vi "Eye tracker_4.2.vi"() -> ()   [LabVIEW 2013]
doc: "made for mouse gaze expt. Version 3"
uses:
  <vilib>/vision/Avi1.llb/AviRefnum.ctl
  <vilib>/vision/Image Controls.llb/IMAQ Image.ctl
  <vilib>/Platform/TimedLoop/XDataNode/timing_clust.ctl
  <vilib>/Platform/TimedLoop/XDataNode/nitl_modes.ctl
  <vilib>/Platform/TimedLoop/XDataNode/wakeup.ctl
  <vilib>/Analysis/baseanly.llb/Mean (DBL).vi
  Eye tracking dependencies/Global 1.vi
  <vilib>/DAQmx/create/channels.llb/DAQmx Create Channel (CO-Pulse Generation-Frequency).vi
  <vilib>/DAQmx/configure/timing.llb/DAQmx Timing (Implicit).vi
  <vilib>/Utility/inputDevices.llb/closeMouse.vi
  <vilib>/Utility/inputDevices.llb/mouseAcquire.vi
  <vilib>/platform/TimedLoop/XDataNode/XDataNode.xnode
  <vilib>/vision/NI_Vision_Development_Module.lvlib
  <vilib>/Platform/TimedLoop/XDataNode/XDNodeRunTimeDep.lvlib
  <vilib>/Analysis/NI_AALBase.lvlib
panel:
  out "Camera ready RTNET":bool
  out "processed frames":i32=12126
  out "param file path":path=path "D:/Satoru/Documents/LabVIEW Data/Saccade suppression project/Eye tracking dependencies/parameters for Eye tracker.txt"
  out "aquired frames":u64=12126
  out "Last Valid Buffer":i32=4318
  in  "duty cylcle of the pulses":dbl=0.5
  out "# of pulses":i32
  out "error IO":errorcluster
  in  "ver":string="3"
  out "saving disk":string="F:\\Eye_tracker_Data3\\"
  out "Info String":string="valid file name"
  out "error flag":errorcluster
  out "eye refnum out":refnum<file>
  in  "Gain offset":dbl min=-10.0 max=10.0 step=0.1
  in  "use % thresh":bool
  in  "Points to show":enum16{"All points", "Fit points"}(ring)
  in  "P Right":i32=237 min=0 max=320 step=5
  in  "P Bottom":i32=187 min=0 max=240 step=5
  in  "P Left":i32=108 min=0 max=320 step=5
  in  "P Top":i32=90 min=0 max=240 step=5
  in  "P Fit type":enum16{"Circle", "Ellipse"}(ring)=enum."Ellipse"
  in  "P Subsampling":i32=2
  in  "P Direction to keep":enum16{"Above", "Below"}(ring)=enum."Below"
  in  "P Threshold":u8=90
  in  "file subname":string="test"
  in  "Eye Y offset(deg)":dbl
  out "calib para":T1={"slope_Rp"=-0.158875, "intercept_Rp"=1.006881, "average_Rp"=0.92245, "slope_Rp0s"=-0.125099, "intercept_Rp0s"=1.099699, "average_Rp0s"=1.033217, "Y correction (pixel,P-CR Y)"=-9.268179}
  out "average_Rp0s":dbl=1.033217 format="%0.2f"
  out "R-squared_Rp0s":dbl=0.136529 format="%0.2f"
  out "intercept_Rp0s":dbl=1.099699 format="%0.2f"
  out "slope_Rp0s":dbl=-0.125099 format="%0.2f"
  out "slope_Rp":dbl=-0.158875 format="%0.2f"
  out "intercept_Rp":dbl=1.006881 format="%0.2f"
  out "R-squared_Rp":dbl=0.186582 format="%0.2f"
  out "average_Rp":dbl=0.92245 format="%0.2f"
  out "Rp0s":dbl[](array[numeric])=[1.0039530251172462, 0.99092677428564, 0.9947124694308508, 0.91502715314781, 0.9309803093450226, 0.9217648889080421, 0.9419782161135387, 0.41862170883477745, 1.0171231935751164, 1.0055084222134438, 0.9877063931309743, 0.9965106512655807, 1.0044842853477027, 1.0208232955492513, 0.3759308138742579, 0.9922053798543352, 0.9837769455073831, 1.0906382792092393, 1.0404579348655312, 1.0380768060657999, 0.7651629263639542, 0.9942213575350989, 0.9175234235218281, 0.9692162880521514, 0.9785182040001951, 0.9925018928857751, 1.0118623499027188, 0.987701680921089, 0.9820974709148313, 0.9777636459363701, 0.996026118758922, 0.9978612450714602, 1.0057534405553457, 1.002758388150481, 1.0281377557537945, 0.9995175172174519, 1.0172882695205345, 0.9728176754414147, 0.9567541016151462, 0.9881969134208142, 0.9994817859973143, 0.937125056422465, 0.9712908288207139, 1.0043446841247143, 1.2083670139927292, 1.510991890895332, 0.9895877539387384, 1.0042622767782914, 1.019202247794033, 0.977553264609903, 0.994725760374644, 1.019400802873885, 1.334253570427072, 0.9352478253803249, 0.956119013286909, 0.9758901683111171, 0.9779851768159086, 1.0516777655254512, 0.778039137219539, 1.1531230503845833, 1.0046625233826771, 0.9901398342766586, 1.011163664944152, 0.9938975966142147, 0.6154945551221118, 1.0077384474948252, 0.9896589896861816, 0.9972982423508683, 0.6853268629838346, 0.9658925865003825, 0.9626225998838313, 1.0096874472713344, 1.0358515198060945, 1.0544730519999652, 1.0617108224193677, 1.0142433944577367, 1.0418591984643595, 1.019211033782866, 1.0450176088988177, 1.0464926937167767, 1.1283816882695141, 1.030013176033189, 1.0427307654804812, 1.0441392816021982, 1.0538940244491395, 1.0462542279584326, 1.0781380078152705, 0.9990695213505404, 1.0272273014788156, 1.0262064169141834, 0.4857640606302865, 1.5639567502437777, 0.8687438257698011, 0.9864671983220689, 1.0593826663266908, 1.077023826126648, 1.0593759395811841, 1.0778741239177942]
  out "Diameters":dbl[](array[numeric])=[0.4171123023396653, 0.41706153689125236, 0.44082198235372194, 0.5954203122934263, 0.5513970359660245, 0.4888545273412629, 0.4723633211125596, 0.6187264429619335, 0.4791395781041599, 0.47868971473218613, 0.4607929067005807, 0.4175941622450629, 0.4072745719163012, 0.40955932983558824, 0.4735723248260562, 0.44999914869512314, 0.495476167758055, 0.5199527975917938, 0.4888346729487987, 0.4452820985792543, 0.6301036042248925, 0.4469040074392198, 0.3829612562912073, 0.4107677254295738, 0.40124095377797425, 0.383476616742587, 0.3832933211731289, 0.43509323930099303, 0.4004105804184655, 0.4216375686518822, 0.45690852528210607, 0.4082721732536112, 0.45028685912440625, 0.3918383679660448, 0.3652661041731884, 0.3475647461563056, 0.4095548614857446, 0.6482149714983727, 0.5034836724573097, 0.4455174223358519, 0.4486765714162201, 0.5064000813046842, 0.49521426028650833, 0.44577031309198606, 0.45147318540007164, 0.4761169863513808, 0.43800992027731955, 0.4015153245290642, 0.39091576046128906, 0.379195166874867, 0.38301812558069126, 0.35970454061703483, 0.42529628662735336, 0.42838925138004624, 0.3826964399461055, 0.3606217495513988, 0.3686694627564316, 0.36628712709457356, 0.5276402515437981, 0.5027800799946363, 0.5917418979942912, 0.4405882646486038, 0.3855160638859669, 0.3520620038697737, 0.4917921769667696, 0.39313264413588306, 0.3962868259759099, 0.3692702539594129, 0.43066029115997034, 0.5289298666466735, 0.4857116713496977, 0.3808981023756301, 0.37251109381109737, 0.3648554945721928, 0.3719954884814041, 0.3714007266142857, 0.34155839352729517, 0.3379878486536885, 0.34158014089555133, 0.3883397541343963, 0.3779925489446427, 0.3350578969183736, 0.3364315822035769, 0.32799683082239195, 0.30857349620419, 0.3354342336706663, 0.2996572825051776, 0.3530772896636659, 0.31517664347717034, 0.3170963264045597, 0.44637289830791427, 0.37272436153500477, 0.3543878411074852, 0.46493263060229995, 0.31309427627625497, 0.39133764775033814, 0.3896143560981249, 0.34679282192506145]
  out "Rp":dbl[](array[numeric])=[0.939777828488882, 0.9243782721008702, 0.9247867300831337, 0.8546428244499522, 0.8722515142500874, 0.8599558310217699, 0.8821886686394919, 0.27768529551706517, 0.9621621967506099, 0.9489706433656064, 0.9286039576834555, 0.9360718380299038, 0.9427832164989408, 0.9580355580333006, 0.18594170348233657, 0.9408721482456565, 0.9298677620512195, 1.03645888355633, 0.9826129548661878, 0.9795606095219592, 0.6946292066688117, 0.9414788639375723, 0.8576339811674867, 0.9130407361980429, 0.9228386688426881, 0.9350370985090772, 0.95317668634537, 0.9265514452452699, 0.9183790967298439, 0.9138737325811144, 0.9315397662213876, 0.9334204076293418, 0.9423909994254046, 0.9378626398245973, 0.9648383077501701, 0.9338531100959763, 0.9531838316474268, 0.9307945475016182, 0.8970066818718861, 0.9280567210488938, 0.9374342077923953, 0.8791518280424994, 0.9236246067129958, 0.9511138467128057, 1.1666245999199012, 1.4802034620448514, 0.9412071610357354, 0.95348691386894, 0.9657397985521751, 0.9190931489538748, 0.9348033445576653, 0.9599667294264533, 1.2900914874489557, 0.8774362961435918, 0.896842734172207, 0.9171822481686075, 0.9164350407661369, 0.9903031524940573, 0.7074385526832087, 1.1067447532230492, 0.9610074838402222, 0.943528766665827, 0.958930447804304, 0.9386499872173812, 0.5144779715413748, 0.9513120067327815, 0.9306395174738417, 0.9365203104014679, 0.5902231328371776, 0.9026704048492892, 0.8933039465724875, 0.9465112185353972, 0.9722657096813544, 0.9903344550575592, 0.9978061383235594, 0.9432972456213076, 0.9754521620179915, 0.9527832237284578, 0.979250668089585, 0.9810855558397411, 1.084116178214518, 0.9823792672041992, 0.9927448850260591, 0.9912403488728432, 0.9999505174357944, 0.9893853300714827, 1.0226328706112693, 0.9508934971805839, 0.9756310457714327, 0.9724214165590328, 0.3641279840331179, 1.5306845012262937, 0.802628109680344, 0.9346469119852467, 1.00312473762936, 1.0121118529364288, 0.994327011204879, 1.0147111135607931]
  out "calib data":dbl[][][](array[numeric])
  out "Frame Rate":cluster{i32, "camera FR":i32}={200, "camera FR"=200}
  out "Frame Buffers Out":T2[](array[typedef])=[refnum, refnum, refnum, refnum, refnum, refnum, refnum, refnum, refnum, refnum, refnum, refnum, refnum, refnum, refnum, refnum, refnum, refnum, refnum, refnum, refnum, refnum, refnum, refnum, refnum, refnum, refnum, refnum, refnum, refnum, refnum, refnum, refnum, refnum, refnum, refnum, refnum, refnum, refnum, refnum, refnum, refnum, refnum, refnum, refnum, refnum, refnum, refnum, refnum, refnum, refnum, refnum, refnum, refnum, refnum, refnum, refnum, refnum, refnum, refnum, refnum, refnum, refnum, refnum, refnum, refnum, refnum, refnum, refnum, refnum, refnum, refnum, refnum, refnum, refnum, refnum, refnum, refnum, refnum, refnum, refnum, refnum, refnum, refnum, refnum, refnum, refnum, refnum, refnum, refnum, refnum, refnum, refnum, refnum, refnum, refnum, refnum, refnum, refnum, refnum, refnum, refnum, refnum, refnum, refnum, refnum, refnum, refnum, refnum, refnum, refnum, refnum, refnum, refnum, refnum, refnum, refnum, refnum, refnum, refnum, refnum, refnum, refnum, refnum, refnum, refnum, refnum, refnum, refnum, refnum, refnum, refnum, refnum, refnum, refnum, refnum, refnum, refnum, refnum, refnum, refnum, refnum, refnum, refnum, refnum, refnum, refnum, refnum, refnum, refnum, refnum, refnum, refnum, refnum, refnum, refnum, refnum, refnum, refnum, refnum, refnum, refnum, refnum, refnum, refnum, refnum, refnum, refnum, refnum, refnum, refnum, refnum, refnum, refnum, refnum, refnum, refnum, refnum, refnum, refnum, refnum, refnum, refnum, refnum, refnum, refnum, refnum, refnum, refnum, refnum, refnum, refnum, refnum, refnum, refnum, refnum, refnum, refnum, refnum, refnum, refnum, refnum, refnum, refnum, refnum, refnum, refnum, refnum, refnum, refnum, refnum, refnum, refnum, refnum, refnum, refnum, refnum, refnum, refnum, refnum, refnum, refnum, refnum, refnum, refnum, refnum, refnum, refnum, refnum, refnum, refnum, refnum, refnum, refnum, refnum, refnum, refnum, refnum, refnum, refnum, refnum, refnum, refnum, refnum, "LL Ring num 244", "LL Ring num 245", "LL Ring num 246", "LL Ring num 247", "LL Ring num 248", "LL Ring num 249", "LL Ring num 250", "LL Ring num 251", "LL Ring num 252", "LL Ring num 253", "LL Ring num 254", "LL Ring num 255", "LL Ring num 256", "LL Ring num 257", "LL Ring num 258", "LL Ring num 259", "LL Ring num 260", "LL Ring num 261", "LL Ring num 262", "LL Ring num 263", "LL Ring num 264", "LL Ring num 265", "LL Ring num 266", "LL Ring num 267", "LL Ring num 268", "LL Ring num 269", "LL Ring num 270", "LL Ring num 271", "LL Ring num 272", "LL Ring num 273", "LL Ring num 274", "LL Ring num 275", "LL Ring num 276", "LL Ring num 277", "LL Ring num 278", "LL Ring num 279", "LL Ring num 280", "LL Ring num 281", "LL Ring num 282", "LL Ring num 283", "LL Ring num 284", "LL Ring num 285", "LL Ring num 286", "LL Ring num 287", "LL Ring num 288", "LL Ring num 289", "LL Ring num 290", "LL Ring num 291", "LL Ring num 292", "LL Ring num 293", "LL Ring num 294", "LL Ring num 295", "LL Ring num 296", "LL Ring num 297", "LL Ring num 298", "LL Ring num 299", "LL Ring num 300", "LL Ring num 301", "LL Ring num 302", "LL Ring num 303", "LL Ring num 304", "LL Ring num 305", "LL Ring num 306", "LL Ring num 307", "LL Ring num 308", "LL Ring num 309", "LL Ring num 310", "LL Ring num 311", "LL Ring num 312", "LL Ring num 313", "LL Ring num 314", "LL Ring num 315", "LL Ring num 316", "LL Ring num 317", "LL Ring num 318", "LL Ring num 319", "LL Ring num 320", "LL Ring num 321", "LL Ring num 322", "LL Ring num 323", "LL Ring num 324", "LL Ring num 325", "LL Ring num 326", "LL Ring num 327", "LL Ring num 328", "LL Ring num 329", "LL Ring num 330", "LL Ring num 331", "LL Ring num 332", "LL Ring num 333", "LL Ring num 334", "LL Ring num 335", "LL Ring num 336", "LL Ring num 337", "LL Ring num 338", "LL Ring num 339", "LL Ring num 340", "LL Ring num 341", "LL Ring num 342", "LL Ring num 343", "LL Ring num 344", "LL Ring num 345", "LL Ring num 346", "LL Ring num 347", "LL Ring num 348", "LL Ring num 349", "LL Ring num 350", "LL Ring num 351", "LL Ring num 352", "LL Ring num 353", "LL Ring num 354", "LL Ring num 355", "LL Ring num 356", "LL Ring num 357", "LL Ring num 358", "LL Ring num 359", "LL Ring num 360", "LL Ring num 361", "LL Ring num 362", "LL Ring num 363", "LL Ring num 364", "LL Ring num 365", "LL Ring num 366", "LL Ring num 367", "LL Ring num 368", "LL Ring num 369", "LL Ring num 370", "LL Ring num 371", "LL Ring num 372", "LL Ring num 373", "LL Ring num 374", "LL Ring num 375", "LL Ring num 376", "LL Ring num 377", "LL Ring num 378", "LL Ring num 379", "LL Ring num 380", "LL Ring num 381", "LL Ring num 382", "LL Ring num 383", "LL Ring num 384", "LL Ring num 385", "LL Ring num 386", "LL Ring num 387", "LL Ring num 388", "LL Ring num 389", "LL Ring num 390", "LL Ring num 391", "LL Ring num 392", "LL Ring num 393", "LL Ring num 394", "LL Ring num 395", "LL Ring num 396", "LL Ring num 397", "LL Ring num 398", "LL Ring num 399", "LL Ring num 400", "LL Ring num 401", "LL Ring num 402", "LL Ring num 403", "LL Ring num 404", "LL Ring num 405", "LL Ring num 406", "LL Ring num 407", "LL Ring num 408", "LL Ring num 409", "LL Ring num 410", "LL Ring num 411", "LL Ring num 412", "LL Ring num 413", "LL Ring num 414", "LL Ring num 415", "LL Ring num 416", "LL Ring num 417", "LL Ring num 418", "LL Ring num 419", "LL Ring num 420", "LL Ring num 421", "LL Ring num 422", "LL Ring num 423", "LL Ring num 424", "LL Ring num 425", "LL Ring num 426", "LL Ring num 427", "LL Ring num 428", "LL Ring num 429", "LL Ring num 430", "LL Ring num 431", "LL Ring num 432", "LL Ring num 433", "LL Ring num 434", "LL Ring num 435", "LL Ring num 436", "LL Ring num 437", "LL Ring num 438", "LL Ring num 439", "LL Ring num 440", "LL Ring num 441", "LL Ring num 442", "LL Ring num 443", "LL Ring num 444", "LL Ring num 445", "LL Ring num 446", "LL Ring num 447", "LL Ring num 448", "LL Ring num 449", "LL Ring num 450", "LL Ring num 451", "LL Ring num 452", "LL Ring num 453", "LL Ring num 454", "LL Ring num 455", "LL Ring num 456", "LL Ring num 457", "LL Ring num 458", "LL Ring num 459", "LL Ring num 460", "LL Ring num 461", "LL Ring num 462", "LL Ring num 463", "LL Ring num 464", "LL Ring num 465", "LL Ring num 466", "LL Ring num 467", "LL Ring num 468", "LL Ring num 469", "LL Ring num 470", "LL Ring num 471", "LL Ring num 472", "LL Ring num 473", "LL Ring num 474", "LL Ring num 475", "LL Ring num 476", "LL Ring num 477", "LL Ring num 478", "LL Ring num 479", "LL Ring num 480", "LL Ring num 481", "LL Ring num 482", "LL Ring num 483", "LL Ring num 484", "LL Ring num 485", "LL Ring num 486", "LL Ring num 487", "LL Ring num 488", "LL Ring num 489", "LL Ring num 490", "LL Ring num 491", "LL Ring num 492", "LL Ring num 493", "LL Ring num 494", "LL Ring num 495", "LL Ring num 496", "LL Ring num 497", "LL Ring num 498", "LL Ring num 499"]
  out "Avi Refnum":T3
  in  "tasks":T4(tab)
  in  "Disp trace Divisor":i32=25 min=1 step=1
  in  "Disp Frame Divisor":i32=25 min=1 step=1
  in  "Save Movie? 2":bool
  in  "Cam FR (f/s)":i32=200 min=2 max=3000 step=1
  in  "Save Frame Divisor":i32=1 min=1 step=1
  in  "Gain (dB)":dbl(slide)=26.8032 min=6.0 max=39.5 step=0.0352 scale=6.0..40.0
  in  "Pixel value offset":cluster{"Ch 1":u8, "Ch 2":u8} {"Ch 2" step=1; "Ch 1" step=1}
  in  "Zoom":i32=2 min=1 step=1
  in  "Region of interest":i32[](array[numeric])
  in  "resolution":cluster{"width":u16, "height":u16}={"width"=320, "height"=240}
  out "Image Histogram":T5(graph)={"Starting Value"=0.0, "Incremental Value"=1.0, "Histogram"=[0, 0, 0, 0, 0, 0, 0, 0, 0, 0, 0, 0, 0, 0, 0, 0, 0, 0, 0, 0, 0, 0, 0, 0, 0, 0, 0, 0, 0, 0, 0, 0, 0, 0, 0, 0, 0, 0, 1, 0, 2, 1, 2, 0, 2, 5, 8, 9, 18, 23, 34, 49, 54, 74, 101, 111, 113, 126, 172, 183, 141, 158, 148, 135, 127, 122, 91, 85, 65, 46, 46, 43, 40, 39, 43, 48, 65, 47, 64, 67, 91, 83, 84, 79, 92, 128, 112, 149, 146, 162, 194, 158, 185, 221, 216, 248, 195, 235, 264, 290, 305, 364, 334, 349, 350, 401, 397, 418, 398, 463, 458, 492, 462, 444, 529, 514, 538, 509, 522, 584, 568, 532, 583, 588, 592, 524, 582, 558, 618, 623, 630, 632, 648, 649, 663, 659, 686, 600, 694, 632, 583, 621, 634, 597, 560, 534, 594, 608, 627, 668, 723, 649, 721, 661, 767, 727, 738, 779, 744, 716, 773, 730, 722, 722, 744, 741, 717, 726, 734, 718, 658, 672, 715, 706, 700, 651, 599, 659, 582, 573, 572, 475, 531, 552, 484, 442, 423, 410, 432, 389, 400, 410, 402, 399, 387, 426, 425, 434, 407, 413, 438, 473, 437, 439, 395, 440, 395, 382, 389, 401, 409, 339, 342, 316, 301, 326, 265, 255, 273, 254, 261, 232, 228, 217, 234, 230, 169, 192, 206, 164, 201, 170, 181, 178, 136, 161, 156, 156, 140, 132, 116, 121, 112, 106, 94, 88, 109, 79, 85, 75, 82, 94, 55, 101, 99, 1333]}
  out "file or folder exists? 4":bool
  in  "stop free run":bool
  in  "counter":tag="Dev1/ctr0"
  in  "Cam FR (f/s) 2":i32=200 min=2 max=3000 step=1
  out "frames captured":u64=39600
  in  "Change pupil size?":bool=TRUE
  in  "1D or 2D cal?":bool=TRUE
  in  "L/R?":bool=TRUE
  in  "clip time(s)":sgl=1.0
  in  "stop calib":bool
  out "counter finished":sgl=88.0 format="%#.1f"
  out "Y correction (pixel,P-CR Y)":dbl=-9.268179
  out "frames/clip":i32=200
  out "conversion factor":cluster{"x":dbl, "y":dbl}={"x"=0.01556420233463035, "y"=0.015463917525773196} {"y" format="%#_9g"; "x" format="%#_9g"}
  out "Rp vs Pupil":cluster{dbl[], dbl[]}[](graph)=[{[0.4171123023396653, 0.41706153689125236, 0.44082198235372194, 0.5954203122934263, 0.5513970359660245, 0.4723633211125596, 0.4607929067005807, 0.4175941622450629, 0.4072745719163012, 0.40955932983558824, 0.44999914869512314, 0.495476167758055, 0.4469040074392198, 0.4107677254295738, 0.40124095377797425, 0.383476616742587, 0.3832933211731289, 0.43509323930099303, 0.4004105804184655, 0.4216375686518822, 0.45690852528210607, 0.4082721732536112, 0.45028685912440625, 0.3918383679660448, 0.3652661041731884, 0.4095548614857446, 0.5034836724573097, 0.4455174223358519, 0.4486765714162201, 0.5064000813046842, 0.49521426028650833, 0.44577031309198606, 0.43800992027731955, 0.4015153245290642, 0.39091576046128906, 0.38301812558069126, 0.35970454061703483, 0.36628712709457356, 0.4405882646486038, 0.3855160638859669, 0.3520620038697737, 0.39313264413588306, 0.3962868259759099, 0.3692702539594129, 0.5289298666466735, 0.4857116713496977, 0.3808981023756301, 0.37251109381109737, 0.3648554945721928, 0.3714007266142857, 0.34155839352729517, 0.3379878486536885, 0.34158014089555133, 0.3883397541343963, 0.3350578969183736, 0.3364315822035769, 0.32799683082239195, 0.30857349620419, 0.3354342336706663, 0.2996572825051776, 0.3530772896636659, 0.31517664347717034, 0.3170963264045597, 0.46493263060229995, 0.31309427627625497], [0.939777828488882, 0.9243782721008702, 0.9247867300831337, 0.8546428244499522, 0.8722515142500874, 0.8821886686394919, 0.9286039576834555, 0.9360718380299038, 0.9427832164989408, 0.9580355580333006, 0.9408721482456565, 0.9298677620512195, 0.9414788639375723, 0.9130407361980429, 0.9228386688426881, 0.9350370985090772, 0.95317668634537, 0.9265514452452699, 0.9183790967298439, 0.9138737325811144, 0.9315397662213876, 0.9334204076293418, 0.9423909994254046, 0.9378626398245973, 0.9648383077501701, 0.9531838316474268, 0.8970066818718861, 0.9280567210488938, 0.9374342077923953, 0.8791518280424994, 0.9236246067129958, 0.9511138467128057, 0.9412071610357354, 0.95348691386894, 0.9657397985521751, 0.9348033445576653, 0.9599667294264533, 0.9903031524940573, 0.943528766665827, 0.958930447804304, 0.9386499872173812, 0.9513120067327815, 0.9306395174738417, 0.9365203104014679, 0.9026704048492892, 0.8933039465724875, 0.9465112185353972, 0.9722657096813544, 0.9903344550575592, 0.9432972456213076, 0.9754521620179915, 0.9527832237284578, 0.979250668089585, 0.9810855558397411, 0.9823792672041992, 0.9927448850260591, 0.9912403488728432, 0.9999505174357944, 0.9893853300714827, 1.0226328706112693, 0.9508934971805839, 0.9756310457714327, 0.9724214165590328, 0.9346469119852467, 1.00312473762936]}, {[0.4171123023396653, 0.41706153689125236, 0.44082198235372194, 0.5954203122934263, 0.5513970359660245, 0.4723633211125596, 0.4607929067005807, 0.4175941622450629, 0.4072745719163012, 0.40955932983558824, 0.44999914869512314, 0.495476167758055, 0.4469040074392198, 0.4107677254295738, 0.40124095377797425, 0.383476616742587, 0.3832933211731289, 0.43509323930099303, 0.4004105804184655, 0.4216375686518822, 0.45690852528210607, 0.4082721732536112, 0.45028685912440625, 0.3918383679660448, 0.3652661041731884, 0.4095548614857446, 0.5034836724573097, 0.4455174223358519, 0.4486765714162201, 0.5064000813046842, 0.49521426028650833, 0.44577031309198606, 0.43800992027731955, 0.4015153245290642, 0.39091576046128906, 0.38301812558069126, 0.35970454061703483, 0.36628712709457356, 0.4405882646486038, 0.3855160638859669, 0.3520620038697737, 0.39313264413588306, 0.3962868259759099, 0.3692702539594129, 0.5289298666466735, 0.4857116713496977, 0.3808981023756301, 0.37251109381109737, 0.3648554945721928, 0.3714007266142857, 0.34155839352729517, 0.3379878486536885, 0.34158014089555133, 0.3883397541343963, 0.3350578969183736, 0.3364315822035769, 0.32799683082239195, 0.30857349620419, 0.3354342336706663, 0.2996572825051776, 0.3530772896636659, 0.31517664347717034, 0.3170963264045597, 0.46493263060229995, 0.31309427627625497], [0.9398873587415357, 0.9399102647487777, 0.929189253650656, 0.8594325475462748, 0.87929640215402, 0.9149574058758638, 0.9201781220243312, 0.9396699375066659, 0.9443262661355832, 0.9432953546971639, 0.9250484010580191, 0.9045285994889237, 0.9264449676252247, 0.9427501114442752, 0.9470487103391233, 0.9550642020860263, 0.9551469073466453, 0.9317741343905228, 0.9474233852170393, 0.9378455018061569, 0.9219308036549254, 0.9438761358959925, 0.9249185825026279, 0.9512912750250406, 0.9632810138317232, 0.9432973708726745, 0.9009155129041384, 0.927070612220364, 0.9256451645196992, 0.8995995926420899, 0.9046467754260529, 0.9269565047383553, 0.930458091340477, 0.9469249108138964, 0.9517075671064884, 0.955271079050637, 0.9657904610852527, 0.9628203154795438, 0.9292947100114956, 0.9541439779474367, 0.9692388695511045, 0.9507072813788446, 0.9492840749593423, 0.9614742912109515, 0.8894338708305484, 0.9089344627765849, 0.956227660119188, 0.9600119836093526, 0.9634662860353198, 0.9605129952195437, 0.9739782303189793, 0.9755893049630445, 0.9739684176335733, 0.9528698934805067, 0.9769113359460448, 0.9762915119107062, 0.9800973775587395, 0.9888614298292744, 0.97674152808178, 0.9928845373156776, 0.9687807598628296, 0.9858820069347005, 0.9850158219129624, 0.918310226661696, 0.9868215971417378]}, {[0.37272436153500477, 0.44637289830791427, 0.43066029115997034, 0.4917921769667696, 0.42529628662735336, 0.4761169863513808, 0.4735723248260562, 0.6187264429619335, 0.3543878411074852, 0.3779925489446427, 0.5027800799946363, 0.5276402515437981, 0.45147318540007164, 0.6301036042248925, 0.5199527975917938, 0.39133764775033814, 0.5917418979942912, 0.42838925138004624, 0.3829612562912073, 0.4888346729487987, 0.3826964399461055, 0.6482149714983727, 0.4888545273412629, 0.3686694627564316, 0.3606217495513988, 0.4452820985792543, 0.4791395781041599, 0.34679282192506145, 0.3896143560981249, 0.3719954884814041, 0.379195166874867, 0.3475647461563056, 0.47868971473218613], [1.5306845012262937, 0.3641279840331179, 0.5902231328371776, 0.5144779715413748, 1.2900914874489557, 1.4802034620448514, 0.18594170348233657, 0.27768529551706517, 0.802628109680344, 1.084116178214518, 1.1067447532230492, 0.7074385526832087, 1.1666245999199012, 0.6946292066688117, 1.03645888355633, 1.0121118529364288, 0.9610074838402222, 0.8774362961435918, 0.8576339811674867, 0.9826129548661878, 0.896842734172207, 0.9307945475016182, 0.8599558310217699, 0.9164350407661369, 0.9171822481686075, 0.9795606095219592, 0.9621621967506099, 1.0147111135607931, 0.994327011204879, 0.9978061383235594, 0.9190931489538748, 0.9338531100959763, 0.9489706433656064]}]
  out "Rp0s vs Pupil":cluster{dbl[], dbl[]}[](graph)=[{[0.4171123023396653, 0.41706153689125236, 0.44082198235372194, 0.5954203122934263, 0.5513970359660245, 0.4607929067005807, 0.4175941622450629, 0.4072745719163012, 0.40955932983558824, 0.44999914869512314, 0.495476167758055, 0.4469040074392198, 0.40124095377797425, 0.383476616742587, 0.3832933211731289, 0.43509323930099303, 0.4004105804184655, 0.4216375686518822, 0.45690852528210607, 0.4082721732536112, 0.45028685912440625, 0.3918383679660448, 0.3652661041731884, 0.3475647461563056, 0.4095548614857446, 0.5034836724573097, 0.4455174223358519, 0.4486765714162201, 0.5064000813046842, 0.49521426028650833, 0.44577031309198606, 0.43800992027731955, 0.4015153245290642, 0.39091576046128906, 0.38301812558069126, 0.35970454061703483, 0.4405882646486038, 0.3855160638859669, 0.39313264413588306, 0.3962868259759099, 0.3692702539594129, 0.5289298666466735, 0.4857116713496977, 0.3808981023756301, 0.37251109381109737, 0.3714007266142857, 0.34155839352729517, 0.3379878486536885, 0.34158014089555133, 0.3350578969183736, 0.3364315822035769, 0.32799683082239195, 0.30857349620419, 0.3354342336706663, 0.3530772896636659, 0.31517664347717034, 0.3170963264045597, 0.46493263060229995, 0.31309427627625497], [1.0039530251172462, 0.99092677428564, 0.9947124694308508, 0.91502715314781, 0.9309803093450226, 0.9877063931309743, 0.9965106512655807, 1.0044842853477027, 1.0208232955492513, 0.9922053798543352, 0.9837769455073831, 0.9942213575350989, 0.9785182040001951, 0.9925018928857751, 1.0118623499027188, 0.987701680921089, 0.9820974709148313, 0.9777636459363701, 0.996026118758922, 0.9978612450714602, 1.0057534405553457, 1.002758388150481, 1.0281377557537945, 0.9995175172174519, 1.0172882695205345, 0.9567541016151462, 0.9881969134208142, 0.9994817859973143, 0.937125056422465, 0.9712908288207139, 1.0043446841247143, 0.9895877539387384, 1.0042622767782914, 1.019202247794033, 0.994725760374644, 1.019400802873885, 0.9901398342766586, 1.011163664944152, 1.0077384474948252, 0.9896589896861816, 0.9972982423508683, 0.9658925865003825, 0.9626225998838313, 1.0096874472713344, 1.0358515198060945, 1.0142433944577367, 1.0418591984643595, 1.019211033782866, 1.0450176088988177, 1.030013176033189, 1.0427307654804812, 1.0441392816021982, 1.0538940244491395, 1.0462542279584326, 0.9990695213505404, 1.0272273014788156, 1.0262064169141834, 0.9864671983220689, 1.0593826663266908]}, {[0.4171123023396653, 0.41706153689125236, 0.44082198235372194, 0.5954203122934263, 0.5513970359660245, 0.4607929067005807, 0.4175941622450629, 0.4072745719163012, 0.40955932983558824, 0.44999914869512314, 0.495476167758055, 0.4469040074392198, 0.40124095377797425, 0.383476616742587, 0.3832933211731289, 0.43509323930099303, 0.4004105804184655, 0.4216375686518822, 0.45690852528210607, 0.4082721732536112, 0.45028685912440625, 0.3918383679660448, 0.3652661041731884, 0.3475647461563056, 0.4095548614857446, 0.5034836724573097, 0.4455174223358519, 0.4486765714162201, 0.5064000813046842, 0.49521426028650833, 0.44577031309198606, 0.43800992027731955, 0.4015153245290642, 0.39091576046128906, 0.38301812558069126, 0.35970454061703483, 0.4405882646486038, 0.3855160638859669, 0.39313264413588306, 0.3962868259759099, 0.3692702539594129, 0.5289298666466735, 0.4857116713496977, 0.3808981023756301, 0.37251109381109737, 0.3714007266142857, 0.34155839352729517, 0.3379878486536885, 0.34158014089555133, 0.3350578969183736, 0.3364315822035769, 0.32799683082239195, 0.30857349620419, 0.3354342336706663, 0.3530772896636659, 0.31517664347717034, 0.3170963264045597, 0.46493263060229995, 0.31309427627625497], [0.9981520309879384, 0.9981725860034583, 0.9885519416378736, 0.925954817597733, 0.943779916290549, 0.9804656807511994, 0.9979569251010901, 1.0021353445969856, 1.0012102422693532, 0.9848360915375929, 0.966422369963961, 0.9860893194424033, 1.004578366738059, 1.0117711767077961, 1.0118453933924256, 0.9908715193435683, 1.004914586309157, 0.9963197430403843, 0.9820384733264252, 1.0017314141361677, 0.9847195971004504, 1.008385489561423, 1.0191446439023368, 1.0263119535614638, 1.0012120515117267, 0.963180117831569, 0.986650750084905, 0.9853716053042193, 0.9619992589798462, 0.9665284167400797, 0.9865483541920353, 0.9896905503063748, 1.004467273559073, 1.0087590548931966, 1.011956820551062, 1.0213965303484416, 0.9886465743301114, 1.0109454011262795, 1.0078614349614985, 1.0065843014247888, 1.0175233569133935, 0.9528769109687112, 0.9703760309970514, 1.0128152215155934, 1.0162111354018852, 1.016660724949043, 1.028743935851917, 1.03018965548182, 1.028735130305901, 1.0313759978716677, 1.030819790387256, 1.0342350354203798, 1.0420995763041199, 1.031223618487147, 1.0240799154156346, 1.0394259508576917, 1.0386486680088383, 0.9787894995746698, 1.0402691048427553]}, {[0.37272436153500477, 0.44637289830791427, 0.43066029115997034, 0.4917921769667696, 0.42529628662735336, 0.4761169863513808, 0.4735723248260562, 0.6187264429619335, 0.3543878411074852, 0.3779925489446427, 0.5027800799946363, 0.5276402515437981, 0.45147318540007164, 0.6301036042248925, 0.5199527975917938, 0.39133764775033814, 0.5917418979942912, 0.42838925138004624, 0.3829612562912073, 0.4888346729487987, 0.34679282192506145, 0.3896143560981249, 0.3826964399461055, 0.6482149714983727, 0.4888545273412629, 0.3719954884814041, 0.3606217495513988, 0.4452820985792543, 0.4791395781041599, 0.3883397541343963, 0.3686694627564316, 0.3648554945721928, 0.379195166874867, 0.47868971473218613, 0.4723633211125596, 0.2996572825051776, 0.3520620038697737, 0.36628712709457356, 0.4107677254295738], [1.5639567502437777, 0.4857640606302865, 0.6853268629838346, 0.6154945551221118, 1.334253570427072, 1.510991890895332, 0.3759308138742579, 0.41862170883477745, 0.8687438257698011, 1.1283816882695141, 1.1531230503845833, 0.778039137219539, 1.2083670139927292, 0.7651629263639542, 1.0906382792092393, 1.077023826126648, 1.0046625233826771, 0.9352478253803249, 0.9175234235218281, 1.0404579348655312, 1.0778741239177942, 1.0593759395811841, 0.956119013286909, 0.9728176754414147, 0.9217648889080421, 1.0617108224193677, 0.9758901683111171, 1.0380768060657999, 1.0171231935751164, 1.0464926937167767, 0.9779851768159086, 1.0544730519999652, 0.977553264609903, 1.0055084222134438, 0.9419782161135387, 1.0781380078152705, 0.9938975966142147, 1.0516777655254512, 0.9692162880521514]}]
  out "calib para file path":path=path "E:/Eye_tracker_Data2/cal/3cal083116_animal16-56.cal"
  in  "Save Movie? 3":bool
  in  "stop 2":bool
  in  "Outlier Cutoff_Rp(1D)":dbl=2.0
  in  "Outlier Cutoff_Rp0s(2D)":dbl=2.0
  out "Buffer Number":i32=39599
  in  "stop program":bool
  in  "End session and save":bool
  in  "Start session":bool
  out "file or folder exists?":bool
  out "Movie Directory":path=path "F:/Eye_tracker_Data3/avi/3mov013119_19-11_V1_flippingStripes.avi"
  in  "Save Movie?":bool
  out "data path":path=path "F:/Eye_tracker_Data3/eye/3trk013119_19-11_V1_flippingStripes.eye"
  in  "save eye data":bool
  out "file or folder exists? 3":bool
  in  "input cal para from file?":bool=TRUE
  in  "calib para file to load":path=path "E:/Eye_tracker_Data2/cal/3cal071717_17-48.cal"
  in  "Max expected duration of eye tracking per trial (ms)":i32=50000000
  in  "Time for eye tracking after VS (>1ms)":dbl=10.0 format="%#_13g"
  out "L Port data":u16=9094
  out "R Port data":u16=9095
  in  "talk to VS":bool=TRUE
  out "Remote IP_VS":string="192.168.137.3"
  out "L Port com":u16=9092
  out "R Port com":u16=9093
  out "Local IP_tracker":string="192.168.137.5"
  out "# in Q3":i32
  out "queue timed out? 3":bool
  out "# in Q2":i32
  out "# in Q1":i32
  out "queue timed out?":bool
  out "queue timed out? 2":bool
  out "Buffer Overrun":bool
  out "Vary pupil size?":bool=TRUE
  out "2D cal?":bool=TRUE
  out "Trial counter":u32=2
  out "frame/trial":i32=12126
  out "error out":errorcluster
  out "data path2":path=path "F:/Eye_tracker_Data3/eye/3trk013119_19-11_V1_flippingStripes.eye"
  out "move path2":path=path "F:/Eye_tracker_Data3/avi/3mov013119_19-11_V1_flippingStripes.avi"
  out "eye file exist":bool=TRUE
  out "avi file exist":bool
  in  "Display Overlay":bool=TRUE
  in  "Include Overlay to Movie?":bool
  out "eye trace":cluster{i32, dbl, "Data":dbl[][]}(graph)={0, 0.005, "Data"=array5x13000[65000 elements]}
  in  "CR Right":i32=185 min=0 max=320 step=5
  in  "CR Bottom":i32=175 min=0 max=240 step=5
  in  "CR Left":i32=150 min=0 max=320 step=5
  in  "CR Top":i32=130 min=0 max=240 step=5
  in  "CR Fit type":enum16{"Circle", "Ellipse"}(ring)
  in  "CR Subsampling":i32=1
  in  "CR Direction to keep":enum16{"Above", "Below"}(ring)
  in  "CR Threshold":u8=255
  out "Image":T2(plugin-control)
  # "Temporary items and other variables"
  # "Common settings"
  # "Pupil"
  # "Region of Interest"
  # "Fit Parameters"
  # "AVI FR"
  # "save or display portion of frames >=2"
  # "left          top         right       bottom"
  # "(mm/pixel)"
  # "Cornea Reflection"
  # "Region of Interest"
  # "Fit Parameters"
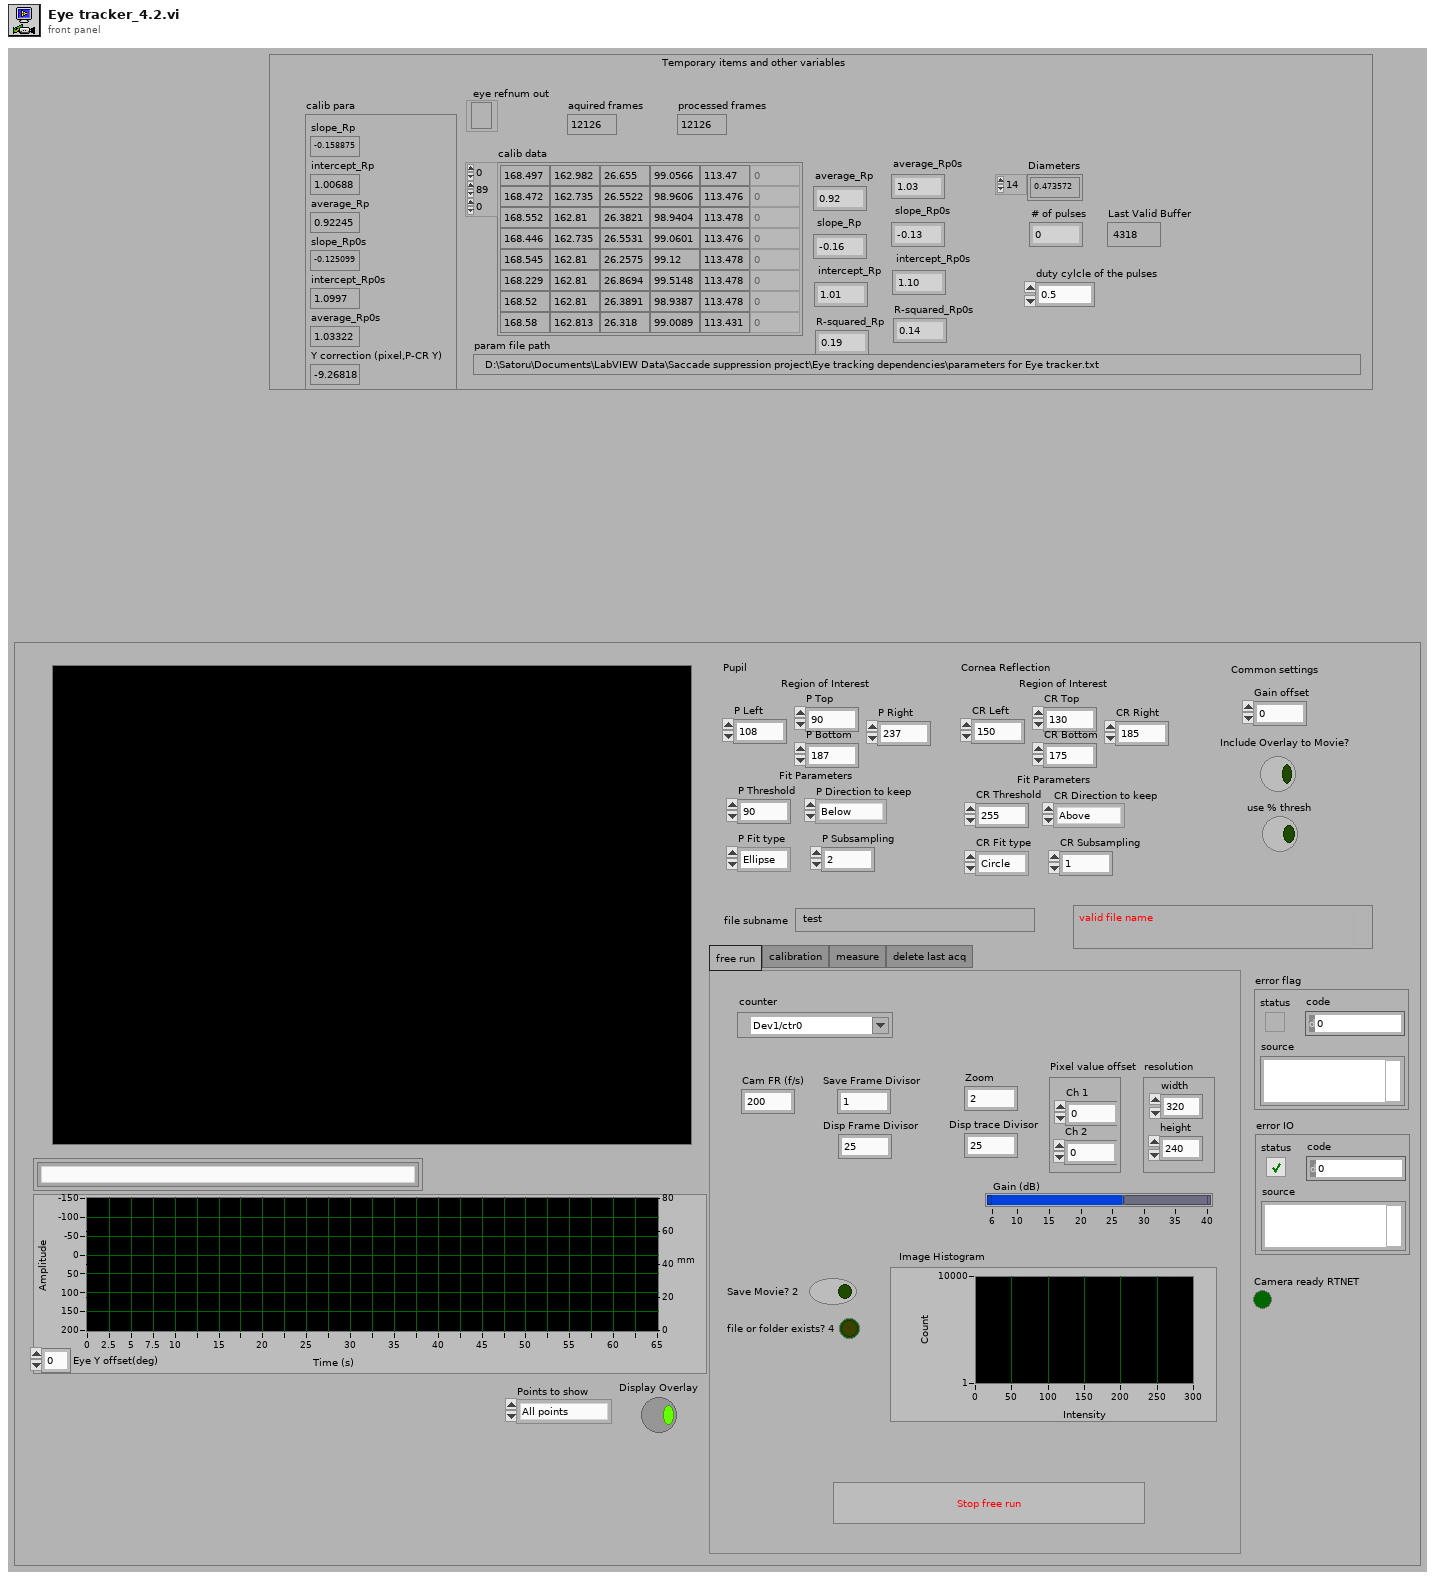
[diagram p1: front panel]
types:
  T1 = cluster{"slope_Rp":dbl, "intercept_Rp":dbl, "average_Rp":dbl, "slope_Rp0s":dbl, "intercept_Rp0s":dbl, "average_Rp0s":dbl, "Y correction (pixel,P-CR Y)":dbl}
  T2 = typedef "IMAQ Image.ctl" = refnum<image>
  T3 = typedef "AviRefnum.ctl" = refnum<k1>
  T4 = enum32{"free run", "calibration", "measure", "delete last acq"}
  T5 = cluster{"Starting Value":sgl, "Incremental Value":sgl, "Histogram":u32[]}
  T6 = enum8{"Enabled", "Disabled", "Disabled and Grayed Out"}
  T7 = enum16{"open", "replace", "create", "open or create", "replace or create", "replace or create with confirmation"}
  T8 = enum16{"big-endian, network order", "native, host order", "little-endian"}
  T9 = typedef "XDNodeRunTimeDep.lvlib/timing_clust.ctl" = cluster{"Expected End [f-1]":u64, "Actual End [f-1]":u64, "Finished Late? [f-1]":bool, "Expected End [i-1]":u64, "Actual End [i-1]":u64, "Finished Late? [i-1]":bool, "Expected Start [i]":u64, "Actual Start [i]":u64, "Expected Start [f]":u64, "Actual Start [f]":u64, "Source Name":string, "Structure Name":string, "Period":i64, "Deadline":i64, "Offset":i64, "Start":i64, "Priority":i32, "Timeout":i32, "Mode":T10, "Wakeup Reason":T11, "Error":errorcluster, "Source Type":string, "Secondary Source Type":string, "Global End Time":u64, "Global Start Time":u64, "Frame Duration":u64, "Iteration Duration":u64, "Assigned CPU":i32, "I/O Scan Engine Mode":u32}
  T10 = typedef "XDNodeRunTimeDep.lvlib/nitl_modes.ctl" = enum32{"No Change", "Process missed periods, maintain original phase", "Discard missed periods, maintain original phase", "Process missed periods, ignore original phase", "Discard missed periods, ignore original phase"}
  T11 = typedef "XDNodeRunTimeDep.lvlib/wakeup.ctl" = enum32{"Normal", "Aborted", "Asynchronous wakeup", "Timing source error", "Timed loop error", "Timeout"}
  T12 = typedef "Image Type" = u32
  T13 = cluster{"button 1":bool, "button 2":bool, "button 3":bool, "button 4":bool}
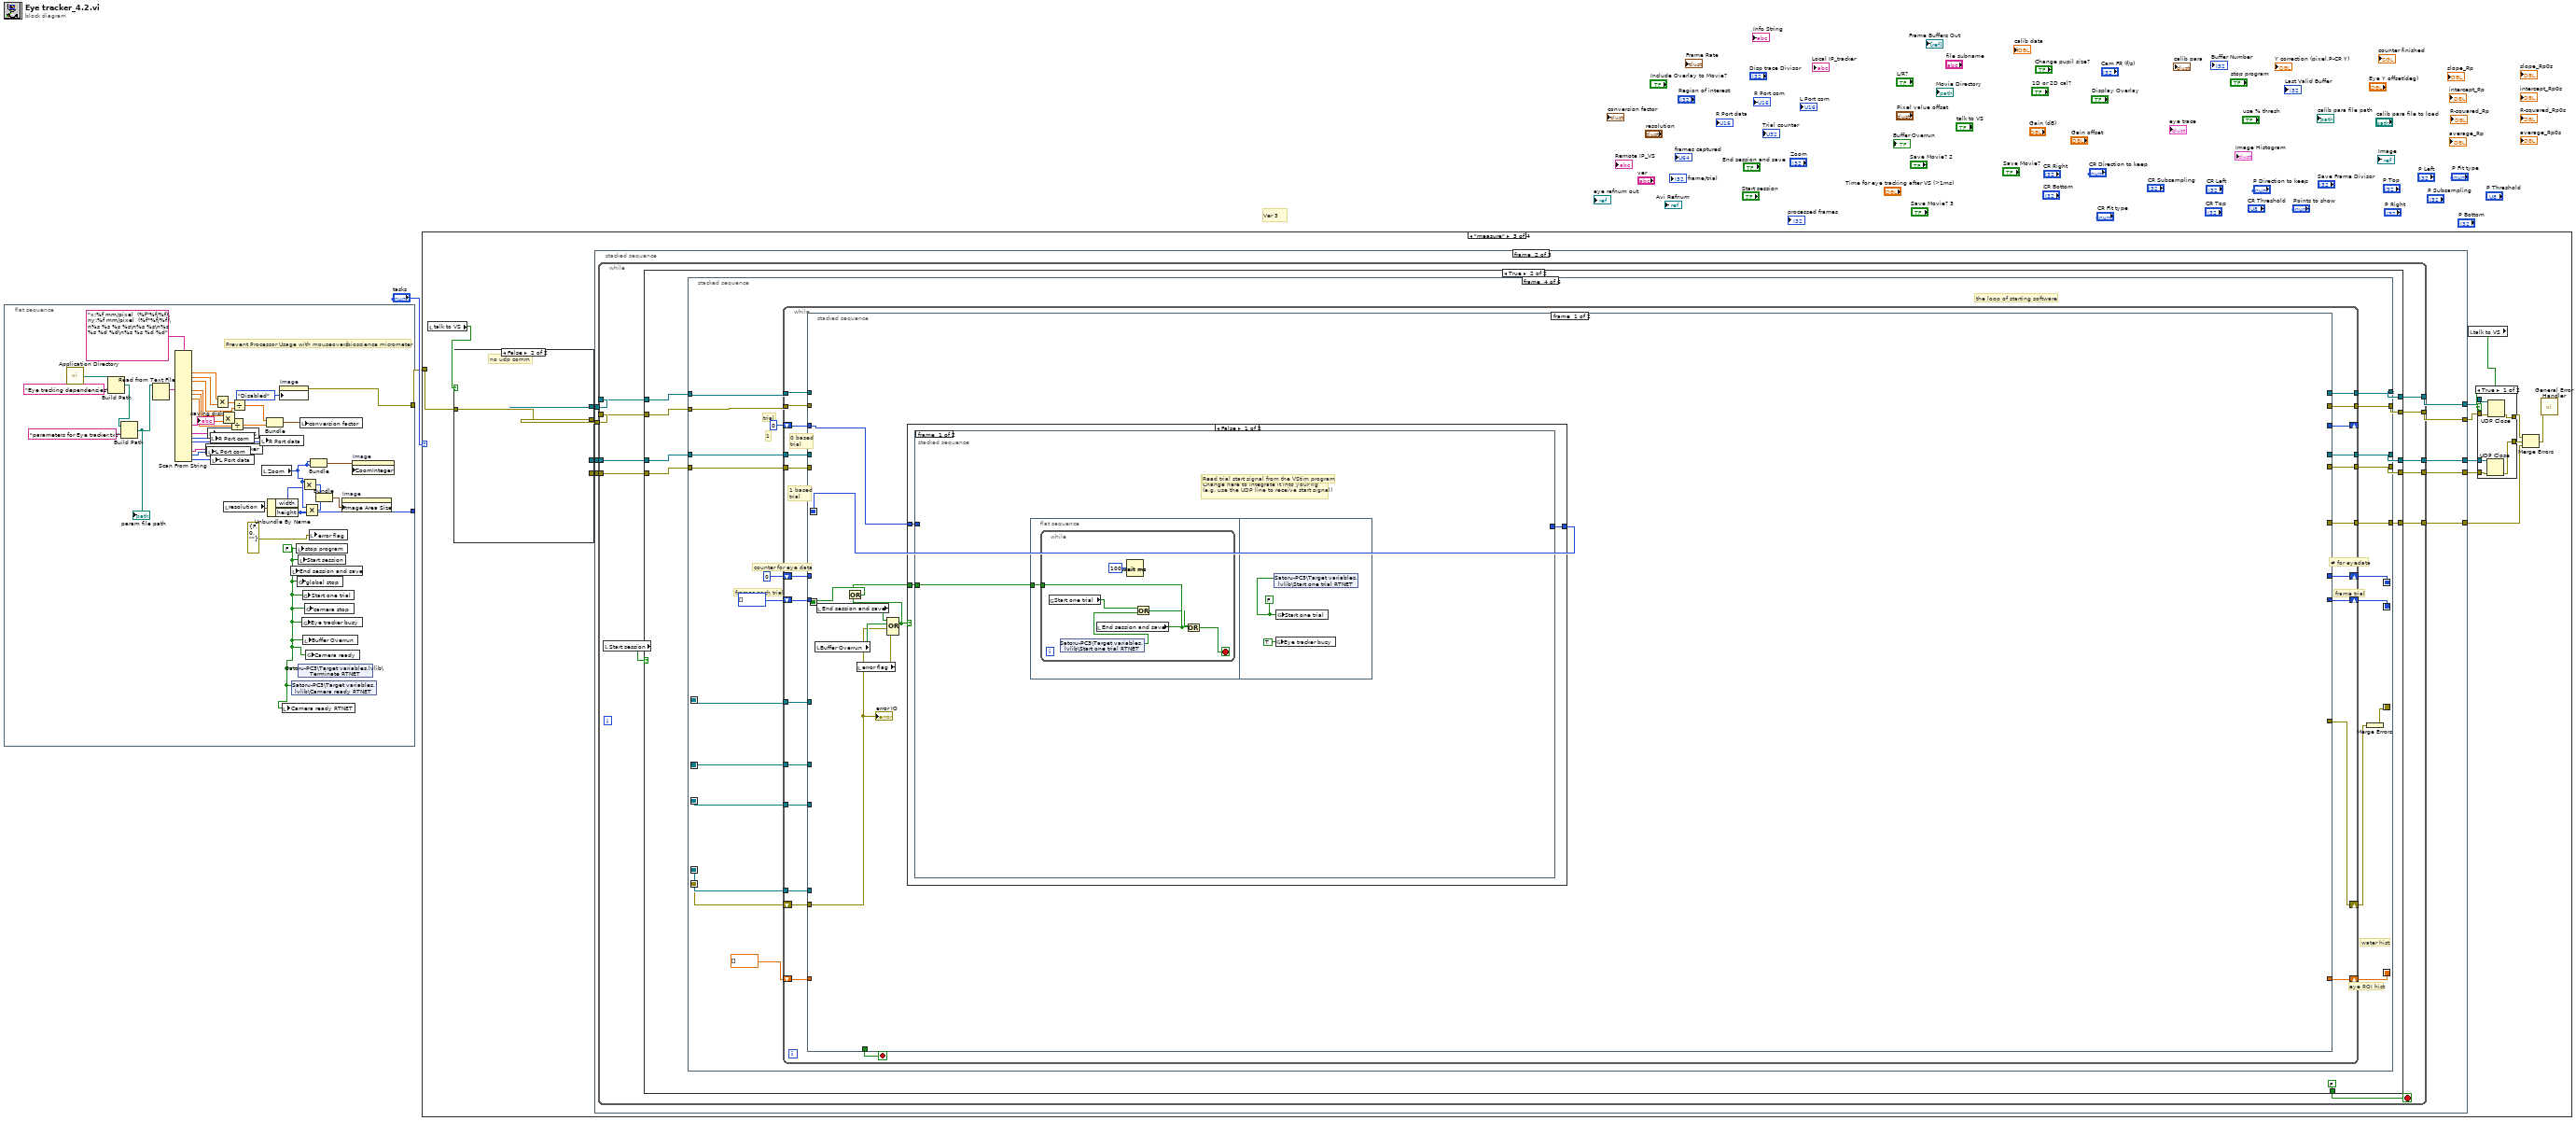
[diagram p0: block diagram]
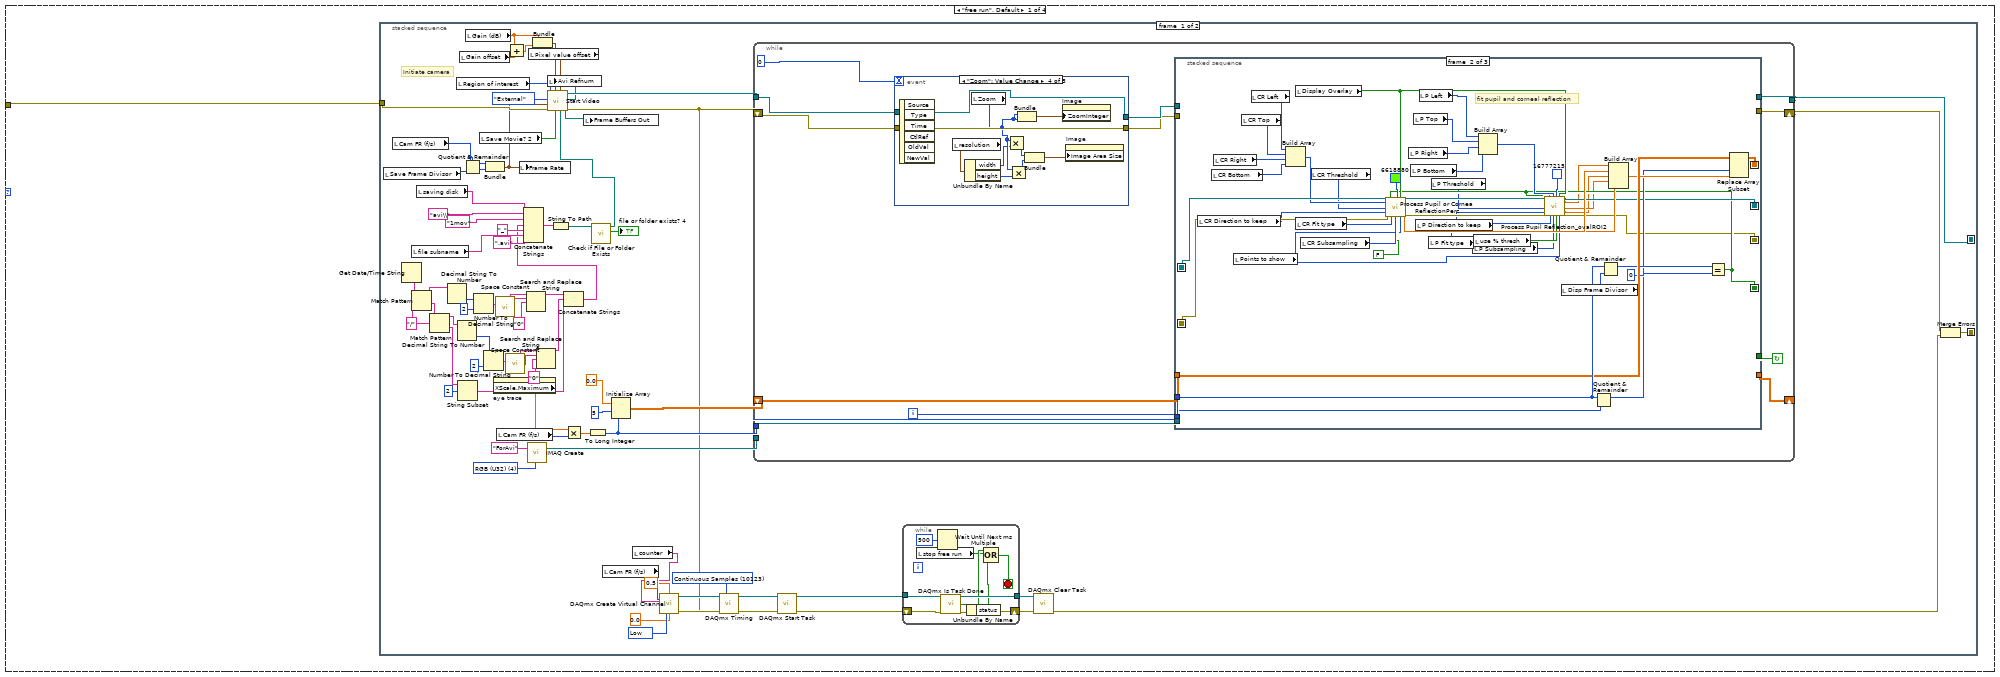
[diagram p2: hidden frame]
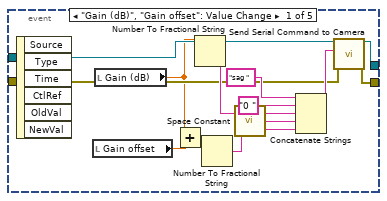
[diagram p3: hidden frame]
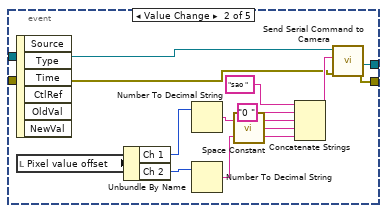
[diagram p4: hidden frame]
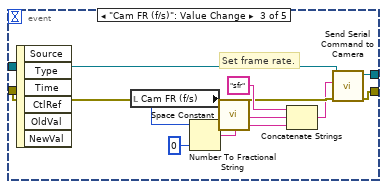
[diagram p5: hidden frame]
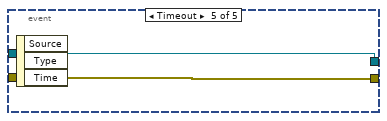
[diagram p6: hidden frame]
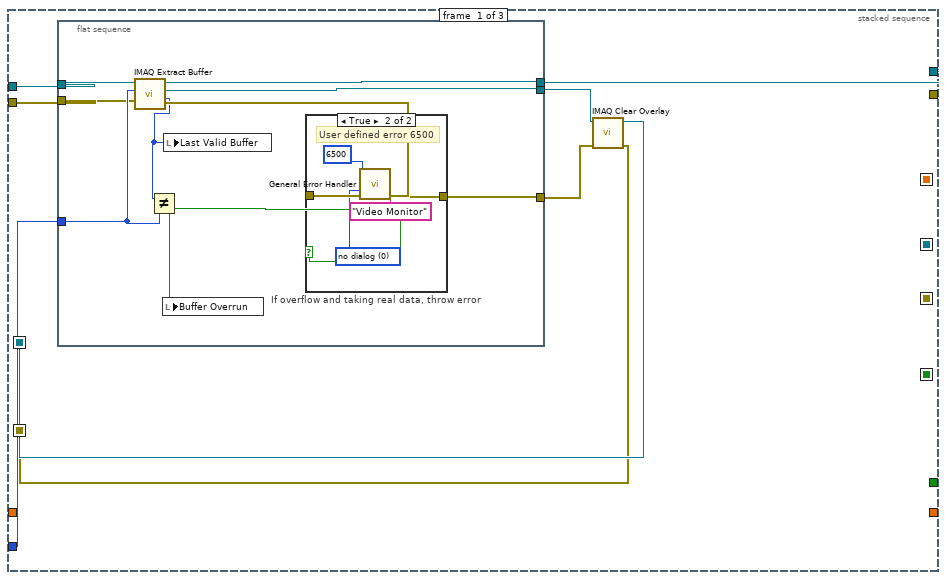
[diagram p7: hidden frame]
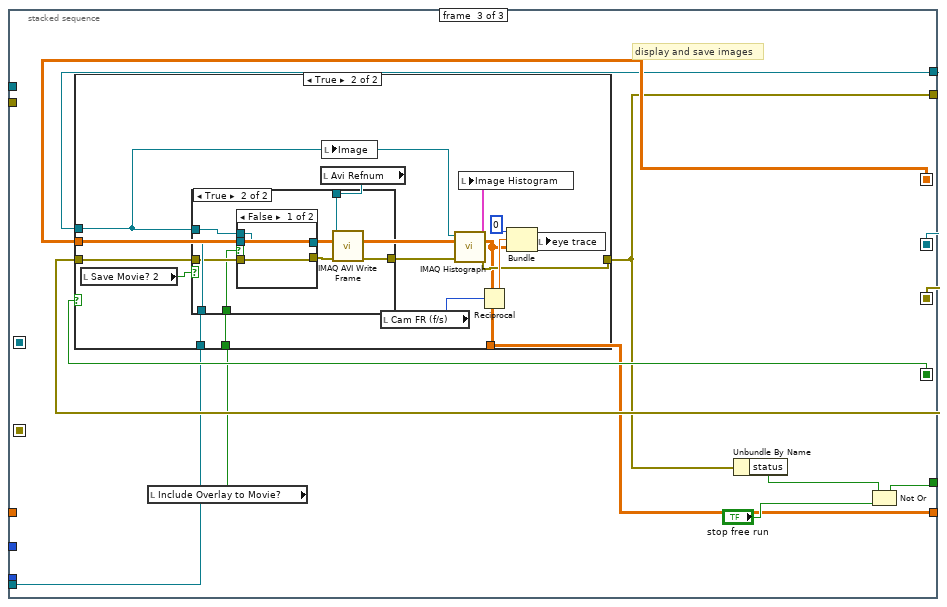
[diagram p9: hidden frame]
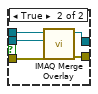
[diagram p12: hidden frame]
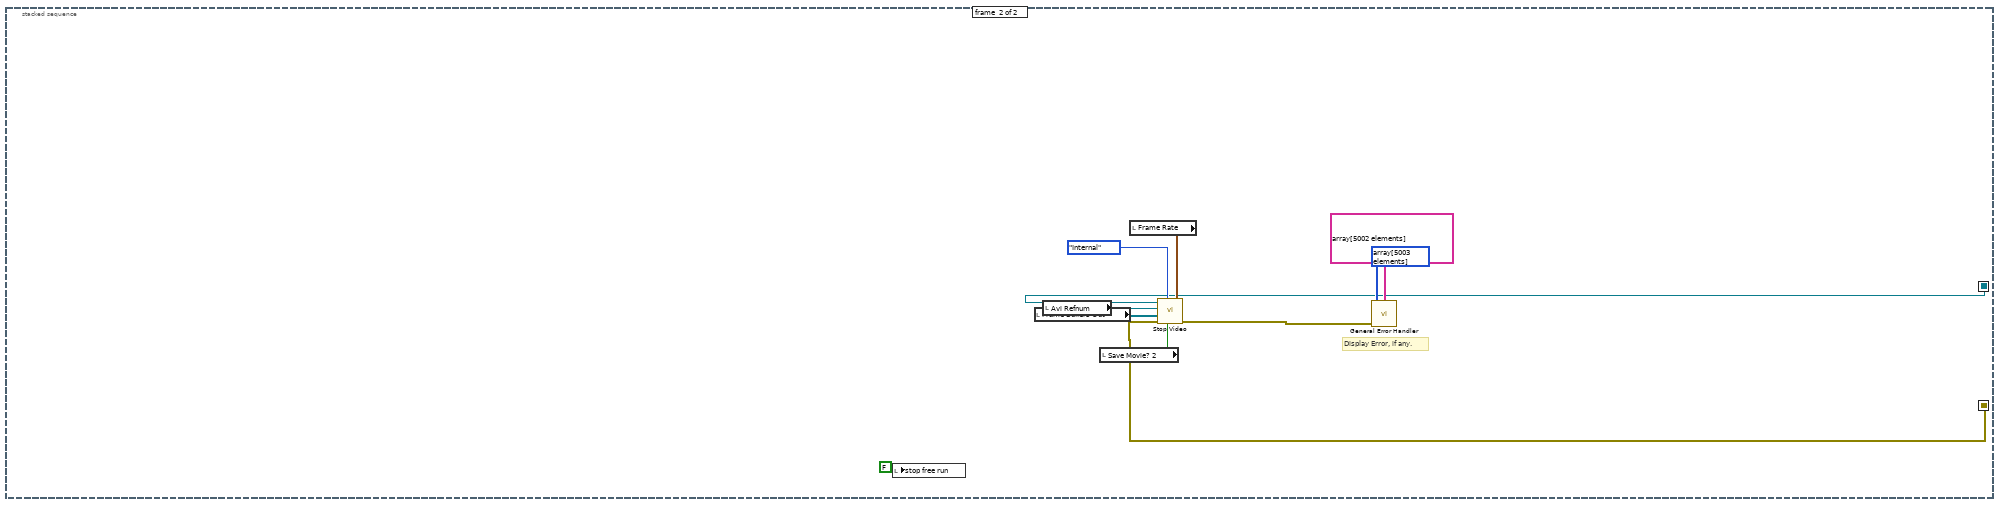
[diagram p13: hidden frame]
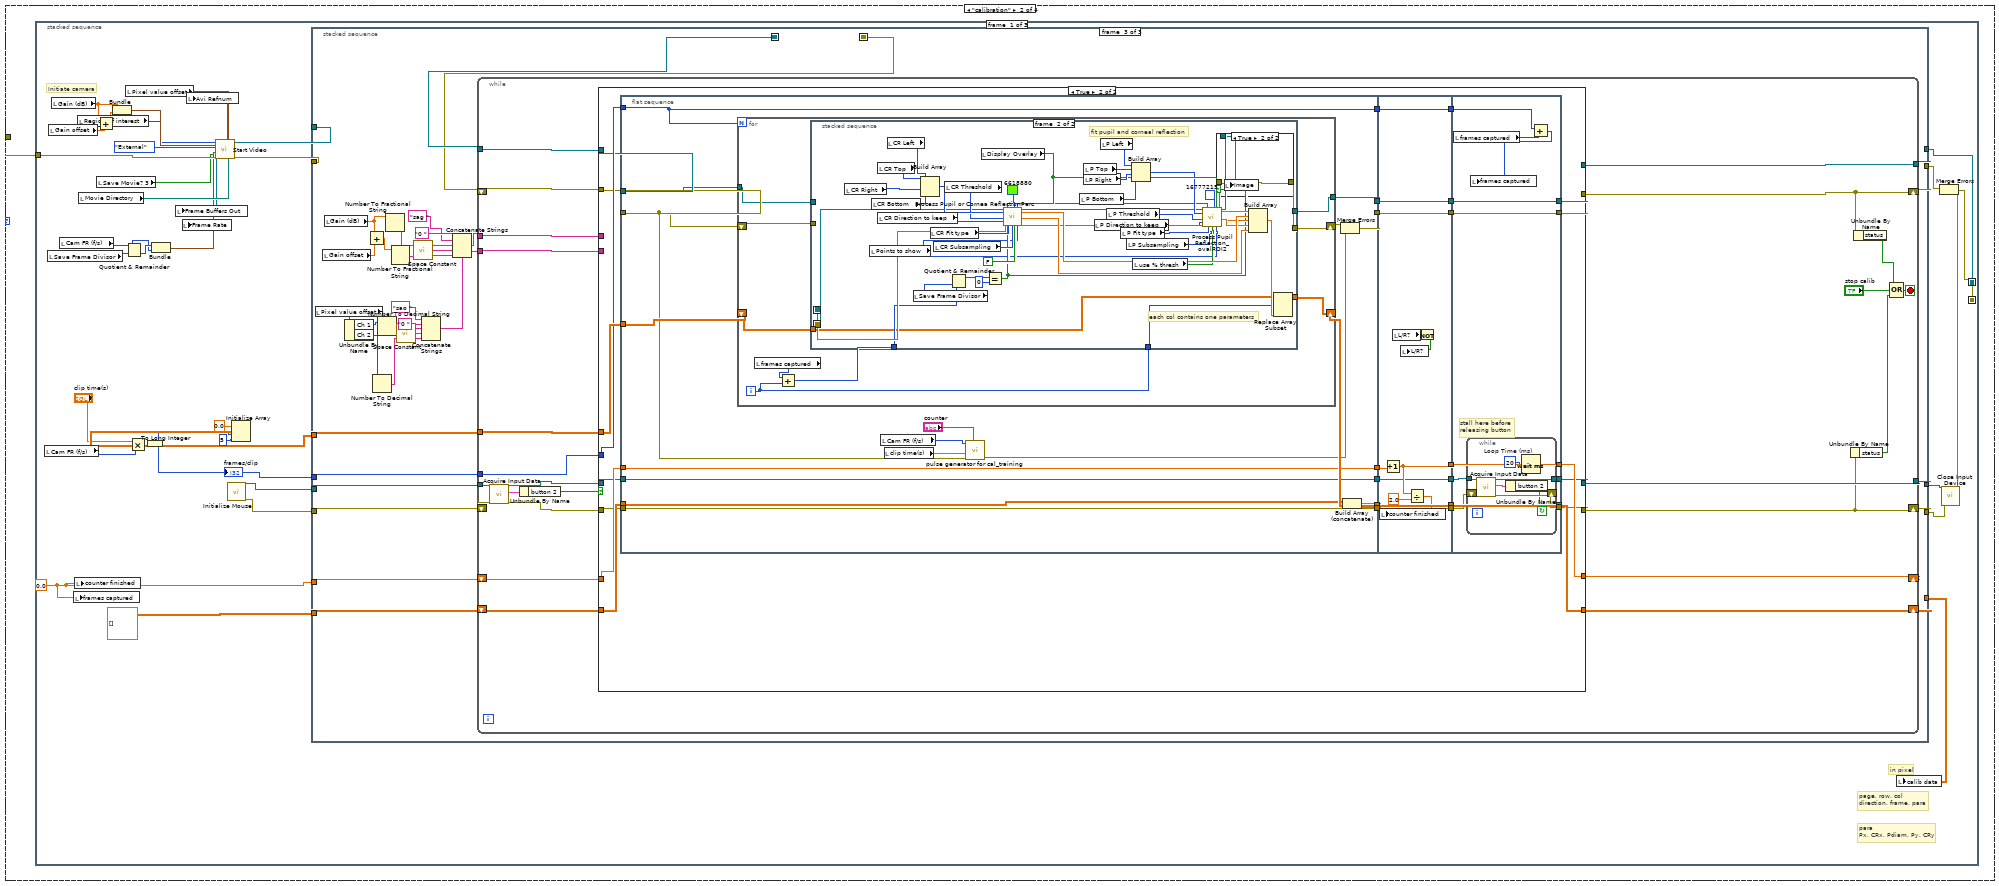
[diagram p14: hidden frame]
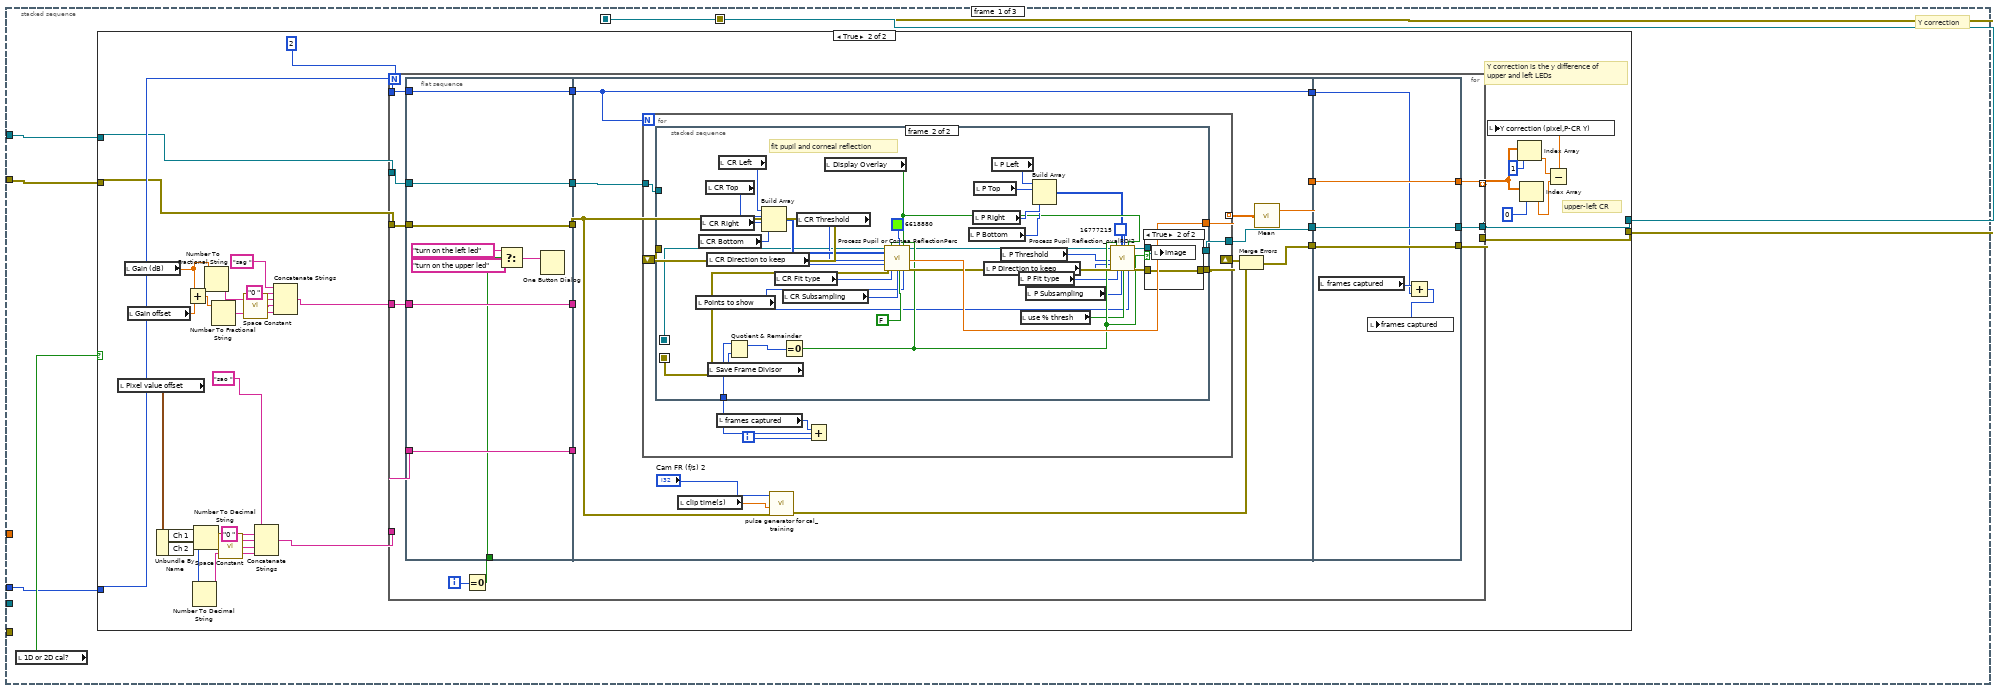
[diagram p15: hidden frame]
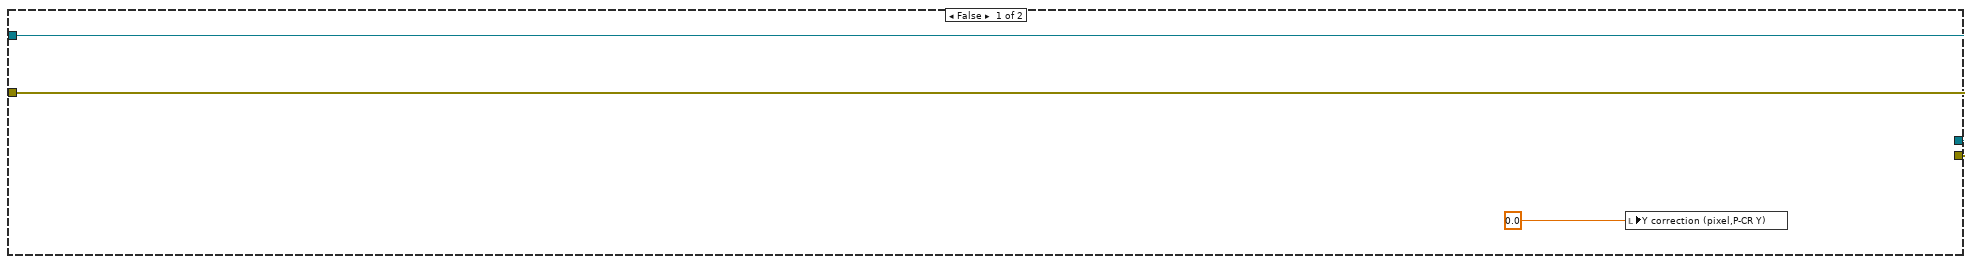
[diagram p16: hidden frame]
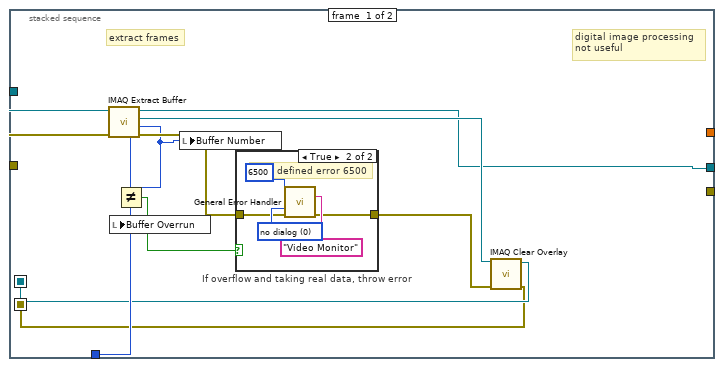
[diagram p17: hidden frame]
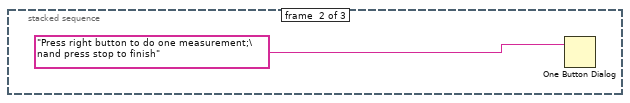
[diagram p20: hidden frame]
diagram:
  # "Ver 3"
  n1 = flat-sequence {
    tunnel: [w35] -> w1
    tunnel: [w30] -> _
    frame #0 {
      w3 = FALSE ("stop meausre")
      # "155 pixels for 4 mm using MBF bioscience micrometer"
      # "Prevent Processor Usage with mouseovers"
      n2 = call <vilib>:"Application Directory.vi"() -> ("Application Directory"=w21:path)
      n3 = Build Path(base path=w21, name or relative path="Eye tracking dependencies") -> (appended path=w5:path)
      n4 = Build Path(base path=w5, name or relative path="parameters for Eye tracker.txt") -> (appended path=w4:path)
      "param file path" <- w4
      n5 = Read from Text File(file (use dialog)=w4) -> (text=w24:string)  [unwired: 3 in, 3 out]
      n6 = Scan From String(format string="x:%f mm/pixel  (%f*%f/%f)\ny:%f mm/pixel  (%f*%f/%f)\n%s %s %s %s\n%s %s\n%s %s %d %d\n%s %s %d %d", input string=w24) -> (output 2=w20:dbl, output 3=w19:dbl, output 4=w18:dbl, output 6=w17:dbl, output 7=w16:dbl, output 8=w15:dbl, output 14=→"saving disk":string, output 16=w13:string, output 17=w12:i32, output 18=w11:i32, output 20=w10:string, output 21=w9:i32, output 22=w8:i32)  [unwired: 33 in, 3 out]
      n7 = local write "Local IP_tracker"(w10) -> ()
      n8 = local write "L Port com"(w9) -> ()
      n9 = local write "Remote IP_VS"(w13) -> ()
      n10 = local write "R Port com"(w12) -> ()
      n11 = local write "L Port data"(w8) -> ()
      n12 = Multiply(x=w20, y=w19) -> (x*y=w28:dbl)
      n13 = Multiply(x=w17, y=w16) -> (x*y=w26:dbl)
      n14 = local read "resolution"() -> (w32:cluster{"width":u16, "height":u16})
      n15 = Divide(x=w26, y=w15) -> (x/y=w25:dbl)
      n16 = Divide(x=w28, y=w18) -> (x/y=w27:dbl)
      n17 = local write "R Port data"(w11) -> ()
      n18 = local read "Zoom"() -> (w39:i32)
      n19 = Bundle(w27, w25) -> (w29:cluster{dbl, dbl})  [unwired: 1 in]
      n20 = Unbundle By Name(w32) -> ("width"=w31:u16, "height"=w30:u16)
      n21 = property on="Image" class="ImageControl"("DisabledEnum"=T6."Disabled" ("Disabled")) -> (error out=w35:errorcluster)  [unwired: 2 in, 1 out]
      n22 = local write "Camera ready RTNET"(w3) -> ()
      n23 = local write "End session and save"(w3) -> ()
      n24 = shared-variable "Satoru-PC3\\Target variables.lvlib\\Camera ready RTNET"(w3) -> ()  [unwired: 1 in, 1 out]
      n25 = local write "stop program"(w3) -> ()
      n26 = global write "Global 1.vi" "global stop"(w3) -> ()
      n27 = shared-variable "Satoru-PC3\\Target variables.lvlib\\Terminate RTNET"(w3) -> ()  [unwired: 1 in, 1 out]
      n28 = local write "Start session"(w3) -> ()
      n29 = local write "conversion factor"(w29) -> ()
      n30 = Multiply(x=w39, y=w31) -> (x*y=w37:i32)
      n31 = global write "Global 1.vi" "Eye tracker busy"(w3) -> ()
      n32 = global write "Global 1.vi" "Start one trial"(w3) -> ()
      n33 = local write "Buffer Overrun"(w3) -> ()
      n34 = Multiply(x=w39, y=w30) -> (x*y=w38:i32)
      n35 = global write "Global 1.vi" "camera stop"(w3) -> ()
      n36 = global write "Global 1.vi" "Camera ready"(w3) -> ()
      n37 = local write "error flag"(errorcluster {"status"=FALSE, "code"=0, "source"=""} ("error constant")) -> ()
      n38 = Bundle("Zoom"=w39, "Zoom"=w39) -> (w34:cluster{"Zoom":i32, "Zoom":i32})  [unwired: 1 in]
      n39 = Bundle(w37, w38) -> (w33:cluster{i32, i32})  [unwired: 1 in]
      n40 = property on="Image" class="ImageControl"("Image Area Size"=w33) -> ()  [unwired: 2 in, 2 out]
      n41 = property on="Image" class="ImageControl"("ZoomInteger"=w34) -> ()  [unwired: 2 in, 2 out]
    }
  }
  n42 = case shown="\"measure\"" "tasks" {
    tunnel: w1 -> [w40 w309 w936 _]
    frame "free run", Default {
      n43 = stacked-sequence {
        seq-local: [w46 _] -> [_ w298]
        seq-local: [w106 _] -> [_ w299]
        tunnel: w40 -> [w99 _]
        frame #0 {
          w50 = 10123 items=["Finite Samples"=10178, "Continuous Samples"=10123, "Hardware Timed Single Point"=12522] ("sample mode")
          w55 = 10214 items=["High"=10192, "Low"=10214] ("idle state")
          w80 = "/"
          w109 = T12 4 items=["Grayscale (U8)", "Grayscale (I16)", "Grayscale (SGL)", "Complex (CSG)", "RGB (U32)", "HSL (U32)", "RGB (U64)"] ("Image Type")
          # "Initiate camera"
          n44 = local read "Save Frame Divisor"() -> (w103:i32)
          n45 = local read "Cam FR (f/s)"() -> (w96:i32)
          n46 = Get Date/Time String() -> (date string=w82:string)  [unwired: 3 in, 1 out]
          n47 = local read "file subname"() -> (w83:string)
          n48 = Match Pattern(string=w82, regular expression=w80) -> (before substring=w79:string, after substring=w81:string)  [unwired: 1 in, 2 out]
          n49 = local read "saving disk"() -> (w44:string)
          n50 = Match Pattern(string=w81, regular expression=w80) -> (before substring=w78:string, after substring=w67:string)  [unwired: 1 in, 2 out]
          n51 = Decimal String To Number(string=w79) -> (number=w73:i32)  [unwired: 2 in, 1 out]
          n52 = local read "Region of interest"() -> (w91:i32[])
          n53 = Decimal String To Number(string=w78) -> (number=w70:i32)  [unwired: 2 in, 1 out]
          n54 = String Subset(string=w67, offset (0)=2) -> (substring=w63:string)  [unwired: 1 in]
          n55 = local read "Gain offset"() -> (w104:dbl)
          n56 = Quotient & Remainder(x=w96, y=w103) -> (floor(x/y)=w97:i32)  [unwired: 1 out]
          n57 = local read "Gain (dB)"() -> (w102:dbl)
          n58 = Number To Decimal String(number=w73, width (-)=i16 2) -> (decimal integer string=w76:string)
          n59 = local read "Save Movie? 2"() -> (w90:bool)
          n60 = Number To Decimal String(number=w70, width (-)=i16 2) -> (decimal integer string=w72:string)
          n61 = Bundle(w97, "Cam FR (f/s)"=w96) -> (w92:cluster{i32, "Cam FR (f/s)":i32})  [unwired: 1 in]
          n62 = property on="eye trace" class="WFGraph (strict)"() -> ("XScale.Maximum"=w113:dbl)  [unwired: 2 in, 2 out]
          n63 = call <vilib>:"Space Constant.vi"() -> ("String"=w75:string)
          n64 = local read "Cam FR (f/s)"() -> (w112:i32)
          n65 = call <vilib>:"Space Constant.vi"() -> ("String"=w71:string)
          n66 = Add(x=w102, y=w104) -> (x+y=w101:dbl)
          n67 = local write "Frame Rate"(w92) -> ()
          n68 = Search and Replace String(input string=w76, search string=w75, replace string="0" ("replace string (\"\")")) -> (result string=w65:string)  [unwired: 5 in, 3 out]
          n69 = call "IMAQ Create"("Image Name"="ForAvi", "Image Type"=w109) -> ("New Image"=w107:T2)  [unwired: 3 in, 1 out]
          n70 = local read "Pixel value offset"() -> (w95:cluster{"Ch 1":u8, "Ch 2":u8})
          n71 = Bundle("Gain (dB)"=w102, w101) -> (w100:cluster{"Gain (dB)":dbl, dbl})  [unwired: 1 in]
          n72 = Search and Replace String(input string=w72, search string=w71, replace string="0" ("replace string (\"\")")) -> (result string=w64:string)  [unwired: 5 in, 3 out]
          n73 = Concatenate Strings(w65, w64, w63) -> (w62:string)
          n74 = Concatenate Strings(w44, "avi\\" ("string"), "1mov" ("string"), w62, "_" ("string"), w83, ".avi" ("string")) -> (w85:string)
          n75 = String To Path(string=w85) -> (path=w84:path)
          n76 = Multiply(x=w113, y=w112) -> (x*y=w111:dbl)
          n77 = To Long Integer(number=w111) -> (32bit integer=w110:i32)
          n78 = call <vilib>:"Check if File or Folder Exists.vi"("path"=w84) -> ("file or folder exists?"=→"file or folder exists? 4":bool, "dup path"=w61:path)  [unwired: 8 in, 1 out]
          n79 = call "Start Video.vi"("AVI Path"=w61, "Offset"=w95, "Save Movie?"=w90, "Gain(dB)"=w100, "error in"=w99, "Frame Rate(Hz)"=w92, "Trigger Type"=enum16{"Internal", "External"}."External", "Region of interest"=w91) -> ("error out"=w48:errorcluster, "Frame Buffers Out"=w93:T2[], "Avi Refnum"=w94:T3, "IMAQ Session Out"=w98:refnum<k11>)
          n80 = local write "Avi Refnum"(w94) -> ()
          n81 = local write "Frame Buffers Out"(w93) -> ()
          n82 = local read "Cam FR (f/s)"() -> (w49:i32)
          n83 = Initialize Array(0.0, 5 ("dimension size"), w110) -> (w114:dbl[][])
          n84 = local read "counter"() -> (w43:tag)
          n85 = call-poly <vilib>:"DAQmx Create Virtual Channel.vi"("frequency"=w49, "duty cycle"=0.5, "counter"=w43, "error in"=w48, "idle state"=w55, "initial delay"=0.0) -> ("task out"=w58:refnum<k21>, "error out"=w59:errorcluster)  [unwired: 8 in]
          n86 = call-poly <vilib>:"DAQmx Timing.vi"("task/channels in"=w58, "sample mode"=w50, "error in"=w59) -> ("task out"=w52:refnum<k21>, "error out"=w51:errorcluster)  [unwired: 11 in]
          n87 = while {
            shift-right: [w134] -> w47
            shift-left: w48 -> [w127]
            shift-right: [w131] -> _
            shift-left: w114 -> [w136]
            tunnel: w110 -> [w137]
            tunnel: w107 -> [w135]
            tunnel: w98 -> [w129]
            tunnel: [w132] -> w106
            i -> [w138]
            stop <- w133 continue-if-true
            n88 = event shown="[3] \"Zoom\": Value Change" {
              selector: _ -> [_ _ _ _ _]
              dyn-events: _ -> [_ _ _ _ _]
              timeout: 0 -> [_ _ _ _ _]
              tunnel: w129 -> [w145 w155 w167 w175 w185]
              tunnel: w127 -> [w143 w153 w169 w182 w186]
              tunnel: [w139 w152 w170 w182 w186] -> w126
              tunnel: [w140 w154 w165 w175 w185] -> w128
              event "Gain (dB)", "Gain offset": Value Change {
                n89 = event-data() -> ()  [unwired: 1 in, 6 out]
                n90 = local read "Gain offset"() -> (w141:dbl)
                n91 = local read "Gain (dB)"() -> (w142:dbl)
                n92 = Add(x=w142, y=w141) -> (x+y=w146:dbl)
                n93 = Number To Fractional String(number=w142) -> (F-format string=w147:string)  [unwired: 3 in]
                n94 = Number To Fractional String(number=w146) -> (F-format string=w149:string)  [unwired: 3 in]
                n95 = call <vilib>:"Space Constant.vi"() -> ("String"=w148:string)
                n96 = Concatenate Strings("sag " ("String to write"), "0 " ("string"), w147, w148, w149) -> (w144:string)
                n97 = call "Send Serial Command to Camera.vi"("error in (no error)"=w143, "String to write"=w144, "IMAQ Session In"=w145) -> ("error out"=w139:errorcluster, "IMAQ Session Out"=w140:refnum<k11>)  [unwired: 5 in, 2 out]
              }
              event "Pixel value offset.Ch 1", "Pixel value offset.Ch 2": Value Change {
                n98 = event-data() -> ()  [unwired: 1 in, 6 out]
                n99 = local read "Pixel value offset"() -> (w160:cluster{"Ch 1":u8, "Ch 2":u8})
                n100 = Unbundle By Name(w160) -> ("Ch 1"=w159:u8, "Ch 2"=w157:u8)
                n101 = Number To Decimal String(number=w159) -> (decimal integer string=w158:string)  [unwired: 1 in]
                n102 = Number To Decimal String(number=w157) -> (decimal integer string=w156:string)  [unwired: 1 in]
                n103 = call <vilib>:"Space Constant.vi"() -> ("String"=w162:string)
                n104 = Concatenate Strings("sao " ("String to write"), "0 " ("string"), w158, w162, w156) -> (w161:string)
                n105 = call "Send Serial Command to Camera.vi"("error in (no error)"=w153, "String to write"=w161, "IMAQ Session In"=w155) -> ("error out"=w152:errorcluster, "IMAQ Session Out"=w154:refnum<k11>)  [unwired: 5 in, 2 out]
              }
              event "Cam FR (f/s)": Value Change {
                # "Set frame rate."
                n106 = event-data() -> ()  [unwired: 1 in, 6 out]
                n107 = local read "Cam FR (f/s)"() -> (w166:i32)
                n108 = Number To Fractional String(number=w166, precision (6)=i16 0) -> (F-format string=w172:string)  [unwired: 2 in]
                n109 = call <vilib>:"Space Constant.vi"() -> ("String"=w173:string)
                n110 = Concatenate Strings("sfr" ("string"), w173, w172) -> (w168:string)
                n111 = call "Send Serial Command to Camera.vi"("error in (no error)"=w169, "String to write"=w168, "IMAQ Session In"=w167) -> ("error out"=w170:errorcluster, "IMAQ Session Out"=w165:refnum<k11>)  [unwired: 5 in, 2 out]
              }
              event "Zoom": Value Change {
                n112 = event-data() -> ()  [unwired: 1 in, 6 out]
                n113 = local read "resolution"() -> (w178:cluster{"width":u16, "height":u16})
                n114 = Unbundle By Name(w178) -> ("width"=w177:u16, "height"=w176:u16)
                n115 = local read "Zoom"() -> (w181:i32)
                n116 = Multiply(x=w181, y=w177) -> (x*y=w184:i32)
                n117 = Multiply(x=w181, y=w176) -> (x*y=w183:i32)
                n118 = Bundle("Zoom"=w181, "Zoom"=w181) -> (w180:cluster{"Zoom":i32, "Zoom":i32})  [unwired: 1 in]
                n119 = Bundle(w184, w183) -> (w179:cluster{i32, i32})  [unwired: 1 in]
                n120 = property on="Image" class="ImageControl"("ZoomInteger"=w180) -> ()  [unwired: 2 in, 2 out]
                n121 = property on="Image" class="ImageControl"("Image Area Size"=w179) -> ()  [unwired: 2 in, 2 out]
              }
              event Timeout {
                n122 = event-data() -> ()  [unwired: 1 in, 3 out]
              }
            }
            n123 = stacked-sequence {
              seq-local: [w188 _ _] -> [_ w253 _]
              seq-local: [w187 _ _] -> [_ w254 _]
              seq-local: [_ w249 _] -> [_ _ w265]
              seq-local: [_ w217 _] -> [_ _ w263]
              seq-local: [_ w226 _] -> [_ _ w264]
              seq-local: [_ w221 _] -> [_ _ w262]
              tunnel: w138 -> [w194 w252 _]
              tunnel: w126 -> [w193 _ _]
              tunnel: [w190 _ _] -> w132
              tunnel: w137 -> [_ w251 _]
              tunnel: w136 -> [_ w250 _]
              tunnel: w135 -> [_ _ w261]
              tunnel: [_ _ w257] -> w134
              tunnel: [_ _ w256] -> w133
              tunnel: w128 -> [w189 _ _]
              tunnel: [_ _ w255] -> w131
              frame #0 {
                n124 = flat-sequence {
                  tunnel: w193 -> [w195]
                  tunnel: [w203] -> w192
                  tunnel: [w201] -> w191
                  tunnel: w194 -> [w199]
                  tunnel: [w197] -> w190
                  tunnel: w189 -> [w196]
                  frame #0 {
                    n125 = call <vilib>:"IMAQ Extract Buffer.vi"("error in (no error)"=w195, "Buffer to extract"=w199, "IMAQ Session In"=w196) -> ("error out"=w202:errorcluster, "Buffer Number"=w200:i32, "Image Out"=w201:T2, "IMAQ Session Out"=w197:refnum<k11>)  [unwired: 3 in, 2 out]
                    n126 = Not Equal?(x=w200, y=w199) -> (x != y?=w198:bool)
                    n127 = local write "Buffer Overrun"(w198) -> ()
                    n128 = local write "Last Valid Buffer"(w200) -> ()
                    n129 = case "If overflow and taking real data, throw error" shown="True" w198 {
                      tunnel: w202 -> [w204 w206]
                      tunnel: [w204 w205] -> w203
                      frame False {
                      }
                      frame True {
                        w207 = u16 0 items=["no dialog", "OK message", "continue or stop message"] ("type of dialog (OK msg:1)")
                        # "User defined error 6500"
                        n130 = call <vilib>:"General Error Handler.vi"("[error code] (0)"=6500 ("error code (no error:0)"), "[error source] (\" \")"="Video Monitor" ("[error source] (\" \")"), "type of dialog (OK msg:1)"=w207, "error in (no error)"=w206) -> ("error out"=w205:errorcluster)  [unwired: 7 in, 4 out]
                      }
                    }
                  }
                }
                n131 = call "IMAQ Clear Overlay"("error in (no error)"=w192, "Image"=w191) -> ("error out"=w187:errorcluster, "Image Out"=w188:T2)  [unwired: 8 in]
              }
              frame #1 {
                # "fit pupil and corneal reflection"
                n132 = local read "CR Direction to keep"() -> (w236:enum16{"Above", "Below"})
                n133 = local read "CR Bottom"() -> (w238:i32)
                n134 = local read "CR Right"() -> (w239:i32)
                n135 = local read "Points to show"() -> (w210:enum16{"All points", "Fit points"})
                n136 = local read "CR Top"() -> (w240:i32)
                n137 = local read "CR Left"() -> (w241:i32)
                n138 = Build Array(w241, w240, w239, w238) -> (w243:i32[])
                n139 = local read "Display Overlay"() -> (w222:bool)
                n140 = local read "CR Fit type"() -> (w235:enum16{"Circle", "Ellipse"})
                n141 = local read "CR Subsampling"() -> (w234:i32)
                n142 = local read "CR Threshold"() -> (w237:u8)
                n143 = local read "P Right"() -> (w231:i32)
                n144 = local read "P Bottom"() -> (w230:i32)
                n145 = local read "P Top"() -> (w232:i32)
                n146 = local read "P Direction to keep"() -> (w214:enum16{"Above", "Below"})
                n147 = local read "P Left"() -> (w233:i32)
                n148 = local read "P Fit type"() -> (w213:enum16{"Circle", "Ellipse"})
                n149 = local read "P Threshold"() -> (w215:u8)
                n150 = local read "P Subsampling"() -> (w211:i32)
                n151 = local read "use % thresh"() -> (w212:bool)
                n152 = Build Array(w233, w232, w231, w230) -> (w223:i32[])
                n153 = local read "Disp Frame Divisor"() -> (w229:i32)
                n154 = Quotient & Remainder(x=w252, y=w251) -> (x-y*floor(x/y)=w228:i32)  [unwired: 1 out]
                n155 = Quotient & Remainder(x=w252, y=w229) -> (x-y*floor(x/y)=w248:i32)  [unwired: 1 out]
                n156 = Equal?(x=w248, y=0) -> (x = y?=w221:bool)
                n157 = call "Process Pupil or Cornea ReflectionPerc.vi"("Image In"=w253, "ROI"=w243, "Threshold"=w237, "Direction to keep"=w236, "error in (no error)"=w254, "Display"=w221, "Fit type"=w235, "Subsampling"=w234, "Color"=u32 6618880, "use % thresh"=FALSE, "Display Overlay"=w222, "Points to show"=w210) -> ("Image out"=w225:T2, "x position"=w246:dbl, "y position"=w244:dbl, "error out"=w216:errorcluster)  [unwired: 3 in, 1 out]
                n158 = call "Process Pupil Reflection_ovalROI2.vi"("Image In"=w225, "Threshold"=w215, "Direction to keep"=w214, "error in (no error)"=w216, "Display"=w221, "Fit type"=w213, "Global Rectangle"=w223, "Subsampling"=w211, "Color"=u32 16777215, "use % thresh"=w212, "Display Overlay"=w222, "Points to show"=w210) -> ("Image out"=w226:T2, "x position"=w220:dbl, "y position"=w219:dbl, "diameter"=w218:dbl, "error out"=w217:errorcluster)  [unwired: 3 in]
                n159 = Build Array(w220, w246, w218, w219, w244) -> (w245:dbl[])
                n160 = Replace Array Subset(array=w250, new element=w245, index (col)=w228) -> (w249:dbl[][])  [unwired: 1 in]
              }
              frame #2 {
                # "display and save images"
                n161 = local read "Include Overlay to Movie?"() -> (w260:bool)
                n162 = case shown="True" w262 {
                  tunnel: w263 -> [w267 w278]
                  tunnel: [w267 w275] -> w257
                  tunnel: w264 -> [_ w270]
                  tunnel: w261 -> [_ w279]
                  tunnel: w260 -> [_ w276]
                  tunnel: w265 -> [w266 w274]
                  tunnel: [w266 w274] -> w255
                  frame False {
                  }
                  frame True {
                    n163 = local read "Save Movie? 2"() -> (w268:bool)
                    n164 = local read "Avi Refnum"() -> (w271:T3)
                    n165 = case shown="True" w268 {
                      tunnel: w271 -> [_ w288]
                      tunnel: w279 -> [_ w287]
                      tunnel: w270 -> [_ w286]
                      tunnel: w278 -> [w282 w285]
                      tunnel: [w282 w284] -> w277
                      tunnel: w276 -> [_ w283]
                      frame False {
                      }
                      frame True {
                        n166 = case shown="False" w283 {
                          tunnel: [w291 w297] -> w290
                          tunnel: [w292 w296] -> w289
                          tunnel: w287 -> [_ w295]
                          tunnel: w286 -> [w291 w294]
                          tunnel: w285 -> [w292 w293]
                          frame False {
                          }
                          frame True {
                            n167 = call "IMAQ Merge Overlay"("error in (no error)"=w293, "Image Dst"=w295, "Image Src"=w294) -> ("error out"=w296:errorcluster, "Image Dst Out"=w297:T2)  [unwired: 7 in]
                          }
                        }
                        n168 = call "IMAQ AVI Write Frame"("error in (no error)"=w289, "Image"=w290, "Avi Refnum"=w288) -> ("error out"=w284:errorcluster)  [unwired: 7 in, 1 out]
                      }
                    }
                    n169 = local write "Image"(w270) -> ()
                    n170 = local read "Cam FR (f/s)"() -> (w273:i32)
                    n171 = call "IMAQ Histograph"("error in (no error)"=w277, "Image"=w270) -> ("error out"=w275:errorcluster, "Histogram Graph"=w269:T5)  [unwired: 6 in, 2 out]
                    n172 = local write "Image Histogram"(w269) -> ()
                    n173 = Reciprocal(x=w273) -> (1/x=w280:dbl)
                    n174 = Bundle(0, w280, w274) -> (w272:cluster{i32, dbl, dbl[][]})  [unwired: 1 in]
                    n175 = local write "eye trace"(w272) -> ()
                  }
                }
                n176 = Unbundle By Name(w257) -> ("status"=w259:bool)
                n177 = Not Or(1:"stop free run", 2:w259) -> (0:w256:bool)
              }
            }
          }
          n178 = call <vilib>:"DAQmx Start Task.vi"("task/channels in"=w52, "error in"=w51) -> ("task out"=w57:refnum<k21>, "error out"=w53:errorcluster)  [unwired: 12 in]
          n179 = while {
            tunnel: w57 -> [w124]
            tunnel: [w123] -> w56
            shift-right: [w121] -> w54
            shift-left: w53 -> [w119]
            stop <- w125 stop-if-true
            n180 = local read "stop free run"() -> (w117:bool)
            n181 = Wait Until Next ms Multiple(millisecond multiple=u32 500) -> ()  [unwired: 1 out]
            n182 = call <vilib>:"DAQmx Is Task Done.vi"("task/channels in"=w124, "error in"=w119) -> ("task out"=w123:refnum<k21>, "task done?"=w118:bool, "error out"=w121:errorcluster)  [unwired: 11 in]
            n183 = Unbundle By Name(w121) -> ("status"=w122:bool)
            n184 = Compound Arithmetic op=OR(w118, w117, w122) -> (w125:bool)
          }
          n185 = call <vilib>:"DAQmx Clear Task.vi"("task in"=w56, "error in"=w54) -> ("error out"=w45:errorcluster)  [unwired: 13 in]
          n186 = Merge Errors(w47, w45) -> (w46:errorcluster)
        }
        frame #1 {
          # "Display Error, if any."
          n187 = local write "stop free run"(FALSE ("stop 2")) -> ()
          n188 = local read "Frame Buffers Out"() -> (w305:T2[])
          n189 = local read "Avi Refnum"() -> (w304:T3)
          n190 = local read "Save Movie? 2"() -> (w300:bool)
          n191 = local read "Frame Rate"() -> (w303:cluster{i32, "camera FR":i32})
          n192 = call "Stop Video.vi"("Frame Rate(Hz)"=w303, "Save Movie?"=w300, "Trigger Type"=enum16{"Internal", "External"}."Internal", "error in"=w298, "Frame Buffers In"=w305, "Avi Refnum"=w304, "IMAQ Session In"=w299) -> ("error out"=w306:errorcluster)  [unwired: 3 in, 1 out]
          n193 = call <vilib>:"General Error Handler.vi"("[user-defined codes]"=i32[] array[5003 elements], "[user-defined descriptions]"=string[] array[5002 elements], "error in (no error)"=w306) -> ()  [unwired: 8 in, 5 out]
        }
      }
    }
    frame "calibration" {
      n194 = stacked-sequence {
        seq-local: [w321 _ _] -> [_ w713 _]
        seq-local: [w342 _ _] -> [_ w710 _]
        tunnel: w309 -> [w334 _ _]
        frame #0 {
          w310 = 0.0
          # "in pixel"
          # "para\nPx, CRx, Pdiam, Py, CRy"
          # "page, row, col\ndirection, frame, para"
          # "Initiate camera"
          n195 = local read "Cam FR (f/s)"() -> (w311:i32)
          n196 = local read "Save Frame Divisor"() -> (w339:i32)
          n197 = local read "Gain offset"() -> (w340:dbl)
          n198 = local read "Gain (dB)"() -> (w337:dbl)
          n199 = local read "Cam FR (f/s)"() -> (w332:i32)
          n200 = local write "frames captured"(w310) -> ()
          n201 = local write "counter finished"(w310) -> ()
          n202 = local read "Region of interest"() -> (w316:i32[])
          n203 = local read "Movie Directory"() -> (w338:path)
          n204 = local read "Save Movie? 3"() -> (w313:bool)
          n205 = Add(x=w337, y=w340) -> (x+y=w336:dbl)
          n206 = Bundle("Gain (dB)"=w337, w336) -> (w335:cluster{"Gain (dB)":dbl, dbl})  [unwired: 1 in]
          n207 = Quotient & Remainder(x=w332, y=w339) -> (floor(x/y)=w333:i32)  [unwired: 1 out]
          n208 = local read "Pixel value offset"() -> (w331:cluster{"Ch 1":u8, "Ch 2":u8})
          n209 = Multiply(x="clip time(s)", y=w311) -> (x*y=w343:sgl)
          n210 = To Long Integer(number=w343) -> (32bit integer=w319:i32)
          "frames/clip" <- w319
          n211 = Bundle(w333, "Cam FR (f/s)"=w332) -> (w328:cluster{i32, "Cam FR (f/s)":i32})  [unwired: 1 in]
          n212 = local write "Frame Rate"(w328) -> ()
          n213 = call "Start Video.vi"("AVI Path"=w338, "Offset"=w331, "Save Movie?"=w313, "Gain(dB)"=w335, "error in"=w334, "Frame Rate(Hz)"=w328, "Trigger Type"=enum16{"Internal", "External"}."External", "Region of interest"=w316) -> ("error out"=w314:errorcluster, "Frame Buffers Out"=w329:T2[], "Avi Refnum"=w330:T3, "IMAQ Session Out"=w315:refnum<k11>)
          n214 = local write "Frame Buffers Out"(w329) -> ()
          n215 = local write "Avi Refnum"(w330) -> ()
          n216 = call <vilib>:"Initialize Mouse.vi"() -> ("error out"=w326:errorcluster, "device ID"=w327:refnum<k1>)  [unwired: 1 in, 9 out]
          n217 = Initialize Array(0.0, w319, 5 ("dimension size")) -> (w344:dbl[][])
          n218 = stacked-sequence {
            seq-local: [w346 _ _] -> [_ _ w514]
            seq-local: [w347 _ _] -> [_ _ w517]
            tunnel: w344 -> [_ _ w525]
            tunnel: [_ _ w524] -> w342
            tunnel: w315 -> [w350 _ _]
            tunnel: w314 -> [w349 _ _]
            tunnel: w327 -> [_ _ w523]
            tunnel: w326 -> [_ _ w516]
            tunnel: [_ _ w522] -> w325
            tunnel: [_ _ w515] -> w324
            tunnel: [_ _ w513] -> w323
            tunnel: w319 -> [w348 _ w521]
            tunnel: dbl[][][] [] -> [_ _ w520]
            tunnel: w310 -> [_ _ w519]
            tunnel: [_ _ w518] -> w317
            frame #0 {
              # "Y correction"
              n219 = local read "1D or 2D cal?"() -> (w351:bool)
              n220 = case shown="True" w351 {
                tunnel: w350 -> [w353 w374]
                tunnel: w349 -> [w352 w373]
                tunnel: w348 -> [_ w384]
                tunnel: [w353 w376] -> w347
                tunnel: [w352 w375] -> w346
                frame False {
                  n221 = local write "Y correction (pixel,P-CR Y)"(0.0 ("Y correction (pixel,P-CR Y)")) -> ()
                }
                frame True {
                  # "upper-left CR"
                  # "Y correction is the y difference of \nupper and left LEDs"
                  n222 = local read "Pixel value offset"() -> (w357:cluster{"Ch 1":u8, "Ch 2":u8})
                  n223 = local read "Gain (dB)"() -> (w366:dbl)
                  n224 = local read "Gain offset"() -> (w372:dbl)
                  n225 = Unbundle By Name(w357) -> ("Ch 1"=w363:u8, "Ch 2"=w364:u8)
                  n226 = Add(x=w366, y=w372) -> (x+y=w365:dbl)
                  n227 = Number To Decimal String(number=w364) -> (decimal integer string=w362:string)  [unwired: 1 in]
                  n228 = Number To Decimal String(number=w363) -> (decimal integer string=w361:string)  [unwired: 1 in]
                  n229 = Number To Fractional String(number=w366) -> (F-format string=w371:string)  [unwired: 3 in]
                  n230 = Number To Fractional String(number=w365) -> (F-format string=w369:string)  [unwired: 3 in]
                  n231 = call <vilib>:"Space Constant.vi"() -> ("String"=w360:string)
                  n232 = call <vilib>:"Space Constant.vi"() -> ("String"=w370:string)
                  n233 = Concatenate Strings("sao " ("String to write"), "0 " ("string"), w361, w360, w362) -> (w355:string)
                  n234 = Concatenate Strings("sag " ("String to write"), "0 " ("string"), w371, w370, w369) -> (w356:string)
                  n235 = for {
                    N: 2 -> [_]
                    tunnel: w384 -> [w403]
                    tunnel: w374 -> [w402]
                    tunnel: w373 -> [w401]
                    tunnel: [w399] -> w380 mode=indexing
                    tunnel: [w398] -> w376
                    tunnel: [w397] -> w375
                    tunnel: w356 -> [w396]
                    tunnel: w355 -> [w395]
                    i -> [w400]
                    n236 = flat-sequence {
                      tunnel: w395 -> [w408]
                      tunnel: w396 -> [w409]
                      tunnel: w401 -> [w410]
                      tunnel: w402 -> [w411]
                      tunnel: w403 -> [w412]
                      tunnel: [w412] -> w389
                      tunnel: [w411] -> w388
                      tunnel: [w410] -> w387
                      tunnel: [w409] -> w386
                      tunnel: [w408] -> w385
                      tunnel: w394 -> [w404]
                      tunnel: w389 -> [w419]
                      tunnel: w388 -> [w421]
                      tunnel: w387 -> [w418]
                      tunnel: w386 -> [_]
                      tunnel: w385 -> [_]
                      tunnel: [w423] -> w393
                      tunnel: [w420] -> w392
                      tunnel: [w414] -> w391
                      tunnel: [w419] -> w390
                      tunnel: [w491] -> w397
                      tunnel: [w492] -> w398
                      tunnel: [w493] -> w399
                      tunnel: w393 -> [w493]
                      tunnel: w392 -> [w492]
                      tunnel: w391 -> [w491]
                      tunnel: w390 -> [w489]
                      frame #0 {
                        n237 = Select(t="turn on the left led" ("message"), s=w404, f="turn on the upper led") -> (s? t:f=w405:string)
                        n238 = One Button Dialog(message=w405) -> ()  [unwired: 1 in, 1 out]
                      }
                      frame #1 {
                        n239 = for {
                          N: w419 -> [_]
                          shift-right: [w428] -> w415
                          shift-left: w418 -> [w429]
                          tunnel: w421 -> [w430]
                          tunnel: [w431] -> w420
                          tunnel: [w427] -> w422 mode=indexing
                          i -> [w425]
                          n240 = local read "frames captured"() -> (w426:u64)
                          n241 = Add(x=w426, y=w425) -> (x+y=w424:u64)
                          n242 = stacked-sequence {
                            seq-local: [w433 _] -> [_ w468]
                            seq-local: [w432 _] -> [_ w482]
                            tunnel: w424 -> [w442 w467]
                            tunnel: w429 -> [w441 _]
                            tunnel: [w438 _] -> w431
                            tunnel: w430 -> [w437 _]
                            tunnel: [_ w466] -> w428
                            tunnel: [_ w465] -> w427
                            frame #0 {
                              # "digital image processing\nnot useful"
                              # "extract frames"
                              n243 = call <vilib>:"IMAQ Extract Buffer.vi"("error in (no error)"=w441, "Buffer to extract"=w442, "IMAQ Session In"=w437) -> ("error out"=w436:errorcluster, "Buffer Number"=w434:i32, "Image Out"=w439:T2, "IMAQ Session Out"=w438:refnum<k11>)  [unwired: 3 in, 2 out]
                              n244 = Not Equal?(x=w434, y=w442) -> (x != y?=w435:bool)
                              n245 = local write "Buffer Overrun"(w435) -> ()
                              n246 = local write "Buffer Number"(w434) -> ()
                              n247 = case "If overflow and taking real data, throw error" shown="True" w435 {
                                tunnel: w436 -> [w443 w445]
                                tunnel: [w443 w444] -> w440
                                frame False {
                                }
                                frame True {
                                w446 = u16 0 items=["no dialog", "OK message", "continue or stop message"] ("type of dialog (OK msg:1)")
                                # "User defined error 6500"
                                n248 = call <vilib>:"General Error Handler.vi"("[error code] (0)"=6500 ("error code (no error:0)"), "[error source] (\" \")"="Video Monitor" ("[error source] (\" \")"), "type of dialog (OK msg:1)"=w446, "error in (no error)"=w445) -> ("error out"=w444:errorcluster)  [unwired: 7 in, 4 out]
                                }
                              }
                              n249 = call "IMAQ Clear Overlay"("error in (no error)"=w440, "Image"=w439) -> ("error out"=w432:errorcluster, "Image Out"=w433:T2)  [unwired: 8 in]
                            }
                            frame #1 {
                              # "fit pupil and corneal reflection"
                              n250 = local read "Points to show"() -> (w449:enum16{"All points", "Fit points"})
                              n251 = local read "CR Bottom"() -> (w478:i32)
                              n252 = local read "CR Right"() -> (w479:i32)
                              n253 = local read "CR Top"() -> (w480:i32)
                              n254 = local read "CR Direction to keep"() -> (w476:enum16{"Above", "Below"})
                              n255 = local read "Save Frame Divisor"() -> (w469:i32)
                              n256 = local read "CR Left"() -> (w481:i32)
                              n257 = Quotient & Remainder(x=w467, y=w469) -> (x-y*floor(x/y)=w463:u64)  [unwired: 1 out]
                              n258 = Build Array(w481, w480, w479, w478) -> (w484:i32[])
                              n259 = local read "CR Fit type"() -> (w475:enum16{"Circle", "Ellipse"})
                              n260 = local read "CR Subsampling"() -> (w474:i32)
                              n261 = Equal To 0?(x=w463) -> (x = 0?=w457:bool)
                              n262 = local read "CR Threshold"() -> (w477:u8)
                              n263 = local read "Display Overlay"() -> (w458:bool)
                              n264 = call "Process Pupil or Cornea ReflectionPerc.vi"("Image In"=w468, "ROI"=w484, "Threshold"=w477, "Direction to keep"=w476, "error in (no error)"=w482, "Display"=w457, "Fit type"=w475, "Subsampling"=w474, "Color"=u32 6618880, "use % thresh"=FALSE, "Display Overlay"=w458, "Points to show"=w449) -> ("Image out"=w455:T2, "y position"=w465:dbl, "error out"=w460:errorcluster)  [unwired: 3 in, 2 out]
                              n265 = local read "P Bottom"() -> (w470:i32)
                              n266 = local read "P Right"() -> (w471:i32)
                              n267 = local read "P Top"() -> (w472:i32)
                              n268 = local read "P Direction to keep"() -> (w453:enum16{"Above", "Below"})
                              n269 = local read "P Left"() -> (w473:i32)
                              n270 = local read "P Threshold"() -> (w454:u8)
                              n271 = local read "P Fit type"() -> (w452:enum16{"Circle", "Ellipse"})
                              n272 = local read "use % thresh"() -> (w450:bool)
                              n273 = local read "P Subsampling"() -> (w451:i32)
                              n274 = Build Array(w473, w472, w471, w470) -> (w456:i32[])
                              n275 = call "Process Pupil Reflection_ovalROI2.vi"("Image In"=w455, "Threshold"=w454, "Direction to keep"=w453, "error in (no error)"=w460, "Display"=w457, "Fit type"=w452, "Global Rectangle"=w456, "Subsampling"=w451, "Color"=u32 16777215, "use % thresh"=w450, "Display Overlay"=w458, "Points to show"=w449) -> ("Image out"=w462:T2, "error out"=w461:errorcluster)  [unwired: 3 in, 3 out]
                              n276 = case shown="True" w457 {
                                tunnel: w461 -> [w485 w486]
                                tunnel: [w485 w486] -> w466
                                tunnel: w462 -> [_ w487]
                                frame False {
                                }
                                frame True {
                                n277 = local write "Image"(w487) -> ()
                                }
                              }
                            }
                          }
                        }
                        n278 = local read "clip time(s)"() -> (w417:sgl)
                        n279 = call "pulse generator for cal_training.vi"("counter freq"="Cam FR (f/s) 2", "clip length(sec)"=w417, "error in"=w418) -> ("error out"=w416:errorcluster)  [unwired: 4 in]
                        n280 = Merge Errors(w415, w416) -> (w414:errorcluster)
                        n281 = call-poly <vilib>:"Mean.vi"("X"=w422) -> ("mean"=w423:dbl)  [unwired: 1 out]
                      }
                      frame #2 {
                        n282 = local read "frames captured"() -> (w490:u64)
                        n283 = Add(x=w490, y=w489) -> (x+y=w488:u64)
                        n284 = local write "frames captured"(w488) -> ()
                      }
                    }
                    n285 = Equal To 0?(x=w400) -> (x = 0?=w394:bool)
                  }
                  n286 = Index Array(array=w380, index=1) -> (element=w381:dbl)
                  n287 = Index Array(array=w380, index=0) -> (element=w378:dbl)
                  n288 = Subtract(x=w381, y=w378) -> (x-y=w377:dbl)
                  n289 = local write "Y correction (pixel,P-CR Y)"(w377) -> ()
                }
              }
            }
            frame #1 {
              n290 = One Button Dialog(message="Press right button to do one measurement;\nand press stop to finish") -> ()  [unwired: 1 in, 1 out]
            }
            frame #2 {
              n291 = local read "Pixel value offset"() -> (w496:cluster{"Ch 1":u8, "Ch 2":u8})
              n292 = local read "Gain offset"() -> (w512:dbl)
              n293 = local read "Gain (dB)"() -> (w506:dbl)
              n294 = Unbundle By Name(w496) -> ("Ch 1"=w502:u8, "Ch 2"=w503:u8)
              n295 = Add(x=w506, y=w512) -> (x+y=w505:dbl)
              n296 = Number To Decimal String(number=w503) -> (decimal integer string=w501:string)  [unwired: 1 in]
              n297 = Number To Decimal String(number=w502) -> (decimal integer string=w500:string)  [unwired: 1 in]
              n298 = Number To Fractional String(number=w506) -> (F-format string=w511:string)  [unwired: 3 in]
              n299 = Number To Fractional String(number=w505) -> (F-format string=w509:string)  [unwired: 3 in]
              n300 = call <vilib>:"Space Constant.vi"() -> ("String"=w499:string)
              n301 = call <vilib>:"Space Constant.vi"() -> ("String"=w510:string)
              n302 = Concatenate Strings("sao " ("String to write"), "0 " ("string"), w500, w499, w501) -> (w495:string)
              n303 = Concatenate Strings("sag " ("String to write"), "0 " ("string"), w511, w510, w509) -> (w504:string)
              n304 = while {
                tunnel: w525 -> [w549]
                tunnel: w521 -> [w547]
                tunnel: [w545] -> w524
                tunnel: w517 -> [w548]
                tunnel: w523 -> [w546]
                tunnel: [w530] -> w522
                shift-right: [w540] -> w518
                shift-left: w520 -> [w541]
                shift-right: [w533] -> _
                shift-left: w519 -> [w534]
                shift-right: [w528] -> w515
                shift-left: w516 -> [w539]
                shift-right: [w537] -> w513
                shift-left: w514 -> [w538]
                tunnel: w504 -> [w527]
                tunnel: w495 -> [w526]
                stop <- w542 stop-if-true
                n305 = call-poly <vilib>:"Acquire Input Data.vi"("device ID"=w546, "error in (no error)"=w539) -> ("device ID"=w531:refnum<k1>, "button info"=w536:T13, "error out"=w529:errorcluster)  [unwired: 1 in, 14 out]
                n306 = Unbundle By Name(w536) -> ("button 2"=w535:bool)
                n307 = case shown="True" w535 {
                  tunnel: w549 -> [_ w584]
                  tunnel: [w556 w583] -> w545
                  tunnel: [w555 w582] -> w537
                  tunnel: w548 -> [w556 w560]
                  tunnel: w538 -> [w555 w559]
                  tunnel: w547 -> [_ w581]
                  tunnel: w541 -> [w554 w580]
                  tunnel: [w554 w579] -> w540
                  tunnel: w534 -> [w553 w569]
                  tunnel: [w553 w575] -> w533
                  tunnel: w531 -> [w552 w567]
                  tunnel: [w552 w562] -> w530
                  tunnel: w529 -> [w551 w564]
                  tunnel: [w551 w561] -> w528
                  tunnel: w527 -> [_ _]
                  tunnel: w526 -> [_ _]
                  frame False {
                    n308 = Wait Until Next ms Multiple(millisecond multiple=u32 100) -> ()  [unwired: 1 out]
                  }
                  frame True {
                    n309 = flat-sequence {
                      tunnel: [w600] -> w578
                      tunnel: [w586] -> w577
                      tunnel: [w596] -> w576
                      tunnel: [w595] -> w570
                      tunnel: [w594] -> w568
                      tunnel: [w593] -> w565
                      tunnel: [w592] -> w557
                      tunnel: w584 -> [w601]
                      tunnel: w560 -> [w599]
                      tunnel: w559 -> [w591]
                      tunnel: w581 -> [w592]
                      tunnel: w580 -> [w597]
                      tunnel: w569 -> [w595]
                      tunnel: w567 -> [w594]
                      tunnel: w564 -> [w593]
                      tunnel: w578 -> [w678]
                      tunnel: w577 -> [w677]
                      tunnel: w576 -> [w687]
                      tunnel: [w678] -> w574
                      tunnel: [w677] -> w573
                      tunnel: [w687] -> w572
                      tunnel: [w682] -> w571
                      tunnel: w570 -> [w681]
                      tunnel: w568 -> [w680]
                      tunnel: [w680] -> w566
                      tunnel: w565 -> [w679]
                      tunnel: [w679] -> w563
                      tunnel: [w676] -> w558
                      tunnel: w557 -> [w676]
                      tunnel: [w695] -> w575
                      tunnel: [w696] -> w579
                      tunnel: [w697] -> w582
                      tunnel: [w698] -> w583
                      tunnel: w574 -> [w698]
                      tunnel: w573 -> [w697]
                      tunnel: w572 -> [w696]
                      tunnel: w571 -> [w695]
                      tunnel: w566 -> [w694]
                      tunnel: w563 -> [w692]
                      tunnel: [w693] -> w562
                      tunnel: [w691] -> w561
                      tunnel: w558 -> [w689]
                      frame #0 {
                        n310 = for {
                          N: w592 -> [_]
                          shift-right: [w608] -> w588
                          shift-left: w591 -> [w606]
                          shift-right: [w605] -> w598
                          shift-left: w601 -> [w610]
                          tunnel: w599 -> [w607]
                          tunnel: [w609] -> w600
                          i -> [w602]
                          n311 = local read "frames captured"() -> (w604:u64)
                          n312 = Add(x=w604, y=w602) -> (x+y=w603:u64)
                          n313 = stacked-sequence {
                            seq-local: [w612 _] -> [_ w652]
                            seq-local: [w611 _] -> [_ w666]
                            tunnel: w603 -> [w621 w649]
                            tunnel: w606 -> [w620 _]
                            tunnel: [w617 _] -> w609
                            tunnel: w610 -> [_ w648]
                            tunnel: [_ w647] -> w608
                            tunnel: w607 -> [w616 _]
                            tunnel: [_ w651] -> w605
                            tunnel: w602 -> [_ w645]
                            frame #0 {
                              # "digital image processing"
                              # "extract frames"
                              n314 = call <vilib>:"IMAQ Extract Buffer.vi"("error in (no error)"=w620, "Buffer to extract"=w621, "IMAQ Session In"=w616) -> ("error out"=w615:errorcluster, "Buffer Number"=w613:i32, "Image Out"=w618:T2, "IMAQ Session Out"=w617:refnum<k11>)  [unwired: 3 in, 2 out]
                              n315 = local write "Buffer Number"(w613) -> ()
                              n316 = Not Equal?(x=w613, y=w621) -> (x != y?=w614:bool)
                              n317 = local write "Buffer Overrun"(w614) -> ()
                              n318 = case "If overflow and taking real data, throw error" shown="True" w614 {
                                tunnel: w615 -> [w622 w624]
                                tunnel: [w622 w623] -> w619
                                frame False {
                                }
                                frame True {
                                w625 = u16 0 items=["no dialog", "OK message", "continue or stop message"] ("type of dialog (OK msg:1)")
                                # "User defined error 6500"
                                n319 = call <vilib>:"General Error Handler.vi"("[error code] (0)"=6500 ("error code (no error:0)"), "[error source] (\" \")"="Video Monitor" ("[error source] (\" \")"), "type of dialog (OK msg:1)"=w625, "error in (no error)"=w624) -> ("error out"=w623:errorcluster)  [unwired: 7 in, 4 out]
                                }
                              }
                              n320 = call "IMAQ Clear Overlay"("error in (no error)"=w619, "Image"=w618) -> ("error out"=w611:errorcluster, "Image Out"=w612:T2)  [unwired: 8 in]
                            }
                            frame #1 {
                              # "each col contains one parameters"
                              # "fit pupil and corneal reflection"
                              n321 = local read "CR Right"() -> (w663:i32)
                              n322 = local read "Points to show"() -> (w628:enum16{"All points", "Fit points"})
                              n323 = local read "CR Bottom"() -> (w662:i32)
                              n324 = local read "CR Top"() -> (w664:i32)
                              n325 = local read "CR Direction to keep"() -> (w660:enum16{"Above", "Below"})
                              n326 = local read "CR Left"() -> (w665:i32)
                              n327 = local read "Save Frame Divisor"() -> (w653:i32)
                              n328 = Build Array(w665, w664, w663, w662) -> (w668:i32[])
                              n329 = local read "CR Fit type"() -> (w659:enum16{"Circle", "Ellipse"})
                              n330 = local read "CR Subsampling"() -> (w658:i32)
                              n331 = local read "CR Threshold"() -> (w661:u8)
                              n332 = Quotient & Remainder(x=w649, y=w653) -> (x-y*floor(x/y)=w672:u64)  [unwired: 1 out]
                              n333 = local read "Display Overlay"() -> (w639:bool)
                              n334 = Equal?(x=w672, y=0) -> (x = y?=w636:bool)
                              n335 = call "Process Pupil or Cornea ReflectionPerc.vi"("Image In"=w652, "ROI"=w668, "Threshold"=w661, "Direction to keep"=w660, "error in (no error)"=w666, "Display"=w636, "Fit type"=w659, "Subsampling"=w658, "Color"=u32 6618880, "use % thresh"=FALSE, "Display Overlay"=w639, "Points to show"=w628) -> ("Image out"=w635:T2, "x position"=w670:dbl, "y position"=w669:dbl, "error out"=w634:errorcluster)  [unwired: 3 in, 1 out]
                              n336 = local read "P Bottom"() -> (w654:i32)
                              n337 = local read "P Right"() -> (w655:i32)
                              n338 = local read "P Top"() -> (w656:i32)
                              n339 = local read "P Direction to keep"() -> (w632:enum16{"Above", "Below"})
                              n340 = local read "P Left"() -> (w657:i32)
                              n341 = local read "P Threshold"() -> (w633:u8)
                              n342 = local read "P Fit type"() -> (w631:enum16{"Circle", "Ellipse"})
                              n343 = local read "P Subsampling"() -> (w630:i32)
                              n344 = Build Array(w657, w656, w655, w654) -> (w637:i32[])
                              n345 = local read "use % thresh"() -> (w629:bool)
                              n346 = call "Process Pupil Reflection_ovalROI2.vi"("Image In"=w635, "Threshold"=w633, "Direction to keep"=w632, "error in (no error)"=w634, "Display"=w636, "Fit type"=w631, "Global Rectangle"=w637, "Subsampling"=w630, "Color"=u32 16777215, "use % thresh"=w629, "Display Overlay"=w639, "Points to show"=w628) -> ("Image out"=w641:T2, "x position"=w642:dbl, "y position"=w644:dbl, "diameter"=w643:dbl, "error out"=w640:errorcluster)  [unwired: 3 in]
                              n347 = case shown="True" w636 {
                                tunnel: w640 -> [w673 w674]
                                tunnel: [w673 w674] -> w647
                                tunnel: w641 -> [_ w675]
                                frame False {
                                }
                                frame True {
                                n348 = local write "Image"(w675) -> ()
                                }
                              }
                              n349 = Build Array(w642, w670, w643, w644, w669) -> (w650:dbl[])
                              n350 = Replace Array Subset(array=w648, new element=w650, index (row)=w645) -> (w651:dbl[][])  [unwired: 1 in]
                            }
                          }
                        }
                        n351 = local read "Cam FR (f/s)"() -> (w590:i32)
                        n352 = local read "clip time(s)"() -> (w589:sgl)
                        n353 = call "pulse generator for cal_training.vi"("counter freq"=w590, "clip length(sec)"=w589, "error in"=w591, "counter"="counter") -> ("error out"=w587:errorcluster)  [unwired: 3 in]
                        n354 = Merge Errors(w588, w587) -> (w586:errorcluster)
                        n355 = Build Array (concatenate)(w597, w598) -> (w596:dbl[][][])
                      }
                      frame #1 {
                        n356 = Increment(x=w681) -> (x+1=w682:dbl)
                        n357 = local read "L/R?"() -> (w683:bool)
                        n358 = Divide(x=w682, y=2.0) -> (x/y=w686:dbl)
                        n359 = local write "counter finished"(w686) -> ()
                        n360 = Not(x=w683) -> (.not. x?=w684:bool)
                        n361 = local write "L/R?"(w684) -> ()
                      }
                      frame #2 {
                        # "stall here before \nreleasing button"
                        n362 = local read "frames captured"() -> (w690:u64)
                        n363 = while {
                          tunnel: w694 -> [w705]
                          tunnel: [w704] -> w693
                          shift-right: [w702] -> w691
                          shift-left: w692 -> [w703]
                          stop <- w700 continue-if-true
                          w699 = u32 20  # Loop Time (ms)
                          n364 = call-poly <vilib>:"Acquire Input Data.vi"("device ID"=w705, "error in (no error)"=w703) -> ("device ID"=w704:refnum<k1>, "button info"=w701:T13, "error out"=w702:errorcluster)  [unwired: 1 in, 14 out]
                          n365 = Unbundle By Name(w701) -> ("button 2"=w700:bool)
                          n366 = Wait (ms)(milliseconds to wait=w699) -> ()  [unwired: 1 out]
                        }
                        n367 = Add(x=w689, y=w690) -> (x+y=w688:u64)
                        n368 = local write "frames captured"(w688) -> ()
                      }
                    }
                  }
                }
                n369 = Unbundle By Name(w528) -> ("status"=w532:bool)
                n370 = Unbundle By Name(w537) -> ("status"=w544:bool)
                n371 = Compound Arithmetic op=OR(w544, "stop calib", w532) -> (w542:bool)
              }
            }
          }
          n372 = local write "calib data"(w317) -> ()
          n373 = call-poly <vilib>:"Close Input Device.vi"("error in (no error)"=w324, "device ID"=w325) -> ("error out"=w322:errorcluster)  [unwired: 8 out]
          n374 = Merge Errors(w323, w322) -> (w321:errorcluster)
        }
        frame #1 {
          # "Display Error, if any."
          n375 = local read "Frame Buffers Out"() -> (w712:T2[])
          n376 = local read "Avi Refnum"() -> (w711:T3)
          n377 = local read "Save Movie? 3"() -> (w706:bool)
          n378 = local read "Frame Rate"() -> (w709:cluster{i32, "camera FR":i32})
          n379 = call "Stop Video.vi"("Frame Rate(Hz)"=w709, "Save Movie?"=w706, "Trigger Type"=enum16{"Internal", "External"}."Internal", "error in"=w713, "Frame Buffers In"=w712, "Avi Refnum"=w711, "IMAQ Session In"=w710) -> ("error out"=w714:errorcluster)  [unwired: 3 in, 1 out]
          n380 = call <vilib>:"General Error Handler.vi"("[user-defined codes]"=i32[] array[5003 elements], "[user-defined descriptions]"=string[] array[5002 elements], "error in (no error)"=w714) -> ()  [unwired: 8 in, 5 out]
          n381 = local write "stop calib"(FALSE ("stop calib")) -> ()
        }
        frame #2 {
          # "in mm"
          # "upper-left CR"
          # "Y correction is the y difference of \nupper and left LEDs"
          # "page, row, col\ndirection, frame, para"
          # "para\nPx, CRx, Pdiam, Py, CRy"
          # "in mm"
          # "need to save calibration paras, including Y correction"
          # "(P-CR2)-(P-CR1)   1: above; 2: left\n=(CR1-CR2)"
          # "left-right 10deg"
          # "in pixel"
          # "para\nPx, CRx, Pdiam, Py, CRy"
          # "page, row, col\ndirection, frame, para"
          # "caculate and fit Rp vs pupil diameter"
          n382 = Divide(x=10.0, y=180.0) -> (x/y=w744:dbl)
          n383 = Multiply(x=w744, y=3.141592653589793) -> (x*y=w745:dbl)
          n384 = local read "conversion factor"() -> (w735:cluster{"x":dbl, "y":dbl})
          n385 = local read "counter finished"() -> (w749:sgl)
          n386 = Sine(x=w745) -> (sin(x)=w746:dbl)
          n387 = local read "Y correction (pixel,P-CR Y)"() -> (w736:dbl)
          n388 = local read "calib data"() -> (w723:dbl[][][])
          n389 = Round Toward -Infinity(1:w749) -> (0:w748:sgl)
          n390 = Unbundle By Name(w735) -> ("x"=w734:dbl, "y"=w733:dbl)
          n391 = Multiply(x=w746, y=2.0) -> (x*y=w741:dbl)
          n392 = Delete From Array(array=w723, length=4, index (dim 1)=0 ("disabled index (row)")) -> (array with subset deleted=w722:dbl[][][])  [unwired: 2 in, 1 out]
          n393 = for {
            N: w748 -> [_]
            tunnel: w722 -> [w893]
            tunnel: w741 -> [w877]
            tunnel: [w863] -> w717 mode=indexing
            tunnel: [w869] -> w732 mode=indexing
            tunnel: [w868] -> w719 mode=indexing
            tunnel: w736 -> [w867]
            tunnel: w734 -> [w866]
            tunnel: w733 -> [w865]
            i -> [w891]
            # "(P-CR2)-(P-CR1)   1: above; 2: left\n=(CR1-CR2)"
            # "(P-CR2)"
            # "(P-CR1)"
            # "2 dir"
            # "1 dir"
            # "make sure this sign is right"
            # "signs depend on the direction of Y correction"
            # "Rp in pixel"
            # "Diameter"
            # "opposite direction"
            # "one direction"
            # "opposite direction"
            # "one direction"
            # "Pupil Position - Cornea Reflection Y"
            # "Pupil Position - Cornea Reflection X"
            n394 = Multiply(x=w891, y=2) -> (x*y=w907:i32)
            n395 = Multiply(x=w891, y=2) -> (x*y=w894:i32)
            n396 = Multiply(x=w891, y=2) -> (x*y=w920:i32)
            n397 = Increment(x=w907) -> (x+1=w903:i32)
            n398 = Increment(x=w920) -> (x+1=w916:i32)
            n399 = Increment(x=w894) -> (x+1=w892:i32)
            n400 = Index Array(array=w893, index (dim 0) #1=w907, index (dim 2) #1=3 ("disabled index (col)"), index (dim 0) #2=w907, index (dim 2) #2=4 ("disabled index (col)"), index (dim 0) #3=w903, index (dim 2) #3=3 ("disabled index (col)"), index (dim 0) #4=w903, index (dim 2) #4=4 ("disabled index (col)")) -> (element #1=w906:dbl[], element #2=w905:dbl[], element #3=w899:dbl[], element #4=w898:dbl[])  [unwired: 4 in]
            n401 = Index Array(array=w893, index (dim 0) #1=w894, index (dim 2) #1=2 ("disabled index (col)"), index (dim 0) #2=w892, index (dim 2) #2=2 ("disabled index (col)")) -> (element #1=w890:dbl[], element #2=w889:dbl[])  [unwired: 2 in]
            n402 = Index Array(array=w893, index (dim 0) #1=w920, index (dim 2) #1=0 ("disabled index (col)"), index (dim 0) #2=w920, index (dim 2) #2=1 ("disabled index (col)"), index (dim 0) #3=w916, index (dim 2) #3=0 ("disabled index (col)"), index (dim 0) #4=w916, index (dim 2) #4=1 ("disabled index (col)")) -> (element #1=w919:dbl[], element #2=w918:dbl[], element #3=w912:dbl[], element #4=w911:dbl[])  [unwired: 4 in]
            n403 = Subtract(x=w906, y=w905) -> (x-y=w904:dbl[])
            n404 = Subtract(x=w899, y=w898) -> (x-y=w900:dbl[])
            n405 = Subtract(x=w919, y=w918) -> (x-y=w917:dbl[])
            n406 = Subtract(x=w912, y=w911) -> (x-y=w913:dbl[])
            n407 = call-poly <vilib>:"Mean.vi"("X"=w889) -> ("mean"=w886:dbl)  [unwired: 1 out]
            n408 = call-poly <vilib>:"Mean.vi"("X"=w890) -> ("mean"=w887:dbl)  [unwired: 1 out]
            n409 = call-poly <vilib>:"Mean.vi"("X"=w904) -> ("mean"=w882:dbl)  [unwired: 1 out]
            n410 = call-poly <vilib>:"Mean.vi"("X"=w900) -> ("mean"=w881:dbl)  [unwired: 1 out]
            n411 = call-poly <vilib>:"Mean.vi"("X"=w917) -> ("mean"=w880:dbl)  [unwired: 1 out]
            n412 = call-poly <vilib>:"Mean.vi"("X"=w913) -> ("mean"=w879:dbl)  [unwired: 1 out]
            n413 = Add(x=w887, y=w886) -> (x+y=w888:dbl)
            n414 = Add(x=w882, y=w881) -> (x+y=w884:dbl)
            n415 = Divide(x=w888, y=2.0) -> (x/y=w873:dbl)
            n416 = Subtract(x=w880, y=w879) -> (x-y=w878:dbl)
            n417 = Divide(x=w884, y=2.0) -> (x/y=w876:dbl)
            n418 = Divide(x=w878, y=w877) -> (x/y=w875:dbl)
            n419 = Multiply(x=w866, y=w875) -> (x*y=w864:dbl)
            n420 = Add(x=w876, y=w867) -> (x+y=w874:dbl)
            n421 = Multiply(x=w865, y=w874) -> (x*y=w869:dbl)
            n422 = Add(x=w866, y=w865) -> (x+y=w872:dbl)
            n423 = Divide(x=w872, y=2.0) -> (x/y=w870:dbl)
            n424 = Multiply(x=w870, y=w873) -> (x*y=w868:dbl)
            n425 = Absolute Value(x=w864) -> (abs(x)=w863:dbl)
          }
          "Rp" <- w717
          "Diameters" <- w719
          n426 = Square(x=w732) -> (x^2=w738:dbl[])
          n427 = Square(x=w717) -> (x^2=w739:dbl[])
          n428 = Add(x=w739, y=w738) -> (x+y=w737:dbl[])
          n429 = Square Root(x=w737) -> (sqrt(x)=w718:dbl[])
          "Rp0s" <- w718
          n430 = while {
            tunnel: w717 -> [w762]
            tunnel: w718 -> [w761]
            tunnel: w719 -> [w760]
            tunnel: [w759] -> w731
            tunnel: [w758] -> w730
            tunnel: [w757] -> w729
            tunnel: [w756] -> w728
            tunnel: [w755] -> w727
            tunnel: [w754] -> w726
            tunnel: [w753] -> w725
            tunnel: [w752] -> w724
            stop <- "stop 2" stop-if-true
            # "in mm"
            n431 = call "XY Fit.vi"("Outlier Cutoff"="Outlier Cutoff_Rp0s(2D)", "X Values"=w760, "Y Values"=w761) -> ("slope"=w755:dbl, "intercept"=w754:dbl, "R-square"=w753:dbl, "mean"=w752:dbl, "XY Graph"=→"Rp0s vs Pupil":cluster{dbl[], dbl[]}[])  [unwired: 8 in]
            n432 = Wait Until Next ms Multiple(millisecond multiple=u32 500 ("milliseconds to wait")) -> ()  [unwired: 1 out]
            n433 = call "XY Fit.vi"("Outlier Cutoff"="Outlier Cutoff_Rp(1D)", "X Values"=w760, "Y Values"=w762) -> ("slope"=w759:dbl, "intercept"=w758:dbl, "R-square"=w757:dbl, "mean"=w756:dbl, "XY Graph"=→"Rp vs Pupil":cluster{dbl[], dbl[]}[])  [unwired: 8 in]
            n434 = local write "intercept_Rp0s"(w754) -> ()
            n435 = local write "intercept_Rp"(w758) -> ()
            n436 = local write "average_Rp"(w756) -> ()
            n437 = local write "slope_Rp0s"(w755) -> ()
            n438 = local write "slope_Rp"(w759) -> ()
            n439 = local write "R-squared_Rp"(w757) -> ()
            n440 = local write "R-squared_Rp0s"(w753) -> ()
            n441 = local write "average_Rp0s"(w752) -> ()
          }
          n442 = stacked-sequence {
            tunnel: w731 -> [_ w844]
            tunnel: w730 -> [_ w843]
            tunnel: w729 -> [_ w842]
            tunnel: w728 -> [_ w841]
            tunnel: w727 -> [_ w840]
            tunnel: w726 -> [_ w839]
            tunnel: w725 -> [_ w838]
            tunnel: w724 -> [_ w837]
            tunnel: w719 -> [_ w810]
            tunnel: w718 -> [_ w808]
            tunnel: w717 -> [_ w806]
            frame #0 {
              n443 = while {
                tunnel: [w775] -> w767
                stop <- w774 continue-if-true
                (unwired) "/"
                w797 = "/"
                n444 = Get Date/Time String() -> (date string=w799:string)  [unwired: 3 in, 1 out]
                n445 = Match Pattern(string=w799, regular expression=w797) -> (before substring=w796:string, after substring=w798:string)  [unwired: 1 in, 2 out]
                n446 = Wait (ms)(milliseconds to wait=u32 100) -> ()  [unwired: 1 out]
                n447 = Match Pattern(string=w798, regular expression=w797) -> (before substring=w795:string, after substring=w784:string)  [unwired: 1 in, 2 out]
                n448 = local read "saving disk"() -> (w770:string)
                n449 = Decimal String To Number(string=w796) -> (number=w790:i32)  [unwired: 2 in, 1 out]
                n450 = Decimal String To Number(string=w795) -> (number=w787:i32)  [unwired: 2 in, 1 out]
                n451 = String Subset(string=w784, offset (0)=2) -> (substring=w780:string)  [unwired: 1 in]
                n452 = Number To Decimal String(number=w790, width (-)=i16 2) -> (decimal integer string=w793:string)
                n453 = Number To Decimal String(number=w787, width (-)=i16 2) -> (decimal integer string=w789:string)
                n454 = call <vilib>:"Space Constant.vi"() -> ("String"=w792:string)
                n455 = local read "file subname"() -> (w771:string)
                n456 = call <vilib>:"Space Constant.vi"() -> ("String"=w788:string)
                n457 = Search and Replace String(input string=w793, search string=w792, replace string="0" ("replace string (\"\")")) -> (result string=w782:string)  [unwired: 5 in, 3 out]
                n458 = Search and Replace String(input string=w789, search string=w788, replace string="0" ("replace string (\"\")")) -> (result string=w781:string)  [unwired: 5 in, 3 out]
                n459 = Concatenate Strings(w782, w781, w780) -> (w772:string)
                n460 = local read "ver"() -> (w768:string)
                n461 = Concatenate Strings(w770, "cal\\" ("string"), w768, "cal" ("string"), w772, "_" ("string"), w771, ".cal" ("string")) -> (w777:string)
                n462 = String To Path(string=w777) -> (path=w776:path)
                n463 = call <vilib>:"Check if File or Folder Exists.vi"("path"=w776) -> ("file or folder exists?"=w774:bool, "dup path"=w775:path)  [unwired: 8 in, 1 out]
                n464 = case shown="False" w774 {
                  frame False {
                    n465 = local write "Info String"("valid file name" ("String")) -> ()
                  }
                  frame True {
                    n466 = local write "Info String"("rename file" ("String")) -> ()
                  }
                }
              }
              n467 = local write "calib para file to load"(w767) -> ()
              n468 = local write "calib para file path"(w767) -> ()
            }
            frame #1 {
              w803 = "      "
              w804 = "%f" ("format string")
              w812 = "\r"
              w811 = "      "
              n469 = local read "1D or 2D cal?"() -> (w821:bool)
              n470 = local read "Change pupil size?"() -> (w818:bool)
              n471 = local read "Y correction (pixel,P-CR Y)"() -> (w836:dbl)
              n472 = local read "counter finished"() -> (w835:sgl)
              n473 = local read "calib para file path"() -> (w823:path)
              n474 = Boolean To (0,1)(Boolean=w821) -> (0, 1=w820:i16)
              n475 = call <vilib>:"Check if File or Folder Exists.vi"("path"=w823) -> ("error out"=w847:errorcluster, "file or folder exists?"=w845:bool, "dup path"=w846:path)  [unwired: 8 in]
              n476 = Boolean To (0,1)(Boolean=w818) -> (0, 1=w817:i16)
              n477 = Number To Fractional String(number=w844) -> (F-format string=w834:string)  [unwired: 3 in]
              n478 = Number To Fractional String(number=w843) -> (F-format string=w833:string)  [unwired: 3 in]
              n479 = Number To Fractional String(number=w842) -> (F-format string=w832:string)  [unwired: 3 in]
              n480 = Number To Fractional String(number=w841) -> (F-format string=w831:string)  [unwired: 3 in]
              n481 = case shown="False" w845 {
                tunnel: [w857 ""] -> w822
                frame False {
                  n482 = Concatenate Strings("Slope_Rp     Intercept_Rp     R2_Rp       Ave_Rp       ", "Slope_Rp0s   Intercept_Rp0s   R2_Rp0s     Ave_Rp0s     ", "Y-correction     counter     1D_or_2D     change_pupil_size", "\r") -> (w857:string)
                }
                frame True {
                }
              }
              n483 = Number To Fractional String(number=w840) -> (F-format string=w830:string)  [unwired: 3 in]
              n484 = Number To Fractional String(number=w839) -> (F-format string=w829:string)  [unwired: 3 in]
              n485 = Number To Fractional String(number=w838) -> (F-format string=w828:string)  [unwired: 3 in]
              n486 = Number To Fractional String(number=w837) -> (F-format string=w827:string)  [unwired: 3 in]
              n487 = Number To Fractional String(number=w820) -> (F-format string=w819:string)  [unwired: 3 in]
              n488 = Number To Fractional String(number=w836) -> (F-format string=w826:string)  [unwired: 3 in]
              n489 = Number To Fractional String(number=w835) -> (F-format string=w825:string)  [unwired: 3 in]
              n490 = Array To Spreadsheet String(delimiter (Tab)=w803, array=w808, 3:w804) -> (spreadsheet string=w807:string)
              n491 = Array To Spreadsheet String(delimiter (Tab)=w803, array=w806, 3:w804) -> (spreadsheet string=w805:string)
              n492 = Array To Spreadsheet String(delimiter (Tab)=w803, array=w810, 3:w804) -> (spreadsheet string=w809:string)
              n493 = Number To Fractional String(number=w817) -> (F-format string=w816:string)  [unwired: 3 in]
              n494 = Open/Create/Replace File(file path (use dialog)=w846, error in=w847, operation (0:open)=T7."open or create") -> (refnum out=w855:refnum<file>, error out=w854:errorcluster)  [unwired: 3 in, 1 out]
              n495 = Set File Position(offset (in bytes) (0)=i64 0, refnum=w855, from (0:start)=enum16{"start", "end", "current"}."end", error in=w854) -> (refnum out=w851:refnum<file>, error out=w850:errorcluster)
              n496 = Concatenate Strings(w822, w834, w811, w833, w811, w832, w811, w831, w811, w830, w811, w829, w811, w828, w811, w827, w811, w826, w811, w825, w811, w819, w811, w816, w812, "pupil_diam" ("string"), w812, w809, w812, "Rp0s" ("string"), w812, w807, w812, "Rp" ("string"), w812, w805, w812) -> (w824:string)
              n497 = Write to Text File(file (use dialog)=w851, text=w824, error in=w850) -> (refnum out=w849:refnum<file>, error out=w848:errorcluster)  [unwired: 1 in, 1 out]
              n498 = Close File(refnum=w849, error in=w848) -> ()  [unwired: 2 out]
            }
          }
        }
      }
    }
    frame "measure" {
      n499 = local read "talk to VS"() -> (w924:bool)
      n500 = case shown="False" w924 {
        tunnel: [w1917 w1918] -> w938
        tunnel: [w1916 _] -> w937
        tunnel: w936 -> [w1912 w1918]
        tunnel: [w1911 _] -> w933
        tunnel: [w1910 _] -> w932
        frame True {
          # "This line is used to communicate with\nthe VS computer to send out eye \ncoordinates"
          # "This line is used to establish UDP \ncommunication with the VS computer\nto send start signal after camera initiation"
          # "establish UDP"
          n501 = local read "Local IP_tracker"() -> (w1914:string)
          n502 = local read "L Port com"() -> (w1915:u16)
          n503 = local read "L Port data"() -> (w1913:u16)
          n504 = String To IP(1:w1914) -> (0:w1909:u32)
          n505 = UDP Open(7:w1909, 11:w1913) -> (port=w1911:refnum<k16>, 0:w1910:errorcluster)  [unwired: 1 in, 3 out]
          n506 = UDP Open(7:w1909, 8:w1912, 11:w1915) -> (port=w1916:refnum<k16>, 0:w1917:errorcluster)  [unwired: 3 out]
        }
        frame False {
          # "no udp comm"
        }
      }
      n507 = stacked-sequence {
        tunnel: w938 -> [_ w950 _]
        tunnel: w937 -> [_ w949 _]
        tunnel: [_ w948 _] -> w935
        tunnel: [_ w947 _] -> w934
        tunnel: w933 -> [_ w946 _]
        tunnel: w932 -> [_ w945 _]
        tunnel: [_ w944 _] -> w931
        tunnel: [_ w943 _] -> w930
        tunnel: [_ w942 _] -> w926
        frame #0 {
          n508 = flat-sequence {
            frame #0 {
              w941 = T6."Enabled" ("Disabled")
              n509 = global write "Global 1.vi" "global stop"(FALSE ("global stop")) -> ()
              n510 = property on="stop program" class="Bool (strict)"("DisabledEnum"=w941) -> ()  [unwired: 2 in, 2 out]
              n511 = property on="Start session" class="Bool (strict)"("DisabledEnum"=w941) -> ()  [unwired: 2 in, 2 out]
              n512 = property on="End session and save" class="Bool (strict)"("DisabledEnum"=T6."Disabled and Grayed Out" ("Disabled")) -> ()  [unwired: 2 in, 2 out]
            }
          }
        }
        frame #1 {
          n513 = while {
            tunnel: w950 -> [w961]
            tunnel: w949 -> [w960]
            tunnel: [w959] -> w948
            tunnel: [w958] -> w947
            tunnel: w946 -> [w955]
            tunnel: w945 -> [w954]
            tunnel: [w953] -> w944
            tunnel: [w952] -> w943
            tunnel: [w951] -> w942
            stop <- w956 stop-if-true
            n514 = local read "Start session"() -> (w957:bool)
            n515 = case shown="True" w957 {
              tunnel: w961 -> [w962 w977]
              tunnel: w960 -> [w963 w976]
              tunnel: [w962 w975] -> w959
              tunnel: [w963 w974] -> w958
              tunnel: [w964 FALSE] -> w956
              tunnel: w955 -> [w966 w972]
              tunnel: w954 -> [w965 w971]
              tunnel: [w966 w970] -> w953
              tunnel: [w965 w969] -> w952
              tunnel: [_ w968] -> w951
              frame False {
                n516 = Wait (ms)(milliseconds to wait=u32 100) -> ()  [unwired: 1 out]
                n517 = local read "stop program"() -> (w964:bool)
              }
              frame True {
                # "frame trial"
                # "# for eyedata"
                # "eye ROI hist"
                n518 = stacked-sequence {
                  seq-local: [_ _ w1067 _ _ _] -> [_ _ _ w1237 w1771 _]
                  seq-local: [_ _ _ w1233 _ _] -> [_ _ _ _ w1774 _]
                  seq-local: [_ _ w1066 _ _ _] -> [_ _ _ w1241 w1773 _]
                  seq-local: [_ _ w1065 _ _ _] -> [_ _ _ w1240 w1772 _]
                  seq-local: [_ _ w1061 _ _ _] -> [_ _ _ w1222 _ _]
                  seq-local: [_ _ w1064 _ _ _] -> [_ _ _ w1232 w1767 _]
                  seq-local: [_ _ _ w1226 _ _] -> [_ _ _ _ w1768 _]
                  seq-local: [_ _ _ w1225 _ _] -> [_ _ _ _ w1770 _]
                  seq-local: [_ _ _ w1223 _ _] -> [_ _ _ _ w1769 _]
                  tunnel: w976 -> [_ _ _ w1239 _ _]
                  tunnel: w977 -> [_ _ _ w1238 _ _]
                  tunnel: [_ _ _ w1234 _ _] -> w974
                  tunnel: [_ _ _ w1235 _ _] -> w975
                  tunnel: w972 -> [_ _ _ w1231 _ _]
                  tunnel: w971 -> [_ _ _ w1230 _ _]
                  tunnel: [_ _ _ w1229 _ _] -> w970
                  tunnel: [_ _ _ w1228 _ _] -> w969
                  tunnel: [_ _ _ w1220 _ _] -> w968
                  frame #0 {
                    # "input calibration parameters"
                    n519 = stacked-sequence {
                      frame #0 {
                        n520 = case shown="True" "input cal para from file?" {
                          frame False {
                          }
                          frame True {
                            # "read the line of parameter names"
                            # "input calibration parameters from file"
                            # "read the values of parameters"
                            n521 = local read "calib para file to load"() -> (w992:path)
                            n522 = call <vilib>:"Check if File or Folder Exists.vi"("path"=w992) -> ("file or folder exists?"=w988:bool, "dup path"=w989:path)  [unwired: 8 in, 1 out]
                            n523 = Not Equal?(x=w989, y=path "") -> (x != y?=w990:bool)
                            n524 = And(x=w988, y=w990) -> (x .and. y?=w987:bool)
                            n525 = case shown="False" w987 {
                              tunnel: [w1032 w1038] -> w1021
                              tunnel: [w1031 w1037] -> w1020
                              tunnel: w989 -> [_ w1035]
                              frame False {
                                n526 = Open/Create/Replace File(operation (0:open)=T7."open", access (0:read/write)=enum16{"read/write", "read-only", "write-only"}."read-only") -> (refnum out=w1032:refnum<file>, error out=w1031:errorcluster)  [unwired: 4 in, 1 out]
                              }
                              frame True {
                                n527 = Open/Create/Replace File(file path (use dialog)=w1035, operation (0:open)=T7."open", access (0:read/write)=enum16{"read/write", "read-only", "write-only"}."read-only") -> (refnum out=w1038:refnum<file>, error out=w1037:errorcluster)  [unwired: 3 in, 1 out]
                              }
                            }
                            n528 = Set File Position(offset (in bytes) (0)=i64 0, refnum=w1021, from (0:start)=enum16{"start", "end", "current"}."start", error in=w1020) -> (refnum out=w1017:refnum<file>, error out=w1016:errorcluster)
                            n529 = Read from Text File(file (use dialog)=w1017, error in=w1016) -> (refnum out=w1015:refnum<file>, error out=w1013:errorcluster)  [unwired: 2 in, 2 out]
                            n530 = Read from Text File(file (use dialog)=w1015, error in=w1013) -> (refnum out=w1014:refnum<file>, text=w985:string, error out=w1012:errorcluster)  [unwired: 2 in, 1 out]
                            n531 = Close File(refnum=w1014, error in=w1012) -> ()  [unwired: 2 out]
                            n532 = while {
                              tunnel: [w1046] -> w984 mode=indexing
                              shift-right: [w1040] -> _
                              shift-left: w985 -> [w1042]
                              stop <- w1045 stop-if-true
                              n533 = Match Pattern(string=w1042, regular expression="[\\t \\r \\n \\s]+ ") -> (before substring=w1041:string, after substring=w1040:string, offset past match=w1044:i32)  [unwired: 1 in, 1 out]
                              n534 = Less Than 0?(x=w1044) -> (x < 0?=w1045:bool)
                              n535 = Fract/Exp String To Number(string=w1041) -> (number=w1046:dbl)  [unwired: 3 in, 1 out]
                            }
                            n536 = Array Size(array=w984) -> (size(s)=w983:i32)
                            n537 = Index Array(array=w984, index=9) -> (element=w993:dbl)
                            n538 = Index Array(array=w984, index=0) -> (element=w986:dbl)
                            n539 = Index Array(array=w984, index=8) -> (element=w994:dbl)
                            n540 = Index Array(array=w984, index=1) -> (element=w1009:dbl)
                            n541 = Index Array(array=w984, index=2) -> (element=w1007:dbl)
                            n542 = Index Array(array=w984, index=7) -> (element=w997:dbl)
                            n543 = Index Array(array=w984, index=3) -> (element=w1005:dbl)
                            n544 = Index Array(array=w984, index=4) -> (element=w1003:dbl)
                            n545 = Index Array(array=w984, index=6) -> (element=w999:dbl)
                            n546 = Index Array(array=w984, index=5) -> (element=w1001:dbl)
                            n547 = Greater?(x=w983, y=10) -> (0:w981:bool)
                            n548 = local write "Y correction (pixel,P-CR Y)"(w994) -> ()
                            n549 = local write "counter finished"(w993) -> ()
                            n550 = case shown="True" w981 {
                              tunnel: w984 -> [_ w1028]
                              tunnel: [FALSE w1025] -> w980
                              tunnel: [TRUE w1024] -> w979
                              frame False {
                              }
                              frame True {
                                n551 = Index Array(array=w1028, index=11) -> (element=w1026:dbl)
                                n552 = Index Array(array=w1028, index=10) -> (element=w1027:dbl)
                                n553 = Greater Than 0?(x=w1027) -> (x > 0?=w1025:bool)
                                n554 = Greater Than 0?(x=w1026) -> (x > 0?=w1024:bool)
                              }
                            }
                            n555 = local write "slope_Rp"(w986) -> ()
                            n556 = local write "intercept_Rp"(w1009) -> ()
                            n557 = local write "R-squared_Rp"(w1007) -> ()
                            n558 = local write "average_Rp"(w1005) -> ()
                            n559 = local write "slope_Rp0s"(w1003) -> ()
                            n560 = local write "intercept_Rp0s"(w1001) -> ()
                            n561 = local write "R-squared_Rp0s"(w999) -> ()
                            n562 = local write "average_Rp0s"(w997) -> ()
                            n563 = local write "Vary pupil size?"(w979) -> ()
                            n564 = local write "2D cal?"(w980) -> ()
                          }
                        }
                      }
                      frame #1 {
                        # "slope_Rp intercept_Rp average_Rp slope_Rp0s intercept_Rp0s average_Rp0s Ycorrection"
                        n565 = local read "Y correction (pixel,P-CR Y)"() -> (w1048:dbl)
                        n566 = local read "slope_Rp0s"() -> (w1051:dbl)
                        n567 = local read "intercept_Rp0s"() -> (w1050:dbl)
                        n568 = local read "average_Rp0s"() -> (w1049:dbl)
                        n569 = local read "intercept_Rp"() -> (w1053:dbl)
                        n570 = local read "average_Rp"() -> (w1052:dbl)
                        n571 = local read "slope_Rp"() -> (w1054:dbl)
                        n572 = Bundle("slope_Rp"=w1054, "intercept_Rp"=w1053, "average_Rp"=w1052, "slope_Rp0s"=w1051, "intercept_Rp0s"=w1050, "average_Rp0s"=w1049, "Y correction (pixel,P-CR Y)"=w1048) -> (w1047:T1)  [unwired: 1 in]
                        n573 = local write "calib para"(w1047) -> ()
                      }
                    }
                  }
                  frame #1 {
                    w1057 = i64 0 ("Last Valid Frame 2")
                    w1055 = FALSE ("lost rec sweeps?")
                    w1059 = T6."Disabled and Grayed Out" ("Disabled")
                    n574 = local write "Last Valid Buffer"(w1057) -> ()
                    n575 = local write "Trial counter"(w1057) -> ()
                    n576 = local write "End session and save"(w1055) -> ()
                    n577 = local write "Buffer Overrun"(w1055) -> ()
                    n578 = local write "error flag"(errorcluster {"status"=FALSE, "code"=0, "source"=""} ("error constant")) -> ()
                    n579 = global write "Global 1.vi" "global stop"(w1055) -> ()
                    n580 = global write "Global 1.vi" "Eye tracker busy"(w1055) -> ()
                    n581 = property on="End session and save" class="Bool (strict)"("DisabledEnum"=T6."Enabled" ("Disabled")) -> ()  [unwired: 2 in, 2 out]
                    n582 = property on="Start session" class="Bool (strict)"("DisabledEnum"=w1059) -> ()  [unwired: 2 in, 2 out]
                    n583 = property on="stop program" class="Bool (strict)"("DisabledEnum"=w1059) -> ()  [unwired: 2 in, 2 out]
                  }
                  frame #2 {
                    # "create eye, avi and ai files"
                    # "send timing parameters and other global variables to the pulse generator and recording computer"
                    # "intiate UDP communication, send out the VS para and global variables, config variable state, create files"
                    n584 = stacked-sequence {
                      tunnel: [_ _ w1201] -> w1067
                      tunnel: [_ _ w1198] -> w1066
                      tunnel: [_ _ w1192] -> w1065
                      tunnel: [w1068 _ _] -> w1060
                      tunnel: [_ _ w1174] -> w1064
                      tunnel: [_ w1124 _] -> w1063
                      tunnel: [_ _ w1173] -> w1062
                      frame #0 {
                        n585 = case shown="True" "save eye data" {
                          tunnel: [_ w1076] -> w1068
                          frame False {
                          }
                          frame True {
                            n586 = while {
                              tunnel: [w1089] -> w1084
                              tunnel: [w1088] -> w1083
                              stop <- w1087 continue-if-true
                              n587 = stacked-sequence {
                                tunnel: [w1122 _] -> w1089
                                tunnel: [w1121 _] -> w1088
                                tunnel: [w1091 _] -> w1087
                                frame #0 {
                                (unwired) "/"
                                w1111 = "/"
                                n588 = local read "file subname"() -> (w1120:string)
                                n589 = Get Date/Time String() -> (date string=w1113:string)  [unwired: 3 in, 1 out]
                                n590 = local read "saving disk"() -> (w1092:string)
                                n591 = Match Pattern(string=w1113, regular expression=w1111) -> (before substring=w1110:string, after substring=w1112:string)  [unwired: 1 in, 2 out]
                                n592 = local read "ver"() -> (w1090:string)
                                n593 = Match Pattern(string=w1112, regular expression=w1111) -> (before substring=w1109:string, after substring=w1098:string)  [unwired: 1 in, 2 out]
                                n594 = Decimal String To Number(string=w1110) -> (number=w1104:i32)  [unwired: 2 in, 1 out]
                                n595 = Decimal String To Number(string=w1109) -> (number=w1101:i32)  [unwired: 2 in, 1 out]
                                n596 = String Subset(string=w1098, offset (0)=2) -> (substring=w1094:string)  [unwired: 1 in]
                                n597 = Number To Decimal String(number=w1104, width (-)=i16 2) -> (decimal integer string=w1107:string)
                                n598 = Number To Decimal String(number=w1101, width (-)=i16 2) -> (decimal integer string=w1103:string)
                                n599 = call <vilib>:"Space Constant.vi"() -> ("String"=w1106:string)
                                n600 = call <vilib>:"Space Constant.vi"() -> ("String"=w1102:string)
                                n601 = Search and Replace String(input string=w1107, search string=w1106, replace string="0" ("replace string (\"\")")) -> (result string=w1096:string)  [unwired: 5 in, 3 out]
                                n602 = Search and Replace String(input string=w1103, search string=w1102, replace string="0" ("replace string (\"\")")) -> (result string=w1095:string)  [unwired: 5 in, 3 out]
                                n603 = Concatenate Strings(w1096, w1095, w1094) -> (w1093:string)
                                n604 = Concatenate Strings(w1092, "eye\\" ("string"), w1090, "trk" ("string"), w1093, "_" ("string"), w1120, ".eye" ("string")) -> (w1115:string)
                                n605 = String To Path(string=w1115) -> (path=w1114:path)
                                n606 = call <vilib>:"Check if File or Folder Exists.vi"("path"=w1114) -> ("error out"=w1122:errorcluster, "file or folder exists?"=w1091:bool, "dup path"=w1121:path)  [unwired: 8 in]
                                "file or folder exists?" <- w1091
                                }
                                frame #1 {
                                n607 = Wait (ms)(milliseconds to wait=u32 100) -> ()  [unwired: 1 out]
                                }
                              }
                            }
                            "data path" <- w1083
                            "data path2" <- w1083
                            n608 = Open/Create/Replace File(file path (use dialog)=w1083, error in=w1084, operation (0:open)=T7."create", access (0:read/write)=enum16{"read/write", "read-only", "write-only"}."write-only") -> (refnum out=w1080:refnum<file>, error out=w1079:errorcluster)  [unwired: 2 in, 1 out]
                            n609 = Set File Position(offset (in bytes) (0)=i64 0, refnum=w1080, from (0:start)=enum16{"start", "end", "current"}."start", error in=w1079) -> (refnum out=w1077:refnum<file>, error out=w1075:errorcluster)
                            n610 = Initialize Array(sgl 0.0 ("element"), 4 ("dimension size")) -> (w1071:sgl[])
                            n611 = Write to Binary File(file (use dialog)=w1077, data=w1071, error in=w1075, 5:FALSE ("prepend array or string size? (T)"), 9:T8."little-endian" ("byte order (0:big-endian, network order)")) -> (refnum out=w1070:refnum<file>, error out=w1076:errorcluster)  [unwired: 1 in, 1 out]
                            n612 = local write "eye refnum out"(w1070) -> ()
                          }
                        }
                      }
                      frame #1 {
                        n613 = local read "Save Movie?"() -> (w1125:bool)
                        n614 = case shown="True" w1125 {
                          tunnel: [_ w1127] -> w1124
                          frame False {
                          }
                          frame True {
                            n615 = while {
                              tunnel: [w1137] -> w1126
                              shift-right: [w1134] -> w1132
                              shift-left: errorcluster {"status"=FALSE, "code"=0, "source"=""} ("error out") -> [w1135]
                              stop <- w1136 continue-if-true
                              n616 = stacked-sequence {
                                tunnel: [w1171 _] -> w1137
                                tunnel: [w1141 _] -> w1136
                                tunnel: [w1139 _] -> w1134
                                tunnel: w1135 -> [w1138 _]
                                frame #0 {
                                w1161 = "/"
                                n617 = Get Date/Time String() -> (date string=w1163:string)  [unwired: 3 in, 1 out]
                                n618 = local read "saving disk"() -> (w1142:string)
                                n619 = local read "file subname"() -> (w1164:string)
                                n620 = Match Pattern(string=w1163, regular expression=w1161) -> (before substring=w1160:string, after substring=w1162:string)  [unwired: 1 in, 2 out]
                                n621 = Match Pattern(string=w1162, regular expression=w1161) -> (before substring=w1159:string, after substring=w1148:string)  [unwired: 1 in, 2 out]
                                n622 = Decimal String To Number(string=w1160) -> (number=w1154:i32)  [unwired: 2 in, 1 out]
                                n623 = Decimal String To Number(string=w1159) -> (number=w1151:i32)  [unwired: 2 in, 1 out]
                                n624 = String Subset(string=w1148, offset (0)=2) -> (substring=w1144:string)  [unwired: 1 in]
                                n625 = Number To Decimal String(number=w1154, width (-)=i16 2) -> (decimal integer string=w1157:string)
                                n626 = local read "ver"() -> (w1140:string)
                                n627 = Number To Decimal String(number=w1151, width (-)=i16 2) -> (decimal integer string=w1153:string)
                                n628 = call <vilib>:"Space Constant.vi"() -> ("String"=w1156:string)
                                n629 = call <vilib>:"Space Constant.vi"() -> ("String"=w1152:string)
                                n630 = Search and Replace String(input string=w1157, search string=w1156, replace string="0" ("replace string (\"\")")) -> (result string=w1146:string)  [unwired: 5 in, 3 out]
                                n631 = Search and Replace String(input string=w1153, search string=w1152, replace string="0" ("replace string (\"\")")) -> (result string=w1145:string)  [unwired: 5 in, 3 out]
                                n632 = Concatenate Strings(w1146, w1145, w1144) -> (w1143:string)
                                n633 = Concatenate Strings(w1142, "avi\\" ("string"), w1140, "mov" ("string"), w1143, "_" ("string"), w1164, ".avi" ("string")) -> (w1166:string)
                                n634 = String To Path(string=w1166) -> (path=w1165:path)
                                n635 = call <vilib>:"Check if File or Folder Exists.vi"("error in (no error)"=w1138, "path"=w1165) -> ("error out"=w1139:errorcluster, "file or folder exists?"=w1141:bool, "dup path"=w1171:path)  [unwired: 7 in]
                                "file or folder exists? 3" <- w1141
                                }
                                frame #1 {
                                n636 = Wait (ms)(milliseconds to wait=u32 100) -> ()  [unwired: 1 out]
                                }
                              }
                            }
                            "move path2" <- w1126
                            n637 = local write "Movie Directory"(w1126) -> ()
                            n638 = local read "Save Frame Divisor"() -> (w1131:i32)
                            n639 = local read "Cam FR (f/s)"() -> (w1130:i32)
                            n640 = Quotient & Remainder(x=w1130, y=w1131) -> (floor(x/y)=w1129:i32)  [unwired: 1 out]
                            n641 = call "IMAQ AVI Create"("error in (no error)"=w1132, "Frames Per Second"=w1129, "AVI Path"=w1126) -> ("error out"=w1127:errorcluster, "Avi Refnum"=w1128:T3)  [unwired: 7 in]
                            n642 = local write "Avi Refnum"(w1128) -> ()
                          }
                        }
                      }
                      frame #2 {
                        w1199 = T12 0 items=["Grayscale (U8)", "Grayscale (I16)", "Grayscale (SGL)", "Complex (CSG)", "RGB (U32)", "HSL (U32)", "RGB (U64)"] ("Image Type")
                        w1179 = 1000 ("max queue size (-1, unlimited)")
                        w1203 = T12 4 items=["Grayscale (U8)", "Grayscale (I16)", "Grayscale (SGL)", "Complex (CSG)", "RGB (U32)", "HSL (U32)", "RGB (U64)"] ("Image Type")
                        n643 = call "IMAQ Create"("Image Name"="ForAvi", "Image Type"=w1203) -> ("New Image"=w1201:T2)  [unwired: 3 in, 1 out]
                        n644 = Initialize Array(sgl 0.0 ("element"), 3 ("dimension size")) -> (w1189:sgl[])
                        n645 = call "IMAQ Create"("Image Name"="Forqueue", "Image Type"=w1199) -> ("New Image"=w1178:T2)  [unwired: 3 in, 1 out]
                        n646 = Obtain Queue(max queue size (-1, unlimited)=w1179, name (unnamed)="processedframes", element data type=w1178) -> (queue out=w1180:refnum<queue>, error out=w1181:errorcluster)  [unwired: 2 in, 1 out]
                        n647 = Obtain Queue(max queue size (-1, unlimited)=w1179, name (unnamed)="eyeposition", element data type=w1189) -> (queue out=w1194:refnum<queue>, error out=w1186:errorcluster)  [unwired: 2 in, 1 out]
                        n648 = Obtain Queue(max queue size (-1, unlimited)=w1179, name (unnamed)="rawframes", element data type=w1178) -> (queue out=w1191:refnum<queue>, error out=w1188:errorcluster)  [unwired: 2 in, 1 out]
                        n649 = for {
                          N: w1179 -> [_]
                          tunnel: w1178 -> [w1206]
                          tunnel: w1194 -> [w1218]
                          tunnel: [w1217] -> w1193
                          tunnel: w1191 -> [w1216]
                          tunnel: [w1215] -> w1190
                          tunnel: w1189 -> [w1214]
                          shift-right: [w1212] -> w1187
                          shift-left: w1188 -> [w1213]
                          shift-right: [w1210] -> w1185
                          shift-left: w1186 -> [w1211]
                          shift-right: [w1208] -> w1176
                          shift-left: w1181 -> [w1209]
                          tunnel: w1180 -> [w1207]
                          tunnel: [w1205] -> w1177
                          n650 = Enqueue Element(queue=w1207, element=w1206, error in (no error)=w1209) -> (queue out=w1205:refnum<queue>, error out=w1208:errorcluster)  [unwired: 1 in, 1 out]
                          n651 = Enqueue Element(queue=w1218, element=w1214, error in (no error)=w1211) -> (queue out=w1217:refnum<queue>, error out=w1210:errorcluster)  [unwired: 1 in, 1 out]
                          n652 = Enqueue Element(queue=w1216, element=w1206, error in (no error)=w1213) -> (queue out=w1215:refnum<queue>, error out=w1212:errorcluster)  [unwired: 1 in, 1 out]
                        }
                        n653 = Flush Queue(queue=w1193, error in (no error)=w1185) -> (queue out=w1192:refnum<queue>, error out=w1183:errorcluster)  [unwired: 1 out]
                        n654 = Flush Queue(queue=w1177, error in (no error)=w1176) -> (queue out=w1174:refnum<queue>, error out=w1175:errorcluster)  [unwired: 1 out]
                        n655 = Flush Queue(queue=w1190, error in (no error)=w1187) -> (queue out=w1198:refnum<queue>, error out=w1184:errorcluster)  [unwired: 1 out]
                        n656 = Merge Errors(w1184, w1175, w1183) -> (w1173:errorcluster)
                      }
                    }
                    n657 = Merge Errors(w1060, w1063, w1062) -> (w1061:errorcluster)
                  }
                  frame #3 {
                    # "water hist"
                    # "frames each trial"
                    # "counter for eye data"
                    # "the loop of starting software"
                    # "1"
                    # "trial"
                    n658 = while {
                      tunnel: w1241 -> [w1265]
                      tunnel: w1240 -> [w1264]
                      tunnel: w1239 -> [w1263]
                      tunnel: w1238 -> [w1262]
                      tunnel: w1237 -> [w1261]
                      shift-right: [w1257] -> _
                      shift-left: 0 -> [w1258]
                      tunnel: [w1260] -> w1234
                      tunnel: [w1259] -> w1235
                      tunnel: w1232 -> [w1255]
                      tunnel: w1231 -> [w1254]
                      tunnel: w1230 -> [w1253]
                      tunnel: [w1252] -> w1229
                      tunnel: [w1251] -> w1228
                      shift-right: [w1249] -> w1225
                      shift-left: u64 0 -> [w1250]
                      shift-right: [w1247] -> w1226
                      shift-left: dbl[] [] -> [w1248]
                      shift-right: [w1246] -> w1223
                      shift-left: i32[] [] -> [w1245]
                      shift-right: [w1244] -> w1221
                      shift-left: w1222 -> [w1243]
                      tunnel: [w1242] -> w1220
                      stop <- w1256 stop-if-true
                      # "1 based\ntrial"
                      # "0 based\ntrial"
                      n659 = stacked-sequence {
                        seq-local: [w1273 _] -> [_ w1308]
                        seq-local: [w1267 _] -> [_ w1307]
                        tunnel: [_ w1317] -> w1244
                        tunnel: w1265 -> [_ w1316]
                        tunnel: w1264 -> [_ w1315]
                        tunnel: w1263 -> [_ w1293]
                        tunnel: w1262 -> [_ w1314]
                        tunnel: w1243 -> [w1270 w1313]
                        tunnel: w1261 -> [_ w1312]
                        tunnel: [_ w1311] -> w1260
                        tunnel: [_ w1310] -> w1259
                        tunnel: w1258 -> [w1274 w1309]
                        tunnel: [_ w1306] -> w1257
                        tunnel: [_ w1305] -> w1256
                        tunnel: w1255 -> [_ w1304]
                        tunnel: w1254 -> [_ w1303]
                        tunnel: w1253 -> [_ w1302]
                        tunnel: [_ w1301] -> w1252
                        tunnel: [_ w1300] -> w1251
                        tunnel: w1250 -> [_ w1299]
                        tunnel: [_ w1298] -> w1249
                        tunnel: w1248 -> [_ w1297]
                        tunnel: [_ w1296] -> w1247
                        tunnel: [_ w1295] -> w1246
                        tunnel: w1245 -> [_ w1294]
                        tunnel: [_ w1292] -> w1242
                        frame #0 {
                          n660 = local read "Buffer Overrun"() -> (w1271:bool)
                          n661 = local read "End session and save"() -> (w1272:bool)
                          n662 = local read "error flag"() -> (w1269:errorcluster)
                          n663 = Compound Arithmetic op=OR(w1272, w1271, w1270, w1269) -> (w1268:bool)
                          n664 = case shown="False" w1268 {
                            tunnel: w1274 -> [w1277 w1291]
                            tunnel: [w1276 w1291] -> w1273
                            tunnel: [w1275 TRUE] -> w1266
                            frame False {
                              n665 = stacked-sequence {
                                tunnel: w1277 -> [_ w1289]
                                tunnel: [_ w1288] -> w1276
                                tunnel: [w1278 _] -> w1275
                                frame #0 {
                                # "This initiates the trial\nChange here to integrate it into your rig\n(e.g. use the UDP line to receive start signal)"
                                # "Read trial start signal from the VStim program"
                                n666 = flat-sequence {
                                tunnel: [w1279] -> w1278
                                frame #0 {
                                n667 = while {
                                tunnel: [w1283] -> w1279
                                stop <- w1284 stop-if-true
                                n668 = global read "Global 1.vi" "Start one trial"() -> (w1282:bool)
                                n669 = shared-variable "Satoru-PC3\\Target variables.lvlib\\Start one trial RTNET"() -> (w1280:bool)  [unwired: 1 in, 1 out]
                                n670 = local read "End session and save"() -> (w1283:bool)
                                n671 = Wait (ms)(milliseconds to wait=u32 100) -> ()  [unwired: 1 out]
                                n672 = Or(x=w1282, y=w1280) -> (x .or. y?=w1281:bool)
                                n673 = Or(x=w1281, y=w1283) -> (x .or. y?=w1284:bool)
                                }
                                }
                                frame #1 {
                                w1286 = FALSE
                                n674 = shared-variable "Satoru-PC3\\Target variables.lvlib\\Start one trial RTNET"(w1286) -> ()  [unwired: 1 in, 1 out]
                                n675 = global write "Global 1.vi" "Eye tracker busy"(TRUE) -> ()
                                n676 = global write "Global 1.vi" "Start one trial"(w1286) -> ()
                                }
                                }
                                }
                                frame #1 {
                                n677 = Increment(x=w1289) -> (x+1=w1288:i32)
                                n678 = local write "Trial counter"(w1288) -> ()
                                }
                              }
                            }
                            frame True {
                            }
                          }
                          n679 = Or(x=w1266, y=w1268) -> (x .or. y?=w1267:bool)
                          "error IO" <- w1270
                        }
                        frame #1 {
                          n680 = case shown="False" w1307 {
                            selector: w1307 -> [_ w1765]
                            tunnel: [w1342 w1759] -> w1317
                            tunnel: w1316 -> [w1341 _]
                            tunnel: w1315 -> [w1340 _]
                            tunnel: w1293 -> [w1339 w1758]
                            tunnel: w1314 -> [w1338 w1759]
                            tunnel: w1313 -> [w1337 w1757]
                            tunnel: w1312 -> [w1336 _]
                            tunnel: [w1335 w1758] -> w1311
                            tunnel: [w1334 w1759] -> w1310
                            tunnel: w1309 -> [w1333 w1766]
                            tunnel: w1308 -> [w1332 _]
                            tunnel: [w1331 w1766] -> w1306
                            tunnel: [w1318 w1765] -> w1305
                            tunnel: w1304 -> [w1330 _]
                            tunnel: w1303 -> [w1329 w1764]
                            tunnel: w1302 -> [w1328 w1763]
                            tunnel: [w1327 w1764] -> w1301
                            tunnel: [w1326 w1763] -> w1300
                            tunnel: w1299 -> [w1325 w1762]
                            tunnel: [w1324 w1762] -> w1298
                            tunnel: w1297 -> [w1323 w1761]
                            tunnel: [w1322 w1761] -> w1296
                            tunnel: [w1321 w1760] -> w1295
                            tunnel: w1294 -> [w1320 w1760]
                            tunnel: [w1319 w1757] -> w1292
                            frame False {
                              n681 = stacked-sequence {
                                seq-local: [w1348 _ _ _] -> [_ w1406 w1703 _]
                                seq-local: [w1347 _ _ _] -> [_ w1407 _ _]
                                seq-local: [_ w1405 _ _] -> [_ _ w1702 _]
                                seq-local: [w1344 _ _ _] -> [_ w1384 _ _]
                                seq-local: [w1343 _ _ _] -> [_ w1383 _ _]
                                seq-local: [_ w1390 _ _] -> [_ _ w1699 _]
                                seq-local: [_ w1389 _ _] -> [_ _ w1698 _]
                                tunnel: w1341 -> [_ w1421 w1720 _]
                                tunnel: w1340 -> [_ w1420 w1719 _]
                                tunnel: w1336 -> [_ w1417 _ _]
                                tunnel: w1337 -> [_ w1400 w1715 _]
                                tunnel: [_ w1426 _ _] -> w1342
                                tunnel: w1339 -> [w1346 _ _ _]
                                tunnel: w1338 -> [w1345 _ _ _]
                                tunnel: [_ w1384 _ _] -> w1335
                                tunnel: [_ w1383 _ _] -> w1334
                                tunnel: w1333 -> [_ _ _ _]
                                tunnel: w1332 -> [_ _ _ w1755]
                                tunnel: [_ _ _ w1755] -> w1331
                                tunnel: w1330 -> [_ w1416 w1716 _]
                                tunnel: w1329 -> [_ w1414 _ _]
                                tunnel: w1328 -> [_ w1413 _ _]
                                tunnel: [_ _ w1697 _] -> w1327
                                tunnel: [_ _ w1696 _] -> w1326
                                tunnel: w1325 -> [_ w1411 _ _]
                                tunnel: [_ w1410 _ _] -> w1324
                                tunnel: w1323 -> [_ _ w1695 _]
                                tunnel: [_ _ w1694 _] -> w1322
                                tunnel: [_ w1409 _ _] -> w1321
                                tunnel: w1320 -> [_ w1408 _ _]
                                tunnel: [_ _ w1700 _] -> w1319
                                tunnel: [_ w1388 _ _] -> w1318
                                frame #0 {
                                n682 = flat-sequence {
                                tunnel: [w1350] -> w1348
                                tunnel: [w1349] -> w1347
                                tunnel: w1346 -> [w1371]
                                tunnel: w1345 -> [w1370]
                                tunnel: [w1369] -> w1344
                                tunnel: [w1368] -> w1343
                                frame #0 {
                                n683 = local read "Pixel value offset"() -> (w1352:cluster{"Ch 1":u8, "Ch 2":u8})
                                n684 = local read "Gain offset"() -> (w1356:dbl)
                                n685 = local read "Gain (dB)"() -> (w1355:dbl)
                                n686 = local read "Region of interest"() -> (w1358:i32[])
                                n687 = Add(x=w1355, y=w1356) -> (x+y=w1354:dbl)
                                n688 = Bundle("Gain (dB)"=w1355, w1354) -> (w1353:cluster{"Gain (dB)":dbl, dbl})  [unwired: 1 in]
                                n689 = local read "Cam FR (f/s)"() -> (w1359:i32)
                                n690 = call "Start Video-reinitiate imaq.vi"("Offset"=w1352, "Gain(dB)"=w1353, "Camera Fr"=w1359, "Trigger Type"=enum16{"Internal", "External"}."External", "Region of interest"=w1358) -> ("error out"=w1349:errorcluster, "Frame Buffers Out"=w1351:T2[], "IMAQ Session Out"=w1350:refnum<k11>)  [unwired: 4 in]
                                n691 = local write "Frame Buffers Out"(w1351) -> ()
                                }
                                frame #1 {
                                # "This is to initialize the number of expected frames per trial. \nIf it is set too short, the eye tracking may terminate too early."
                                n692 = local read "Cam FR (f/s)"() -> (w1362:i32)
                                n693 = Divide(x="Max expected duration of eye tracking per trial (ms)", y=sgl 1000.0) -> (x/y=w1365:sgl)
                                n694 = Multiply(x=w1365, y=w1362) -> (x*y=w1363:sgl)
                                n695 = property on="eye trace" class="WFGraph (strict)"("XScale.Maximum"=w1365) -> ()  [unwired: 2 in, 2 out]
                                n696 = To Unsigned Long Integer(number=w1363) -> (unsigned 32bit integer=w1360:u32)
                                n697 = local write "processed frames"(w1360) -> ()
                                n698 = local write "frame/trial"(w1360) -> ()
                                }
                                frame #2 {
                                w1366 = TRUE
                                # "Send ready signal to VS"
                                n699 = local read "talk to VS"() -> (w1367:bool)
                                n700 = case shown="False" w1367 {
                                tunnel: w1371 -> [_ w1380]
                                tunnel: w1370 -> [_ w1379]
                                tunnel: [_ w1375] -> w1369
                                tunnel: [_ w1374] -> w1368
                                frame False {
                                }
                                frame True {
                                # "When fitting this to your rig, change here (e.g. send out TTL\ninstead of an UDP packet)"
                                n701 = local read "R Port com"() -> (w1376:u16)
                                n702 = local read "Remote IP_VS"() -> (w1373:string)
                                n703 = String To IP(1:w1373) -> (0:w1377:u32)
                                n704 = UDP Write(address=w1377, port or service name=w1376, connection ID=w1380, data in="presentVS", 8:w1379, 9:25000 ("timeout ms (25000)")) -> (error out=w1374:errorcluster, 3:w1375:refnum<k16>)
                                }
                                }
                                n705 = global write "Global 1.vi" "Camera ready"(w1366) -> ()
                                n706 = shared-variable "Satoru-PC3\\Target variables.lvlib\\Camera ready RTNET"(w1366) -> ()  [unwired: 1 in, 1 out]
                                }
                                frame #3 {
                                n707 = shared-variable "Satoru-PC3\\Target variables.lvlib\\Camera ready RTNET"() -> (→"Camera ready RTNET":bool)  [unwired: 1 in, 1 out]
                                }
                                }
                                }
                                frame #1 {
                                w1418 = u32 0
                                # "This loop receives stop variable from main program to end pulse generation"
                                # "Buffer size in ms"
                                # "loop of Image acquisition and eye tracking."
                                # "frame \ncounter"
                                # "Camera"
                                # "frames when parameters are changed"
                                # "availalbe frame#"
                                # "grabbed frame#"
                                n708 = local read "Time for eye tracking after VS (>1ms)"() -> (w1392:dbl)
                                n709 = local read "Cam FR (f/s)"() -> (w1401:i32)
                                n710 = call "Pulse generator2.vi"("Framedur"=10000, "duty cylcle"="duty cylcle of the pulses", "error in"=w1400, "Counter freq"=w1401) -> ("error out"=w1402:errorcluster, "# of pulses"=→"# of pulses":i32)
                                n711 = local read "Cam FR (f/s)"() -> (w1395:i32)
                                n712 = node-c288(i64 200 ("Period")) -> (w1424:T9)  [unwired: 3 in]
                                n713 = Divide(x=w1392, y=1000.0) -> (x/y=w1394:dbl)
                                n714 = Multiply(x=w1394, y=w1395) -> (x*y=w1396:dbl)
                                n715 = To Unsigned Long Integer(number=w1396) -> (unsigned 32bit integer=w1397:u32)
                                n716 = timed-loop {
                                timing: w1424 -> [_]
                                timing-out: [_] -> w1423
                                tunnel: w1421 -> [w1527]
                                tunnel: w1420 -> [w1526]
                                shift-right: [w1523] -> _
                                shift-left: w1400 -> [w1519]
                                tunnel: w1416 -> [w1520]
                                stop <- w1516 stop-if-true
                                n717 = node-c288() -> ()  [unwired: 1 in, 1 out]
                                n718 = Get Queue Status(queue=w1527, error in (no error)=w1519) -> (error out=w1525:errorcluster, # elements in queue=→"# in Q1":i32)  [unwired: 7 out]
                                n719 = Get Queue Status(queue=w1520, error in (no error)=w1519) -> (error out=w1518:errorcluster, # elements in queue=→"# in Q3":i32)  [unwired: 7 out]
                                n720 = Get Queue Status(queue=w1526, error in (no error)=w1519) -> (error out=w1524:errorcluster, # elements in queue=→"# in Q2":i32)  [unwired: 7 out]
                                n721 = global read "Global 1.vi" "global stop"() -> (w1516:bool)
                                n722 = Merge Errors(w1518, w1525, w1524) -> (w1523:errorcluster)
                                n723 = node-c288() -> ()  [unwired: 1 in, 1 out]
                                }
                                n724 = while {
                                tunnel: w1397 -> [w1460]
                                shift-right: [w1456] -> w1391
                                shift-left: FALSE -> [w1457]
                                stop <- w1458 stop-if-true
                                n725 = shared-variable "Satoru-PC3\\Target variables.lvlib\\Camera stop RTNET"() -> (w1453:bool)  [unwired: 1 in, 1 out]
                                n726 = global read "Global 1.vi" "camera stop"() -> (w1455:bool)
                                n727 = Or(x=w1455, y=w1453) -> (x .or. y?=w1454:bool)
                                n728 = case shown="False" w1454 {
                                tunnel: w1460 -> [_ w1467]
                                tunnel: [w1462 TRUE] -> w1456
                                tunnel: w1457 -> [w1462 _]
                                frame False {
                                n729 = shared-variable "Satoru-PC3\\Target variables.lvlib\\Camera ready RTNET"() -> (w1461:bool)  [unwired: 1 in, 1 out]
                                n730 = local write "Camera ready RTNET"(w1461) -> ()
                                }
                                frame True {
                                w1463 = FALSE
                                n731 = shared-variable "Satoru-PC3\\Target variables.lvlib\\Camera stop RTNET"(w1463) -> ()  [unwired: 1 in, 1 out]
                                n732 = local read "aquired frames"() -> (w1465:u64)
                                n733 = Add(x=w1465, y=w1467) -> (x+y=w1464:u64)
                                n734 = global write "Global 1.vi" "camera stop"(w1463) -> ()
                                n735 = local write "frame/trial"(w1464) -> ()
                                }
                                }
                                n736 = global read "Global 1.vi" "global stop"() -> (w1459:bool)
                                n737 = Or(x=w1459, y=w1456) -> (x .or. y?=w1458:bool)
                                }
                                n738 = node-c288(w1423) -> ()  [unwired: 1 out]
                                n739 = while {
                                tunnel: w1416 -> [w1480]
                                shift-right: [w1471] -> w1415
                                shift-left: w1400 -> [w1474]
                                shift-right: [w1473] -> _
                                shift-left: w1418 -> [w1476]
                                tunnel: w1417 -> [w1475]
                                stop <- w1469 stop-if-true
                                n740 = Dequeue Element(queue=w1480, timeout in ms (-1)=5, error in (no error)=w1474) -> (element=w1478:T2, timed out?=w1479:bool, error out=w1477:errorcluster)  [unwired: 1 out]
                                n741 = case shown="False" w1479 {
                                tunnel: w1478 -> [w1488 _]
                                tunnel: w1477 -> [w1487 w1515]
                                tunnel: w1476 -> [w1486 w1513]
                                tunnel: [w1485 w1513] -> w1473
                                tunnel: [w1484 w1515] -> w1471
                                tunnel: w1475 -> [w1483 _]
                                tunnel: [FALSE w1514] -> w1468
                                frame False {
                                n742 = Quotient & Remainder(x=w1486, y="Disp Frame Divisor") -> (x-y*floor(x/y)=w1492:u32)  [unwired: 1 out]
                                n743 = Equal To 0?(x=w1492) -> (x = 0?=w1491:bool)
                                n744 = case shown="True" w1491 {
                                tunnel: w1488 -> [_ w1511]
                                frame False {
                                }
                                frame True {
                                n745 = local write "Image"(w1511) -> ()
                                }
                                }
                                n746 = local read "Include Overlay to Movie?"() -> (w1494:bool)
                                n747 = local read "Save Movie?"() -> (w1489:bool)
                                n748 = local read "Avi Refnum"() -> (w1490:T3)
                                n749 = case shown="True" w1489 {
                                tunnel: w1490 -> [_ w1501]
                                tunnel: w1483 -> [_ w1500]
                                tunnel: w1488 -> [_ w1499]
                                tunnel: w1487 -> [w1495 w1498]
                                tunnel: [w1495 w1497] -> w1484
                                tunnel: w1494 -> [_ w1496]
                                frame False {
                                }
                                frame True {
                                n750 = case shown="True" w1496 {
                                tunnel: [w1504 w1510] -> w1503
                                tunnel: [w1505 w1509] -> w1502
                                tunnel: w1500 -> [_ w1508]
                                tunnel: w1499 -> [w1504 w1507]
                                tunnel: w1498 -> [w1505 w1506]
                                frame False {
                                }
                                frame True {
                                n751 = call "IMAQ Merge Overlay"("error in (no error)"=w1506, "Image Dst"=w1508, "Image Src"=w1507) -> ("error out"=w1509:errorcluster, "Image Dst Out"=w1510:T2)  [unwired: 7 in]
                                }
                                }
                                n752 = call "IMAQ AVI Write Frame"("error in (no error)"=w1502, "Image"=w1503, "Avi Refnum"=w1501) -> ("error out"=w1497:errorcluster)  [unwired: 7 in, 1 out]
                                }
                                }
                                n753 = Increment(x=w1486) -> (x+1=w1485:u32)
                                }
                                frame True {
                                n754 = local read "processed frames"() -> (w1512:i32)
                                n755 = Equal?(x=w1513, y=w1512) -> (x = y?=w1514:bool)
                                }
                                }
                                n756 = local read "error flag"() -> (w1472:errorcluster)
                                n757 = local read "Buffer Overrun"() -> (w1470:bool)
                                n758 = Compound Arithmetic op=OR(w1472, w1468, w1471, w1470) -> (w1469:bool)
                                }
                                n759 = while {
                                tunnel: w1406 -> [w1446]
                                shift-right: [w1442] -> w1405
                                shift-left: w1407 -> [w1445]
                                tunnel: w1421 -> [w1444]
                                i -> [w1429]
                                stop <- w1438 stop-if-true
                                # "image acquisition"
                                # "extract frames"
                                n760 = call <vilib>:"IMAQ Extract Buffer.vi"("error in (no error)"=w1445, "Buffer to extract"=w1429, "IMAQ Session In"=w1446) -> ("error out"=w1431:errorcluster, "Buffer Number"=w1433:i32, "Image Out"=w1436:T2)  [unwired: 3 in, 3 out]
                                n761 = Not Equal?(x=w1433, y=w1429) -> (x != y?=w1440:bool)
                                n762 = local write "Buffer Overrun"(w1440) -> ()
                                n763 = case shown="True" w1440 {
                                tunnel: w1431 -> [w1447 w1449]
                                tunnel: [w1447 w1448] -> w1437
                                frame False {
                                }
                                frame True {
                                w1450 = u16 0 items=["no dialog", "OK message", "continue or stop message"] ("type of dialog (OK msg:1)")
                                # "User defined error 6500"
                                n764 = call <vilib>:"General Error Handler.vi"("[error code] (0)"=6500 ("error code (no error:0)"), "[error source] (\" \")"="Video Monitor" ("[error source] (\" \")"), "type of dialog (OK msg:1)"=w1450, "error in (no error)"=w1449) -> ("error out"=w1448:errorcluster)  [unwired: 7 in, 4 out]
                                }
                                }
                                n765 = local write "Last Valid Buffer"(w1433) -> ()
                                n766 = call "IMAQ Clear Overlay"("error in (no error)"=w1437, "Image"=w1436) -> ("error out"=w1434:errorcluster, "Image Out"=w1435:T2)  [unwired: 8 in]
                                n767 = Enqueue Element(queue=w1444, element=w1435, error in (no error)=w1434) -> (timed out?=→"queue timed out?":bool, error out=w1442:errorcluster)  [unwired: 1 in, 1 out]
                                "error flag" <- w1442
                                n768 = Increment(x=w1429) -> (x+1=w1430:i32)
                                "aquired frames" <- w1430
                                n769 = local read "frame/trial"() -> (w1439:i32)
                                n770 = Greater Or Equal?(x=w1430, y=w1439) -> (x >= y?=w1443:bool)
                                n771 = Unbundle By Name(w1442) -> ("status"=w1441:bool)
                                n772 = Compound Arithmetic op=OR(w1441, w1443, w1440) -> (w1438:bool)
                                }
                                n773 = Not(x=w1391) -> (.not. x?=w1388:bool)
                                n774 = local read "Remote IP_VS"() -> (w1386:string)
                                n775 = String To IP(1:w1386) -> (0:w1385:u32)
                                n776 = local read "R Port data"() -> (w1387:u16)
                                n777 = while {
                                tunnel: w1421 -> [w1557]
                                tunnel: w1420 -> [w1555]
                                shift-right: [w1546] -> w1425
                                shift-left: w1400 -> [w1554]
                                shift-right: [w1551] -> w1427
                                shift-left: dbl[][] [] -> [w1552]
                                shift-right: [w1535] -> _
                                shift-left: w1418 -> [w1548]
                                tunnel: w1416 -> [w1545]
                                shift-right: [w1540] -> w1389
                                shift-left: w1413 -> [w1542]
                                tunnel: w1414 -> [w1543]
                                tunnel: [w1541] -> w1390
                                tunnel: w1387 -> [w1538]
                                tunnel: w1385 -> [w1537]
                                stop <- w1534 stop-if-true
                                n778 = Dequeue Element(queue=w1557, timeout in ms (-1)=5, error in (no error)=w1554) -> (element=w1556:T2, timed out?=w1549:bool, error out=w1553:errorcluster)  [unwired: 1 out]
                                n779 = case shown="False" w1549 {
                                tunnel: w1556 -> [w1603 _]
                                tunnel: w1555 -> [w1602 _]
                                tunnel: w1553 -> [w1601 w1648]
                                tunnel: w1552 -> [w1600 w1647]
                                tunnel: [w1599 w1647] -> w1551
                                tunnel: w1548 -> [w1583 w1646]
                                tunnel: [w1595 w1648] -> w1546
                                tunnel: [w1597 w1646] -> w1535
                                tunnel: w1545 -> [w1590 _]
                                tunnel: w1543 -> [w1587 w1645]
                                tunnel: w1542 -> [w1582 w1644]
                                tunnel: [w1586 w1645] -> w1541
                                tunnel: [w1585 w1644] -> w1540
                                tunnel: w1538 -> [w1581 _]
                                tunnel: w1537 -> [w1580 _]
                                frame False {
                                w1572 = TRUE
                                # "fit pupil&CR, calculate eye position"
                                # "each row contain one parameter"
                                # "fit pupil and corneal reflection"
                                n780 = local read "CR Bottom"() -> (w1611:i32)
                                n781 = local read "CR Right"() -> (w1610:i32)
                                n782 = local read "CR Top"() -> (w1609:i32)
                                n783 = local read "CR Direction to keep"() -> (w1613:enum16{"Above", "Below"})
                                n784 = local read "Points to show"() -> (w1565:enum16{"All points", "Fit points"})
                                n785 = local read "CR Left"() -> (w1608:i32)
                                n786 = Build Array(w1608, w1609, w1610, w1611) -> (w1606:i32[])
                                n787 = local read "CR Fit type"() -> (w1614:enum16{"Circle", "Ellipse"})
                                n788 = local read "CR Subsampling"() -> (w1615:i32)
                                n789 = local read "CR Threshold"() -> (w1612:u8)
                                n790 = local read "Display Overlay"() -> (w1578:bool)
                                n791 = call "Process Pupil or Cornea ReflectionPerc.vi"("Image In"=w1603, "ROI"=w1606, "Threshold"=w1612, "Direction to keep"=w1613, "error in (no error)"=w1601, "Display"=w1572, "Fit type"=w1614, "Subsampling"=w1615, "Color"=u32 6618880, "use % thresh"=FALSE, "Display Overlay"=w1578, "Points to show"=w1565) -> ("Image out"=w1577:T2, "x position"=w1604:dbl, "y position"=w1605:dbl, "error out"=w1574:errorcluster)  [unwired: 3 in, 1 out]
                                n792 = local read "P Right"() -> (w1624:i32)
                                n793 = local read "P Left"() -> (w1625:i32)
                                n794 = local read "Disp trace Divisor"() -> (w1592:i32)
                                n795 = local read "P Top"() -> (w1616:i32)
                                n796 = local read "P Direction to keep"() -> (w1570:enum16{"Above", "Below"})
                                n797 = local read "P Threshold"() -> (w1571:u8)
                                n798 = local read "P Bottom"() -> (w1617:i32)
                                n799 = local read "use % thresh"() -> (w1569:bool)
                                n800 = local read "P Fit type"() -> (w1563:enum16{"Circle", "Ellipse"})
                                n801 = local read "P Subsampling"() -> (w1564:i32)
                                n802 = Build Array(w1625, w1616, w1624, w1617) -> (w1573:i32[])
                                n803 = Quotient & Remainder(x=w1583, y=w1592) -> (x-y*floor(x/y)=w1594:u32)  [unwired: 1 out]
                                n804 = Decrement(x=w1592) -> (x-1=w1591:i32)
                                n805 = call "Process Pupil Reflection_ovalROI2.vi"("Image In"=w1577, "Threshold"=w1571, "Direction to keep"=w1570, "error in (no error)"=w1574, "Display"=w1572, "Fit type"=w1563, "Global Rectangle"=w1573, "Subsampling"=w1564, "Color"=u32 16777215, "use % thresh"=w1569, "Display Overlay"=w1578, "Points to show"=w1565) -> ("Image out"=w1576:T2, "x position"=w1568:dbl, "y position"=w1567:dbl, "diameter"=w1566:dbl, "error out"=w1575:errorcluster)  [unwired: 3 in]
                                n806 = Equal?(x=w1594, y=w1591) -> (x = y?=w1593:bool)
                                n807 = Build Array(w1568, w1604, w1566, w1567, w1605) -> (w1618:dbl[])
                                n808 = Enqueue Element(queue=w1590, element=w1576, error in (no error)=w1575) -> (timed out?=→"queue timed out? 3":bool, error out=w1589:errorcluster)  [unwired: 1 in, 1 out]
                                n809 = local read "Eye Y offset(deg)"() -> (w1623:dbl)
                                n810 = local read "conversion factor"() -> (w1620:cluster{"x":dbl, "y":dbl})
                                n811 = local read "calib para"() -> (w1619:T1)
                                n812 = local read "Vary pupil size?"() -> (w1622:bool)
                                n813 = local read "talk to VS"() -> (w1559:bool)
                                n814 = local read "2D cal?"() -> (w1621:bool)
                                n815 = call "degree conversion-eyecursor.vi"("xdegcorr"=sgl 0.0, "Change pupil size?"=w1622, "1D or 2D cal?"=w1621, "Y manual offset (degrees)"=w1623, "calib para"=w1619, "pixel input"=w1618, "conversion factor(mm/pixel)"=w1620) -> ("angle output"=w1562:dbl[])  [unwired: 3 in]
                                n816 = Enqueue Element(queue=w1602, element=w1562, error in (no error)=w1575) -> (timed out?=→"queue timed out? 2":bool, error out=w1596:errorcluster)  [unwired: 1 in, 1 out]
                                n817 = Build Array (concatenate)(w1600, w1562) -> (w1599:dbl[][])
                                n818 = case shown="True" w1593 {
                                tunnel: w1599 -> [_ w1638]
                                frame False {
                                }
                                frame True {
                                n819 = local read "Cam FR (f/s)"() -> (w1641:i32)
                                n820 = Transpose 2D Array(2D array=w1638) -> (transposed array=w1639:dbl[][])
                                n821 = Reciprocal(x=w1641) -> (1/x=w1640:dbl)
                                n822 = Bundle(0, w1640, w1639) -> (w1642:cluster{i32, dbl, dbl[][]})  [unwired: 1 in]
                                n823 = local write "eye trace"(w1642) -> ()
                                }
                                }
                                n824 = Index Array(array=w1562, index=0) -> (element=w1560:dbl)
                                n825 = case shown="False" w1559 {
                                tunnel: w1587 -> [_ w1637]
                                tunnel: [_ w1636] -> w1586
                                tunnel: [_ w1635] -> w1585
                                tunnel: w1582 -> [_ w1630]
                                tunnel: w1581 -> [_ w1629]
                                tunnel: w1580 -> [_ w1628]
                                tunnel: w1562 -> [_ w1627]
                                frame False {
                                }
                                frame True {
                                n826 = To Single Precision Float(number=w1627) -> (single precision float=w1632:sgl[])
                                n827 = call <vilib>:"Space Constant.vi"() -> ("String"=w1633:string)
                                n828 = Array To Spreadsheet String(delimiter (Tab)=w1633, array=w1632, 3:"%.3f" ("format string")) -> (spreadsheet string=w1631:string)
                                n829 = UDP Write(address=w1628, port or service name=w1629, connection ID=w1637, data in=w1631, 8:w1630) -> (error out=w1635:errorcluster, 3:w1636:refnum<k16>)  [unwired: 1 in]
                                }
                                }
                                n830 = Increment(x=w1583) -> (x+1=w1597:u32)
                                n831 = Merge Errors(w1596, w1589) -> (w1595:errorcluster)
                                n832 = shared-variable "My Computer\\Network variables.lvlib\\x degree out"(w1560) -> ()  [unwired: 1 in, 1 out]
                                }
                                frame True {
                                }
                                }
                                n833 = local read "Buffer Overrun"() -> (w1544:bool)
                                n834 = local read "frame/trial"() -> (w1539:i32)
                                n835 = local read "error flag"() -> (w1547:errorcluster)
                                n836 = Greater Or Equal?(x=w1535, y=w1539) -> (x >= y?=w1536:bool)
                                n837 = Compound Arithmetic op=OR(w1536, w1547, w1546, w1544) -> (w1534:bool)
                                n838 = case shown="True" w1536 {
                                tunnel: w1535 -> [_ w1558]
                                frame False {
                                }
                                frame True {
                                n839 = local write "processed frames"(w1558) -> ()
                                }
                                }
                                n840 = global write "Global 1.vi" "global stop"(w1534) -> ()
                                n841 = shared-variable "Satoru-PC3\\Target variables.lvlib\\Terminate RTNET"(w1534) -> ()  [unwired: 1 in, 1 out]
                                }
                                n842 = stacked-sequence {
                                tunnel: w1420 -> [w1671]
                                tunnel: w1400 -> [w1670]
                                tunnel: [w1668] -> w1419
                                frame #0 {
                                # "retrieve data"
                                # "frame counter"
                                n843 = while {
                                tunnel: w1671 -> [w1685]
                                shift-right: [w1677] -> w1668
                                shift-left: w1670 -> [w1683]
                                tunnel: [w1682] -> _
                                shift-right: [w1675] -> _
                                shift-left: u32 0 -> [w1679]
                                stop <- w1672 stop-if-true
                                n844 = Dequeue Element(queue=w1685, timeout in ms (-1)=5, error in (no error)=w1683) -> (queue out=w1682:refnum<queue>, element=w1684:sgl[], timed out?=w1680:bool, error out=w1677:errorcluster)
                                n845 = case shown="False" w1680 {
                                tunnel: w1684 -> [w1688 _]
                                tunnel: w1679 -> [w1689 w1691]
                                tunnel: [w1690 w1691] -> w1675
                                frame False {
                                n846 = Array Subset(array=w1688, index=0, length=2) -> ()  [unwired: 1 out]
                                n847 = Increment(x=w1689) -> (x+1=w1690:u32)
                                }
                                frame True {
                                }
                                }
                                n848 = local read "frame/trial"() -> (w1674:i32)
                                n849 = global read "Global 1.vi" "global stop"() -> (w1673:bool)
                                n850 = local read "error flag"() -> (w1676:errorcluster)
                                n851 = Greater Or Equal?(x=w1675, y=w1674) -> (x >= y?=w1678:bool)
                                n852 = Compound Arithmetic op=OR(w1678, w1677, w1676, w1673) -> (w1672:bool)
                                }
                                }
                                }
                                n853 = local read "save eye data"() -> (w1428:bool)
                                n854 = case shown="True" w1428 {
                                tunnel: w1425 -> [w1651 w1667]
                                tunnel: [w1651 w1666] -> w1404
                                tunnel: w1427 -> [_ w1661]
                                tunnel: w1411 -> [w1650 w1659]
                                tunnel: [w1650 w1658] -> w1410
                                tunnel: [w1649 w1653] -> w1409
                                tunnel: w1408 -> [w1649 w1652]
                                frame False {
                                }
                                frame True {
                                n855 = Array Size(array=w1661) -> (size(s)=w1656:i32[])
                                n856 = local read "eye refnum out"() -> (w1662:refnum<file>)
                                n857 = Multiply Array Elements(1:w1656) -> (0:w1660:i32)
                                n858 = Index Array(array=w1656, index=0) -> (element=w1654:i32)
                                n859 = To Single Precision Float(number=w1661) -> (single precision float=w1663:sgl[][])
                                n860 = Compound Arithmetic op=ADD(w1660, w1659, u64 2 ("value")) -> (w1658:u64)
                                n861 = Build Array (concatenate)(w1652, w1654) -> (w1653:i32[])
                                n862 = Write to Binary File(file (use dialog)=w1662, data=w1663, error in=w1667, 5:TRUE ("prepend array or string size? (T)"), 9:T8."little-endian" ("byte order (0:big-endian, network order)")) -> (error out=w1666:errorcluster)  [unwired: 1 in, 2 out]
                                }
                                }
                                n863 = Merge Errors(w1415, w1404, w1419, w1402) -> (w1426:errorcluster)
                                }
                                frame #2 {
                                w1692 = FALSE ("stop flag")
                                n864 = property class="IMAQ"(reference=w1703, error in=w1702) -> (reference out=w1709:refnum<k11>, error out=w1711:errorcluster, "Frame Count"=w1705:u32)
                                n865 = property class="IMAQ"(reference=w1709, error in=w1711) -> (reference out=w1708:refnum<k11>, error out=w1710:errorcluster, "Last Valid Frame"=w1707:u32)
                                n866 = Increment(x=w1707) -> (x+1=w1706:u32)
                                n867 = Not Equal?(x=w1706, y=w1705) -> ()  [unwired: 1 out]
                                n868 = local read "Frame Buffers Out"() -> (w1712:T2[])
                                n869 = local read "Cam FR (f/s)"() -> (w1704:i32)
                                n870 = call "Stop Video-reinitiate imaq.vi"("Camera Fr"=w1704, "Trigger Type"=enum16{"Internal", "External"}."Internal", "error in"=w1710, "Frame Buffers In"=w1712, "IMAQ Session In"=w1708) -> ("error out"=w1701:errorcluster)  [unwired: 6 in]
                                n871 = Flush Queue(queue=w1716, error in (no error)=w1715) -> (error out=w1714:errorcluster)  [unwired: 2 out]
                                n872 = Flush Queue(queue=w1720, error in (no error)=w1715) -> (error out=w1718:errorcluster)  [unwired: 2 out]
                                n873 = Flush Queue(queue=w1719, error in (no error)=w1715) -> (error out=w1717:errorcluster)  [unwired: 2 out]
                                n874 = Merge Errors(w1701, w1714, w1718, w1717) -> (w1700:errorcluster)
                                n875 = global write "Global 1.vi" "Camera ready"(w1692) -> ()
                                n876 = global write "Global 1.vi" "global stop"(w1692) -> ()
                                n877 = case shown="False" FALSE {
                                tunnel: w1699 -> [w1722 w1739]
                                tunnel: w1698 -> [w1723 w1738]
                                tunnel: [w1722 w1737] -> w1697
                                tunnel: [w1723 w1729] -> w1696
                                tunnel: w1695 -> [w1721 w1727]
                                tunnel: [w1721 w1726] -> w1694
                                frame False {
                                }
                                frame True {
                                # "This is for receiving VS position. Not necessary for simply tracking the eye."
                                n878 = local read "R Port data"() -> (w1736:u16)
                                n879 = UDP Read(connection ID=w1739, timeout ms (25000)=1000, 8:w1738) -> (data out=w1728:string, error out=w1725:errorcluster, 3:w1737:refnum<k16>, 4:w1735:u16)  [unwired: 1 in, 1 out]
                                n880 = String Length(string=w1728) -> (length=w1734:i32)
                                n881 = Equal?(x=w1735, y=w1736) -> (x = y?=w1732:bool)
                                n882 = call "no timeout error.vi"("error in (no error)"=w1725) -> ("error out"=w1724:errorcluster)
                                n883 = Not Equal To 0?(x=w1734) -> (x != 0?=w1733:bool)
                                n884 = And(x=w1733, y=w1732) -> (x .and. y?=w1730:bool)
                                n885 = case shown="True" w1730 {
                                tunnel: w1724 -> [w1741 w1750]
                                tunnel: [w1741 w1745] -> w1729
                                tunnel: w1728 -> [_ w1749]
                                tunnel: w1727 -> [w1740 w1748]
                                tunnel: [w1740 w1747] -> w1726
                                frame False {
                                }
                                frame True {
                                (unwired) FALSE ("data includes array or string size? (T)")
                                w1746 = -1.0 ("default value 2")
                                n886 = Scan From String(format string="%f %f ", input string=w1749, initial scan location=u32 0, error in=w1750, default 1=w1746, default 2=w1746) -> (error out=w1745:errorcluster, output 1=w1744:dbl, output 2=w1743:dbl)  [unwired: 2 out]
                                n887 = Build Array(w1744, w1743) -> (w1742:dbl[])
                                n888 = Build Array (concatenate)(w1748, w1742) -> (w1747:dbl[])
                                }
                                }
                                }
                                }
                                }
                                frame #3 {
                                n889 = global write "Global 1.vi" "Eye tracker busy"(FALSE) -> ()
                                n890 = Wait (ms)(milliseconds to wait=u32 500) -> ()  [unwired: 1 out]
                                }
                              }
                            }
                            frame True {
                              n891 = global write "Global 1.vi" "Eye tracker busy"(FALSE) -> ()
                            }
                          }
                        }
                      }
                    }
                    n892 = Merge Errors(w1221) -> (w1233:errorcluster)
                  }
                  frame #4 {
                    n893 = stacked-sequence {
                      seq-local: [w1781 _] -> [_ w1796]
                      tunnel: w1774 -> [w1776 _]
                      tunnel: w1773 -> [w1786 _]
                      tunnel: w1772 -> [w1785 _]
                      tunnel: w1771 -> [w1784 _]
                      tunnel: w1770 -> [_ w1795]
                      tunnel: w1769 -> [_ w1794]
                      tunnel: w1768 -> [_ w1793]
                      tunnel: w1767 -> [w1780 _]
                      frame #0 {
                        w1778 = TRUE ("force destroy? (F)")
                        n894 = local read "Save Movie?"() -> (w1777:bool)
                        n895 = case shown="True" w1777 {
                          tunnel: w1776 -> [w1788 w1791]
                          tunnel: [w1788 w1790] -> w1775
                          frame False {
                          }
                          frame True {
                            n896 = local read "Avi Refnum"() -> (w1789:T3)
                            n897 = call "IMAQ AVI Close"("error in (no error)"=w1791, "Avi Refnum"=w1789) -> ("error out"=w1790:errorcluster)  [unwired: 9 in]
                          }
                        }
                        n898 = Release Queue(queue=w1786, force destroy? (F)=w1778, error in (no error)=w1775) -> (error out=w1787:errorcluster)  [unwired: 2 out]
                        n899 = Release Queue(queue=w1785, force destroy? (F)=w1778, error in (no error)=w1775) -> (error out=w1782:errorcluster)  [unwired: 2 out]
                        n900 = call "IMAQ Dispose"("Image"=w1784, "error in (no error)"=w1775) -> ("error out"=w1783:errorcluster)  [unwired: 4 in]
                        n901 = Release Queue(queue=w1780, force destroy? (F)=w1778, error in (no error)=w1775) -> (error out=w1779:errorcluster)  [unwired: 2 out]
                        n902 = Merge Errors(w1779, w1783, w1787, w1782) -> (w1781:errorcluster)
                      }
                      frame #1 {
                        # "The first four elements are (1,\"number of trials\",\"number of elements for eye position info\",0).\nThis is followed by the eye position info for every trial:\n     - The first two elements for each trial are (\"number of frames for the trial\",3)\n     - The above two elements are followed by (x, y, radius) for every frame \n     - Thus, \"number of frames for the trial\" * 3 + 2 is the total number of elements for each trial\nThis is then followed by an array of numbers of frames for each trial. This number is obviously redundant info.\nThis is then followed by the size of the parameters and the actual parameters."
                        # "terminate image acquisition and eye tracking, and save remaining parameters"
                        n903 = local read "save eye data"() -> (w1797:bool)
                        n904 = case shown="True" w1797 {
                          tunnel: w1796 -> [w1798 w1875]
                          tunnel: [w1798 w1847] -> w1792
                          tunnel: w1795 -> [_ w1799]
                          tunnel: w1794 -> [_ w1826]
                          tunnel: w1793 -> [_ w1829]
                          frame False {
                          }
                          frame True {
                            w1801 = FALSE ("prepend array or string size? (T)")
                            w1802 = T8."little-endian" ("byte order (0:big-endian, network order)")
                            # "Conversion factor 2\ncalib para 7\nEye Y offset\nCam FR\n2D cal\nvary pupil size\nsave movie\nTime for eye tracking\ninput cal para from file\ntalk to VS\n18\n3\n1"
                            # "data: each line is one frame"
                            # "save the size of the data array and the size of the stimulation parameters,\n which are required to retrieve the data and para"
                            n905 = local read "Last Valid Buffer"() -> (w1857:i32)
                            n906 = local read "Trial counter"() -> (w1856:u32)
                            n907 = local read "eye refnum out"() -> (w1848:refnum<file>)
                            n908 = Build Array(w1857, w1856) -> (w1855:u32[])
                            n909 = local read "P Direction to keep"() -> (w1868:enum16{"Above", "Below"})
                            n910 = local read "CR Direction to keep"() -> (w1860:enum16{"Above", "Below"})
                            n911 = local read "CR Subsampling"() -> (w1858:i32)
                            n912 = local read "P Subsampling"() -> (w1866:i32)
                            n913 = local read "CR Threshold"() -> (w1861:u8)
                            n914 = local read "P Threshold"() -> (w1869:u8)
                            n915 = local read "CR Fit type"() -> (w1859:enum16{"Circle", "Ellipse"})
                            n916 = local read "CR Bottom"() -> (w1863:i32)
                            n917 = local read "P Bottom"() -> (w1871:i32)
                            n918 = local read "P Fit type"() -> (w1867:enum16{"Circle", "Ellipse"})
                            n919 = local read "CR Top"() -> (w1865:i32)
                            n920 = local read "CR Right"() -> (w1862:i32)
                            n921 = local read "CR Left"() -> (w1864:i32)
                            n922 = local read "P Left"() -> (w1872:i32)
                            n923 = local read "P Top"() -> (w1873:i32)
                            n924 = local read "P Right"() -> (w1870:i32)
                            n925 = Set File Position(offset (in bytes) (0)=i64 0, refnum=w1848, from (0:start)=enum16{"start", "end", "current"}."current", error in=w1875) -> (refnum out=w1812:refnum<file>, error out=w1813:errorcluster)
                            n926 = Build Array (concatenate)(w1873, w1872, w1871, w1870, w1869, w1868, w1867, w1866, w1865, w1864, w1863, w1862, w1861, w1860, w1859, w1858, w1855) -> (w1837:u32[])
                            n927 = To Single Precision Float(number=w1826) -> (single precision float=w1827:sgl[])
                            n928 = Write to Binary File(file (use dialog)=w1812, data=w1827, error in=w1813, 5:w1801, 9:w1802) -> (refnum out=w1823:refnum<file>, error out=w1825:errorcluster)  [unwired: 1 in, 1 out]
                            n929 = Array Size(array=w1826) -> (size(s)=w1800:i32)
                            n930 = local read "input cal para from file?"() -> (w1853:bool)
                            n931 = Build Array(1 ("element"), w1800, w1799) -> (w1815:u64[])
                            n932 = To Single Precision Float(number=w1815) -> (single precision float=w1803:sgl[])
                            n933 = local read "Save Movie?"() -> (w1854:bool)
                            n934 = local read "conversion factor"() -> (w1889:cluster{"x":dbl, "y":dbl})
                            n935 = local read "Vary pupil size?"() -> (w1886:bool)
                            n936 = local read "calib para"() -> (w1888:T1)
                            n937 = local read "Cam FR (f/s)"() -> (w1882:i32)
                            n938 = local read "Eye Y offset(deg)"() -> (w1883:dbl)
                            n939 = local read "2D cal?"() -> (w1887:bool)
                            n940 = local read "Time for eye tracking after VS (>1ms)"() -> (w1814:dbl)
                            n941 = local read "talk to VS"() -> (w1849:bool)
                            n942 = Boolean To (0,1)(Boolean=w1887) -> (0, 1=w1881:i16)
                            n943 = Boolean To (0,1)(Boolean=w1886) -> (0, 1=w1880:i16)
                            n944 = Boolean To (0,1)(Boolean=w1854) -> (0, 1=w1878:i16)
                            n945 = Cluster To Array(cluster=w1888) -> (array=w1884:dbl[])
                            n946 = Cluster To Array(cluster=w1889) -> (array=w1885:dbl[])
                            n947 = Build Array(w1853, w1849) -> (w1874:bool[])
                            n948 = Array Size(array=w1829) -> (size(s)=w1831:i32)
                            n949 = case shown="True" w1854 {
                              tunnel: ["" w1894] -> w1852
                              frame False {
                              }
                              frame True {
                                n950 = local read "Movie Directory"() -> (w1895:path)
                                n951 = Path To String(path=w1895) -> (string=w1894:string)
                              }
                            }
                            n952 = Boolean To (0,1)(Boolean=w1874) -> (0, 1=w1834:i16[])
                            n953 = To Single Precision Float(number=w1831) -> (single precision float=w1830:sgl)
                            n954 = Build Array (concatenate)(w1814, w1834) -> (w1835:dbl[])
                            n955 = To Single Precision Float(number=w1829) -> (single precision float=w1828:sgl[])
                            n956 = local read "queue timed out?"() -> (w1844:bool)
                            n957 = local read "queue timed out? 2"() -> (w1843:bool)
                            n958 = local read "Buffer Overrun"() -> (w1845:bool)
                            n959 = case shown="True" w1853 {
                              tunnel: ["" w1891] -> w1851
                              frame False {
                              }
                              frame True {
                                n960 = local read "calib para file to load"() -> (w1892:path)
                                n961 = Path To String(path=w1892) -> (string=w1891:string)
                              }
                            }
                            n962 = Boolean To (0,1)(Boolean=w1844) -> (0, 1=w1841:i16)
                            n963 = Boolean To (0,1)(Boolean=w1845) -> (0, 1=w1842:i16)
                            n964 = Boolean To (0,1)(Boolean=w1843) -> (0, 1=w1840:i16)
                            n965 = Build Array(w1842, w1841, w1840) -> (w1836:i16[])
                            n966 = Concatenate Strings(w1852, "&" ("string"), w1851) -> (w1850:string)
                            n967 = String To Byte Array(string=w1850) -> (unsigned byte array=w1838:u8[])
                            n968 = Array Size(array=w1838) -> (size(s)=w1839:i32)
                            n969 = Build Array (concatenate)(w1885, w1884, w1883, w1882, w1881, w1880, w1878, w1835, w1837, w1836, w1839, w1838) -> (w1879:dbl[])
                            n970 = To Single Precision Float(number=w1879) -> (single precision float=w1819:sgl[])
                            n971 = Array Size(array=w1819) -> (size(s)=w1821:i32)
                            n972 = To Single Precision Float(number=w1821) -> (single precision float=w1820:sgl)
                            n973 = Write to Binary File(file (use dialog)=w1823, data=w1820, error in=w1825, 9:w1802) -> (refnum out=w1822:refnum<file>, error out=w1824:errorcluster)  [unwired: 2 in, 1 out]
                            n974 = Write to Binary File(file (use dialog)=w1822, data=w1819, error in=w1824, 5:w1801, 9:w1802) -> (refnum out=w1818:refnum<file>, error out=w1817:errorcluster)  [unwired: 1 in, 1 out]
                            n975 = Write to Binary File(file (use dialog)=w1818, data=w1830, error in=w1817, 5:w1801, 9:w1802) -> (refnum out=w1833:refnum<file>, error out=w1832:errorcluster)  [unwired: 1 in, 1 out]
                            n976 = Write to Binary File(file (use dialog)=w1833, data=w1828, error in=w1832, 5:w1801, 9:w1802) -> (refnum out=w1811:refnum<file>, error out=w1810:errorcluster)  [unwired: 1 in, 1 out]
                            n977 = Set File Position(offset (in bytes) (0)=i64 0, refnum=w1811, from (0:start)=enum16{"start", "end", "current"}."start", error in=w1810) -> (refnum out=w1807:refnum<file>, error out=w1805:errorcluster)
                            n978 = Write to Binary File(file (use dialog)=w1807, data=w1803, error in=w1805, 5:w1801, 9:w1802) -> (refnum out=w1806:refnum<file>, error out=w1804:errorcluster)  [unwired: 1 in, 1 out]
                            n979 = Close File(refnum=w1806, error in=w1804) -> (error out=w1847:errorcluster)  [unwired: 1 out]
                          }
                        }
                        n980 = call <vilib>:"General Error Handler.vi"("error in (no error)"=w1792) -> ()  [unwired: 2 in, 13 out]
                      }
                    }
                  }
                  frame #5 {
                    w1898 = T6."Enabled" ("Disabled")
                    w1896 = FALSE ("stop meausre")
                    n981 = local write "End session and save"(w1896) -> ()
                    n982 = local write "Start session"(w1896) -> ()
                    n983 = global write "Global 1.vi" "global stop"(w1896) -> ()
                    n984 = global write "Global 1.vi" "Start one trial"(w1896) -> ()
                    n985 = local write "stop program"(w1896) -> ()
                    n986 = global write "Global 1.vi" "Eye tracker busy"(w1896) -> ()
                    n987 = property on="Start session" class="Bool (strict)"("DisabledEnum"=w1898) -> ()  [unwired: 2 in, 2 out]
                    n988 = property on="stop program" class="Bool (strict)"("DisabledEnum"=w1898) -> ()  [unwired: 2 in, 2 out]
                    n989 = property on="End session and save" class="Bool (strict)"("DisabledEnum"=T6."Disabled and Grayed Out" ("Disabled")) -> ()  [unwired: 2 in, 2 out]
                  }
                }
              }
            }
          }
        }
        frame #2 {
          n990 = local write "stop program"(FALSE ("stop meausre")) -> ()
          n991 = property on="End session and save" class="Bool (strict)"("DisabledEnum"=T6."Enabled" ("Disabled")) -> ()  [unwired: 2 in, 2 out]
        }
      }
      n992 = local read "talk to VS"() -> (w925:bool)
      n993 = case shown="True" w925 {
        tunnel: [w1906 w1908] -> w928
        tunnel: w935 -> [w1905 w1908]
        tunnel: w934 -> [w1904 _]
        tunnel: w931 -> [w1903 _]
        tunnel: w930 -> [w1902 w1907]
        tunnel: [w1901 w1907] -> w929
        frame True {
          n994 = UDP Close(connection ID=w1903, 8:w1902) -> (error out=w1901:errorcluster)  [unwired: 1 out]
          n995 = UDP Close(connection ID=w1904, 8:w1905) -> (error out=w1906:errorcluster)  [unwired: 1 out]
        }
        frame False {
        }
      }
      n996 = Merge Errors(w928, w929, w926) -> (w927:errorcluster)
      n997 = call <vilib>:"General Error Handler.vi"("error in (no error)"=w927) -> ()  [unwired: 2 in, 13 out]
    }
    frame "delete last acq" {
      w1927 = TRUE ("confirm (F)")
      n998 = local read "data path"() -> (w1926:path)
      n999 = call <vilib>:"Check if File or Folder Exists.vi"("path"=w1926) -> ("error out"=w1925:errorcluster, "file or folder exists?"=w1924:bool)  [unwired: 8 in, 1 out]
      "eye file exist" <- w1924
      n1000 = case shown="True" w1924 {
        tunnel: [w1933 w1937] -> w1920
        tunnel: w1927 -> [_ w1936]
        tunnel: w1926 -> [_ w1935]
        tunnel: w1925 -> [w1933 w1934]
        frame False {
        }
        frame True {
          n1001 = Delete(path (use dialog)=w1935, confirm (F)=w1936, error in=w1934) -> (error out=w1937:errorcluster)  [unwired: 2 in, 2 out]
        }
      }
      n1002 = local read "Movie Directory"() -> (w1923:path)
      n1003 = call <vilib>:"Check if File or Folder Exists.vi"("error in (no error)"=w1920, "path"=w1923) -> ("error out"=w1921:errorcluster, "file or folder exists?"=w1922:bool)  [unwired: 7 in, 1 out]
      "avi file exist" <- w1922
      n1004 = case shown="True" w1922 {
        tunnel: w1927 -> [_ w1932]
        tunnel: [w1928 w1931] -> w1919
        tunnel: w1923 -> [_ w1930]
        tunnel: w1921 -> [w1928 w1929]
        frame False {
        }
        frame True {
          n1005 = Delete(path (use dialog)=w1930, confirm (F)=w1932, error in=w1929) -> (error out=w1931:errorcluster)  [unwired: 2 in, 2 out]
        }
      }
      "error out" <- w1919
    }
  }
